vi "DCSource.vi"() -> ()   [LabVIEW 2014]
uses:
  <vilib>/Instr/_visa.llb/VISA Set IO Buffer Mask.ctl
  <vilib>/Utility/miscctls.llb/LVRowAndColumnTypeDef.ctl
  <vilib>/Instr/_visa.llb/VISA Configure Serial Port (Instr).vi
  <vilib>/Utility/file.llb/Write To Spreadsheet File (string).vi
  <vilib>/Utility/file.llb/Read From Spreadsheet File (string).vi
panel:
  in  "shutDown":bool
  in  "本机表格":string[][](table)=[["0.000"], ["0.000"], ["0.000"], ["0.000"], ["0.000"], ["0.000"], ["0.000"], ["0.000"]]
  in  "result_Tab":enum32{"输出控制", "电能校验", "误差计算", "潜动启动", "无"}(tab)
  in  "outPut_form":string[][](table)=[["0.000"], ["0.000"], ["0.000"], ["0.000"], ["0.000"], ["0.000"], ["0.000"], ["0.000"]]
  in  "电能显示表":string[][](table)=[["", "", "", "", "", ""], ["", "", "", "", "", ""], ["", "", "", "", "", ""], ["", "", "", "", "", ""], ["", "", "", "", "", ""], ["", "", "", "", "", ""], ["", "", "", "", "", ""], ["", "", "", "", "", ""], ["", "", "", "", "", ""], ["", "", "", "", "", ""], ["", "", "", "", "", ""], ["", "", "", "", "", ""], ["", "", "", "", "", ""], ["", "", "", "", "", ""], ["", "", "", "", "", ""]]
  in  "误差显示表":string[][](table)=[["", "", "", "", "", ""], ["", "", "", "", "", ""], ["", "", "", "", "", ""], ["", "", "", "", "", ""], ["", "", "", "", "", ""], ["", "", "", "", "", ""], ["", "", "", "", "", ""], ["", "", "", "", "", ""], ["", "", "", "", "", ""], ["", "", "", "", "", ""], ["", "", "", "", "", ""], ["", "", "", "", "", ""], ["", "", "", "", "", ""], ["", "", "", "", "", ""], ["", "", "", "", "", ""]]
  out "单点显示表":string[][](table)
  in  "All输出":cluster{"A停止":bool, "A启动":bool}
  in  "超时记录":bool[](array[boolean])=[FALSE, FALSE, FALSE]
  out "当前功率":dbl
  out "表3已等待时间":dbl
  out "表2已等待时间":dbl
  out "表1已等待时间":dbl
  in  "表1OK":bool
  in  "表2OK":bool
  in  "表3OK":bool
  in  "已用秒数":dbl
  out "计时状态":bool
  out "E检定行":i32
  out "下一点":bool
  out "UI行数":i32
  out "E行数":i32
  in  "UI当前行":i32
  out "检定状态":bool
  in  "E当前行":i32
  in  "软键盘":bool caption="Ia停止"
  out "提示信息":bool
  in  "控制选项卡":T1(tab)
  in  "vOptios_Tab":enum32{"电流1", "电流2", "电流3", "电流4"}(tab)
  in  "I操作":T2
  in  "I纹波":sgl caption="电流纹波(A)" min=0 max=20 format="%.3f"
  out "I状态":bool caption="状态"
  in  "I幅值":sgl=1.0 caption="电流(A)" min=0 max=200 format="%.3f"
  in  "I档位":u32(ring)=85 caption="电流档位" items=["自动"=85, "0.02A"=0, "0.2A"=1, "1A"=2, "5A"=3, "10A"=4, "20A"=5, "30A"=6, "60A"=7, "200A"=8]
  in  "UB_outPut_ctl":T3
  out "UB_status":bool caption="状态"
  in  "UB_Pos":u32(ring)=85 caption="电流档位" items=["自动"=85, "0.01V"=0, "0.1V"=1, "0.5"=2, "5V"=3]
  in  "UB_amplitude":sgl=48.0 caption="电流(A)" min=0 max=10 format="%.3f"
  in  "UB_ripple":sgl caption="电流纹波(A)" min=0 max=100 format="%.3f"
  in  "IB_outPut_ctl":T4
  in  "IB_pos":u32(ring)=85 caption="电流档位" items=["自动"=85, "0.01V"=0, "0.1V"=1, "0.5V"=2, "5V"=3]
  in  "IB_amplitude":sgl=1.0 caption="电流(A)" min=0 max=200 format="%.3f"
  out "IB_status":bool caption="状态"
  in  "IB_ripple":sgl caption="电流纹波(A)" min=0 max=20 format="%.3f"
  in  "UC_outPut_ctl":T5
  in  "UC_ripple":sgl caption="电流纹波(A)" min=0 max=20 format="%.3f"
  out "UC_status":bool caption="状态"
  in  "UC_amplitude":sgl=1.0 caption="电流(A)" min=0 max=200 format="%.3f"
  in  "UC_pos":u32(ring)=85 caption="电流档位" items=["自动"=85, "0.01"=0, "0.1V"=1, "0.5V"=2, "5V"=3]
  in  "U档位":u32(ring)=85 caption="电压档位" items=["自动"=85, "65V"=0, "250V"=1, "500V"=2, "750V"=3, "1000V"=4]
  in  "U频率":sgl caption="纹波频率(Hz)" min=0 max=1000 format="%.3f"
  in  "U纹波":sgl caption="电压纹波(V)" min=0 max=100 format="%.3f"
  out "U状态":bool caption="状态"
  in  "U幅值":sgl=48.0 caption="电压(V)" min=0 max=1000 format="%.3f"
  in  "U操作":T6
  in  "电能检定通道":u16(ring) items=["电流 1", "电流 2", "电流 3", "电流 4"]
  in  "表3超时时间":string
  in  "表2超时时间":string
  in  "表1超时时间":string
  in  "E检定表格":string[][](table)=[["", "", "", "", ""], ["", "", "", "", ""], ["", "", "", "", ""], ["", "", "", "", ""], ["", "", "", "", ""]]
  in  "E检定操作":T7
  in  "E检定参数":T8={"额定电压"=48.0, "U检定点"=100.0, "标定电流"=20.0, "I检定点"=100.0, "允许误差"=0.5, "I检定点 2"=10.0} {"标定电流" min=0 max=200; "额定电压" min=0 max=1000}
  in  "E增删改清":T9
  in  "表1":bool
  in  "表2":bool
  in  "表3":bool
  in  "增加等待时间(s)":dbl=4.0
  in  "UI检定表格":string[][](table) caption="默认电压误差表"
  in  "UI检定操作":T10
  in  "UI增删改清":T9
  in  "UI检定参数":T11={"检定项目"=0, "额定电压"=48.0, "电压检定点"=20.0, "标定电流"=100.0, "电流检定点"=100.0, "误差限值"=0.5, "电压纹波"=0.0, "电流纹波"=0.0, "纹波频率"=0.0} {"标定电流" min=0 max=200; "额定电压" min=0 max=1000; "检定项目" items=["电压误差", "电流误差", "纹波试验"]}
  in  "误差电流通道":u16(ring) items=["电流 1", "电流 2", "电流 3", "电流 4"]
  in  "潜启电流通道":u16(ring) items=["电流 1", "电流 2", "电流 3", "电流 4"]
  in  "潜动起动":T12={"已用时间"="", "开始试验"=FALSE, "测试时间"=20.0, "标定电流"=20.0, "额定电压"=48.0, "试验项目"=0, "U检定点"=130.0, "I检定点"=0.1, "脉冲数"=1} {"脉冲数" max=200; "试验项目" items=["潜动试验", "起动试验"]; "额定电压" min=0 max=1000; "标定电流" min=0 max=200; "测试时间" format="%#.3f"}
  out "试验结果":string[](array[string])
  in  "生成报表":bool
  in  "报表名称":string
  in  "报表选项":u16(ring) items=["按时间命名", "自定义命名"]
  in  "小信号变比(A/1mv)":cluster{"电流2":sgl, "电流3":sgl, "电流4":sgl}={"电流2"=200.0, "电流3"=200.0, "电流4"=200.0}
  in  "脉冲输入口":u8(ring) items=["端口1", "端口2", "端口3"]
  in  "本机表参数":cluster{"有功常数":i32, "无功常数":i32, "输出类型":i32}={"有功常数"=200, "无功常数"=200, "输出类型"=0} {"输出类型" items=["有功脉冲", "无功脉冲"]}
  in  "电能表参数":T13={"有功常数"=200, "无功常数"=200, "校验圈数"=5, "校验类型"=0, "S值计算次数"=12, "S值计算方法"=0} {"S值计算方法" items=["平均值法"]; "校验类型" items=["有功脉冲", "无功脉冲"]}
  in  "本机表设置":cluster{"本机读参数":bool, "本机写参数":bool}
  in  "电能表设置":cluster{"表读参数":bool, "表写参数":bool}
  in  "串口信息":T14={"串口号"="COM1", "波特率"=57600, "校验位"=0, "停止位"=10} {"停止位" items=["1位"=10, "1.5位"=15, "2位"=20]; "校验位" items=["无校验", "奇校验", "偶检验"]; "波特率" items=["9600"=9600, "38400"=38400, "57600"=57600]}
  in  "串口连接":bool
  out "串口灯":bool
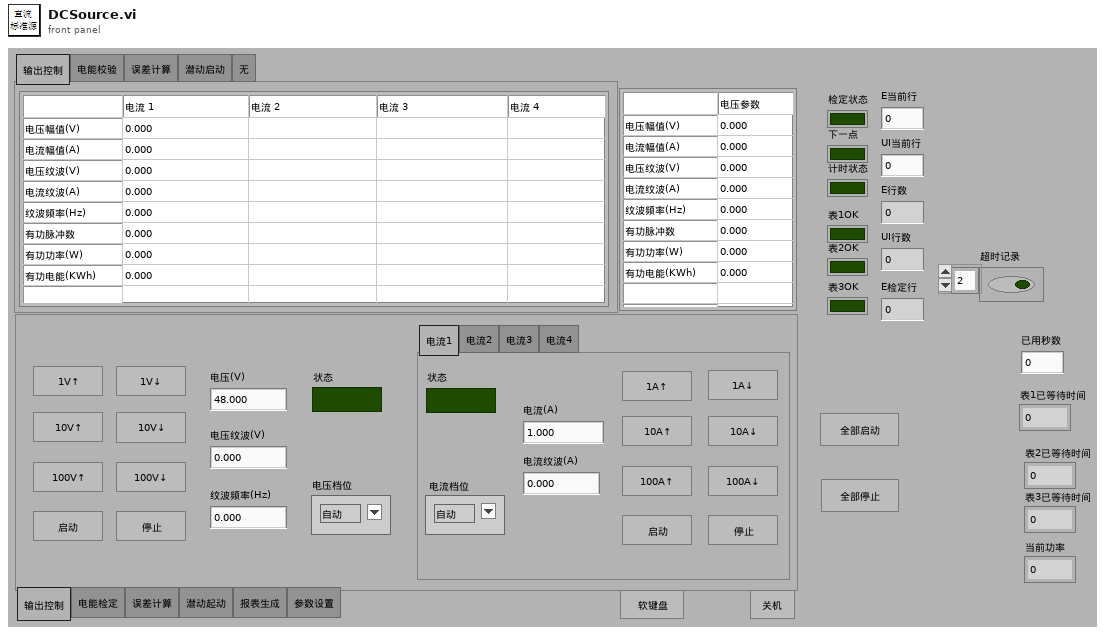
[diagram p1: front panel]
types:
  T1 = enum32{"输出控制", "电能检定", "误差计算", "潜动起动", "报表生成", "参数设置"}
  T2 = cluster{"ISub100":bool, "IAdd100":bool, "ISub10":bool, "IAdd10":bool, "ISub1":bool, "IAdd1":bool, "I启动":bool, "I停止":bool}
  T3 = cluster{"UB_outPut_start":bool, "UB_outPut_stop":bool}
  T4 = cluster{"IB_outPut_start":bool, "IB_outPut_stop":bool}
  T5 = cluster{"UC_outPut_stop":bool, "UC_outPut_start":bool}
  T6 = cluster{"UAdd10":bool, "USub10":bool, "UAdd100":bool, "USub100":bool, "U停止":bool, "USub1":bool, "UAdd1":bool, "U启动":bool}
  T7 = cluster{"开始检定":bool, "单点检定":bool, "保存方案":bool, "导入方案":bool}
  T8 = cluster{"额定电压":sgl, "U检定点":sgl, "标定电流":sgl, "I检定点":sgl, "允许误差":sgl, "I检定点 2":sgl}
  T9 = cluster{"插入":bool, "编辑":bool, "删除":bool, "清空":bool}
  T10 = cluster{"输出开关":bool, "保存方案":bool, "导入方案":bool, "计算误差":bool}
  T11 = cluster{"检定项目":u16, "额定电压":sgl, "电压检定点":sgl, "标定电流":sgl, "电流检定点":sgl, "误差限值":sgl, "电压纹波":sgl, "电流纹波":sgl, "纹波频率":sgl}
  T12 = cluster{"已用时间":string, "开始试验":bool, "测试时间":dbl, "标定电流":sgl, "额定电压":sgl, "试验项目":u16, "U检定点":sgl, "I检定点":sgl, "脉冲数":u32}
  T13 = cluster{"有功常数":i32, "无功常数":i32, "校验圈数":i32, "校验类型":i32, "S值计算次数":i32, "S值计算方法":i32}
  T14 = cluster{"串口号":refnum<visa-resource-name>, "波特率":u32, "校验位":u8, "停止位":u16}
  T15 = cluster{"串口号":refnum<visa-resource-name>, "波特率":u16, "校验位":u16, "停止位":u16}
  T16 = cluster{"有功功率":sgl, "有功电能":sgl, "有功脉冲":u64, "标准偏差值":sgl[], "电能误差":sgl[], "脉冲输入功率":sgl[], "脉冲电能累计":sgl[], "输入脉冲数":sgl[]}
  T17 = typedef "LVRowAndColumnTypeDef.ctl" = cluster{"Row":i32, "Column":i32}
  T18 = cluster{"有功常数":i32, "无功常数":i32, "校验圈数":i32, "校验类型":i32, "S值计算次数":i32, "S值计算方法":i32}[]
  T19 = enum8{"Enabled", "Disabled", "Disabled and Grayed Out"}
  T20 = typedef "VISA Set IO Buffer Mask.ctl" = u16
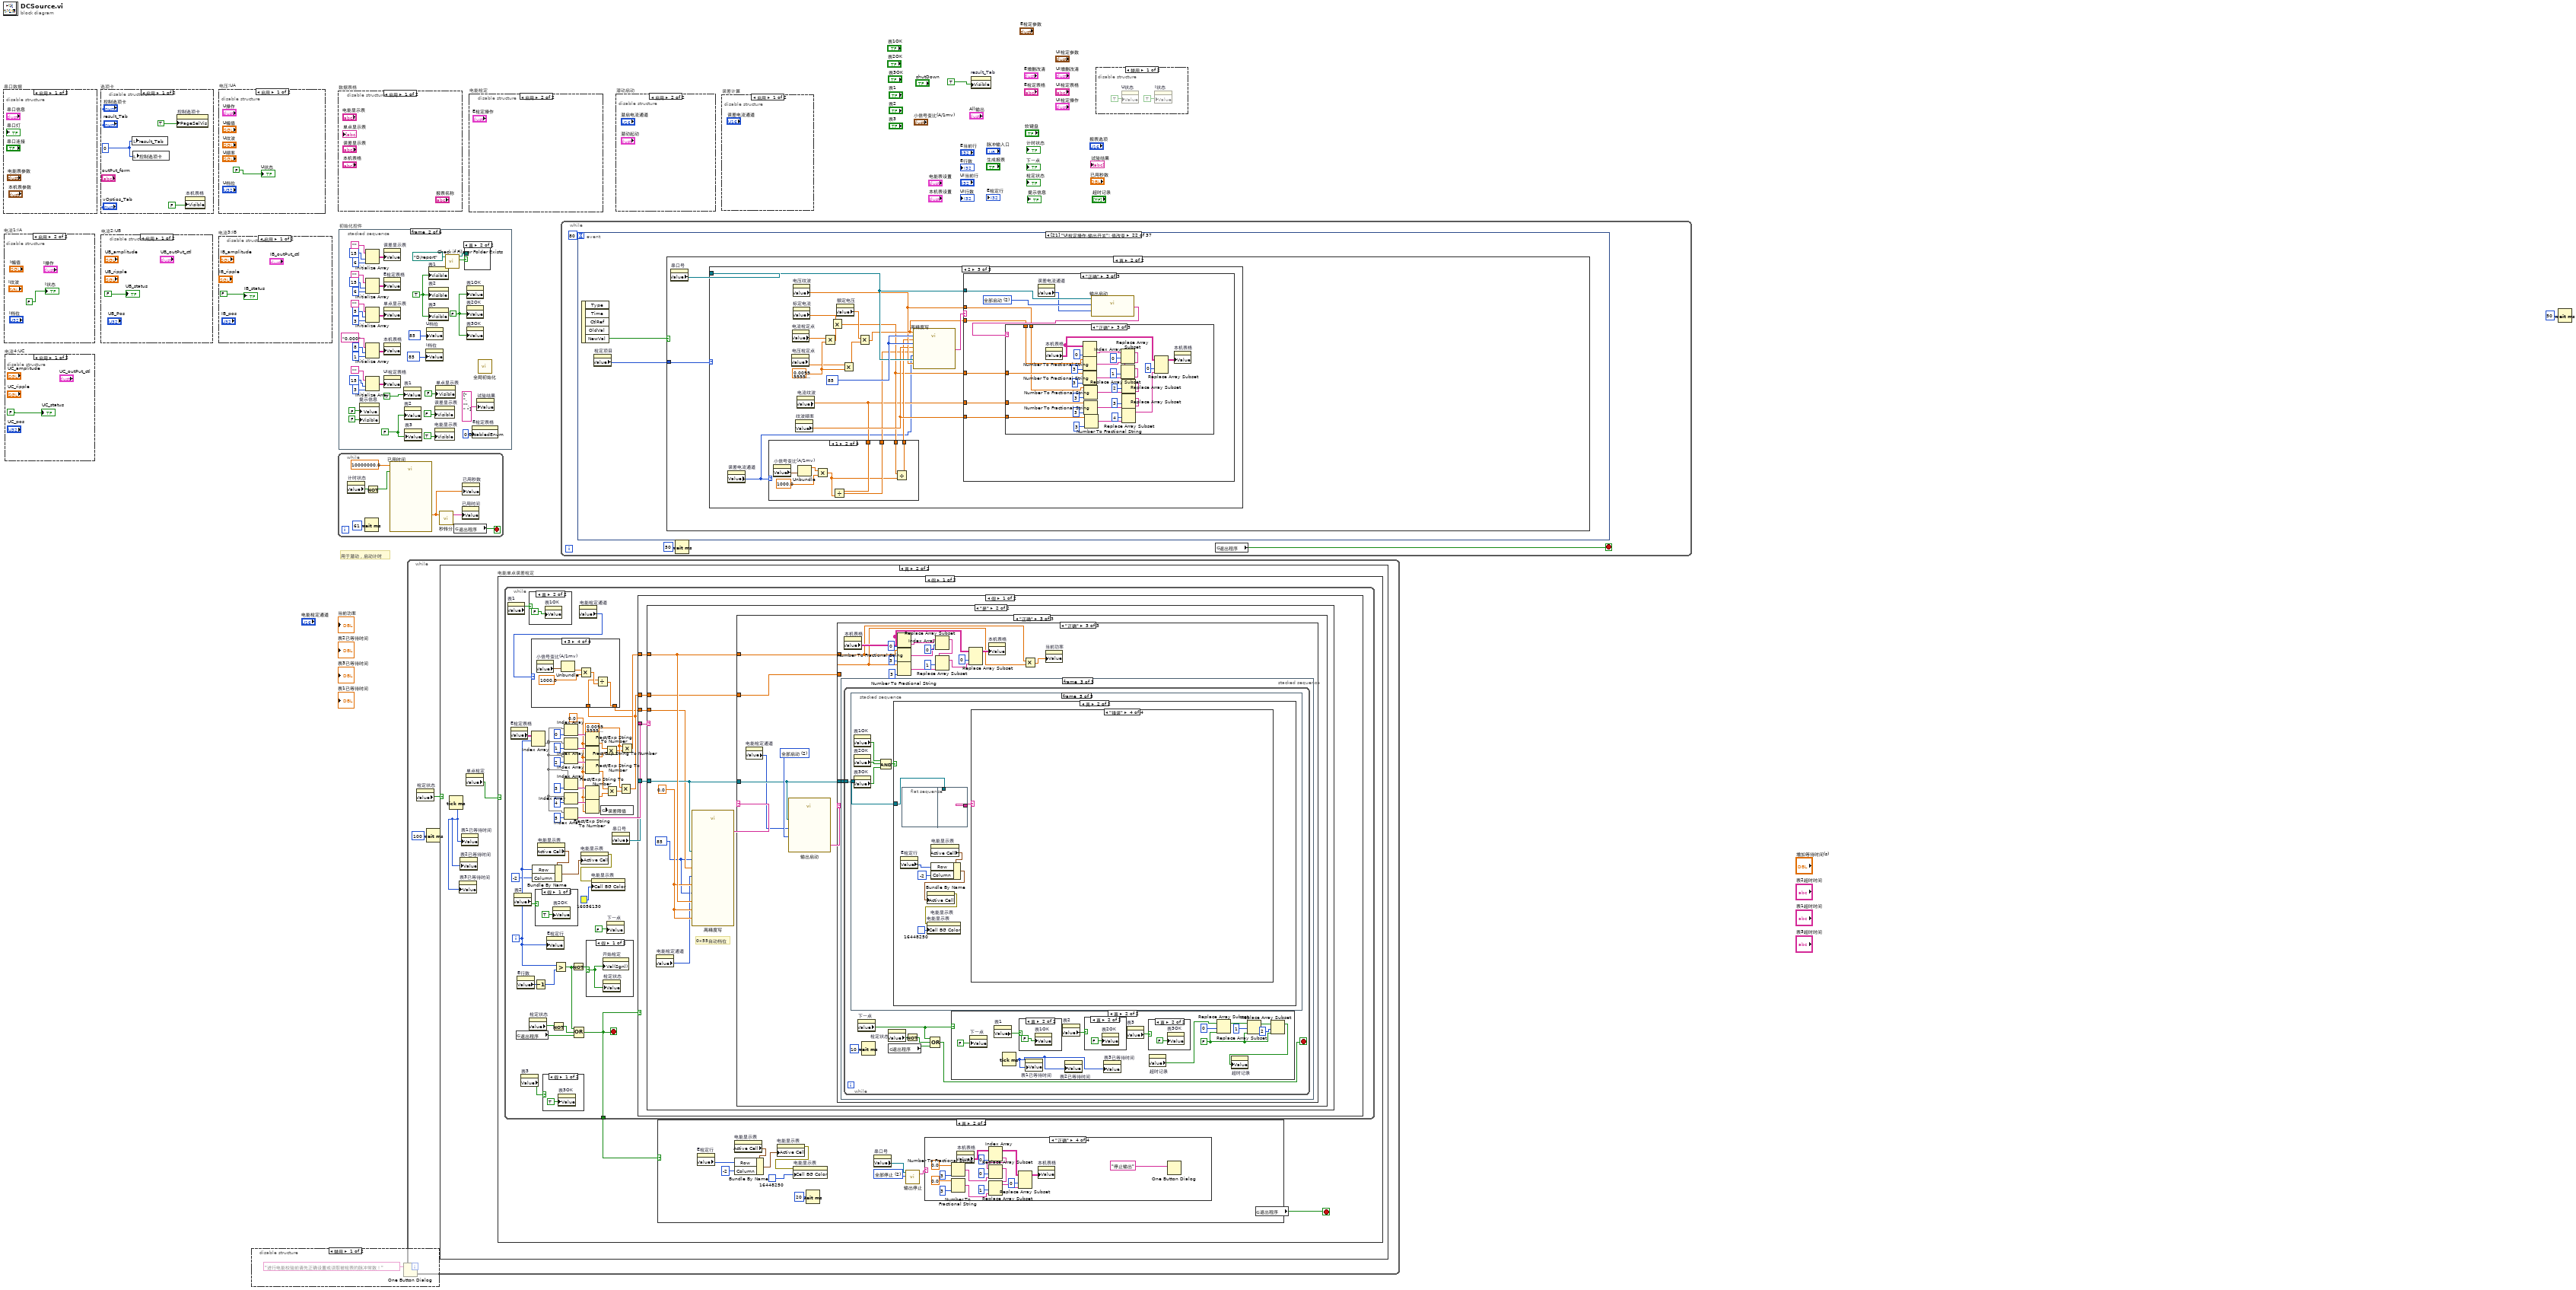
[diagram p0: block diagram]
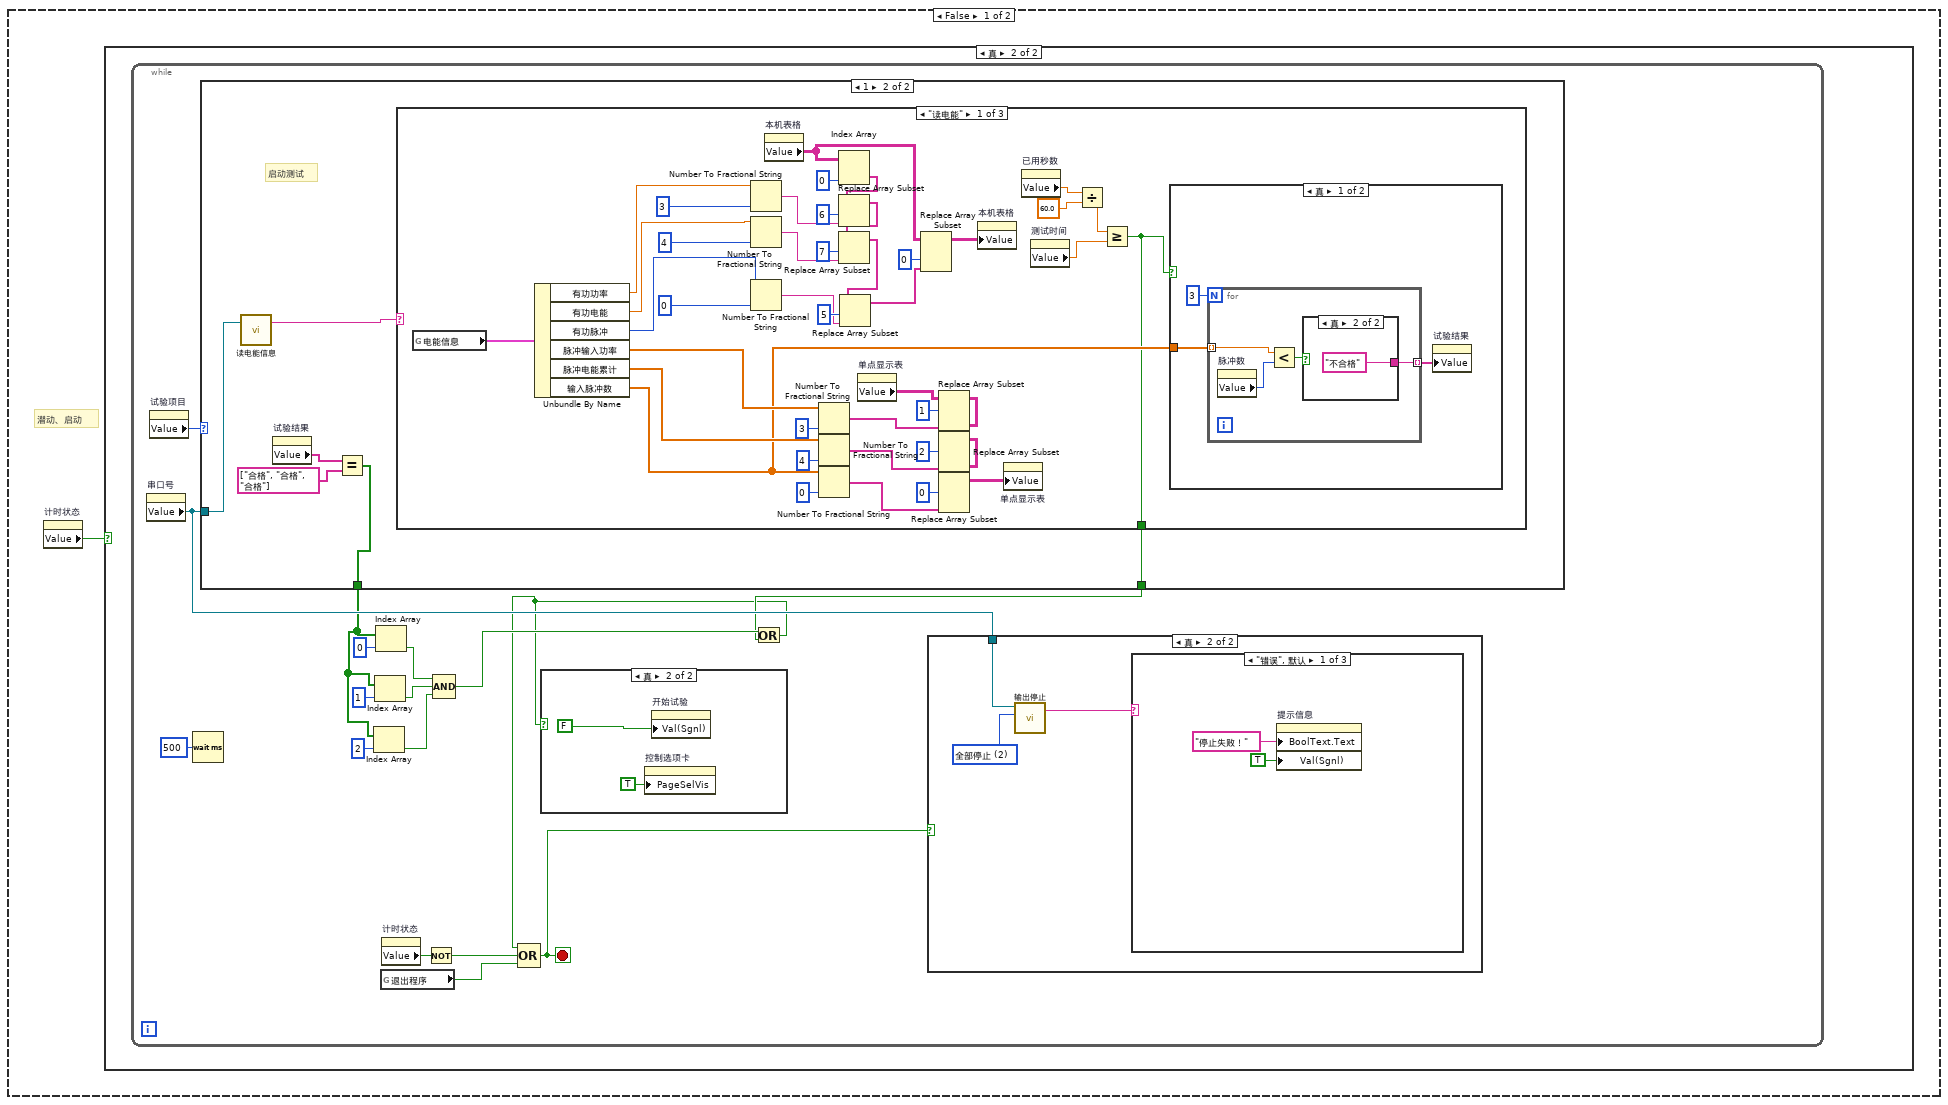
[diagram p15: hidden frame]
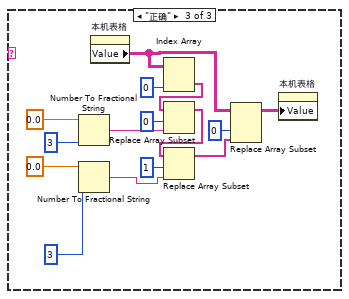
[diagram p20: hidden frame]
diagram:
  # "用于潜动，启动计时"
  n1 = disable-structure "串口数据" shown="启用" {
    frame Enabled {
    }
    frame Disabled {
    }
  }
  n2 = disable-structure "电流1:IA" shown="启用" {
    frame Disabled {
    }
    frame Enabled {
      "I状态" <- FALSE
    }
  }
  n3 = disable-structure "电流4:UC" shown="启用" {
    frame Enabled {
      "UC_status" <- FALSE
    }
    frame Disabled {
    }
  }
  n4 = disable-structure "选项卡" shown="启用" {
    frame Enabled {
      w6 = 0
      n5 = local write "result_Tab"(w6) -> ()
      n6 = local write "控制选项卡"(w6) -> ()
      n7 = property on="控制选项卡" class="TabCtl (严格)"("PageSelVis"=TRUE ("页选择器可见")) -> ()  [unwired: 2 in, 2 out]
      n8 = property on="本机表格" class="Tbl (严格)"("Visible"=FALSE) -> ()  [unwired: 2 in, 2 out]
    }
    frame Disabled {
    }
  }
  n9 = disable-structure "电流2:UB" shown="启用" {
    frame Enabled {
      "UB_status" <- FALSE
    }
    frame Disabled {
    }
  }
  n10 = disable-structure "电流3:IB" shown="启用" {
    frame Enabled {
      "IB_status" <- FALSE
    }
    frame Disabled {
    }
  }
  n11 = disable-structure "电压:UA" shown="启用" {
    frame Enabled {
      "U状态" <- FALSE
    }
    frame Disabled {
    }
  }
  n12 = disable-structure shown="禁用" {
    frame Disabled {
      n13 = One Button Dialog(message="进行电能校验前请先正确设置或读取被检表的脉冲常数！" ("消息")) -> ()  [unwired: 1 in, 1 out]
    }
    frame Enabled {
    }
  }
  n14 = disable-structure "数据表格" shown="启用" {
    frame Enabled {
    }
    frame Disabled {
    }
  }
  n15 = while {
    stop <- w12 stop-if-true
    n16 = property on="计时状态" class="Bool (严格)"() -> ("Value"=w16:bool)  [unwired: 2 in, 2 out]
    n17 = Wait (ms)(milliseconds to wait=u32 61 ("等待时间（毫秒）")) -> ()  [unwired: 1 out]
    n18 = Not(x=w16) -> (.not. x?=w15:bool)
    n19 = call "已用时间"("Time Target (s)"=10000000.0, "Reset"=w15) -> ("Elapsed Time (s)"=w13:dbl)  [unwired: 10 in, 7 out]
    n20 = call "秒转分.vi"("秒计数"=w13) -> ("分钟数"=w14:string)  [unwired: 2 in]
    n21 = global read "系统全局.vi" "退出程序"() -> (w12:bool)
    n22 = property on="已用时间" class="Str"("Value"=w14) -> ()  [unwired: 2 in, 2 out]
    n23 = property on="已用秒数" class="DigNum (严格)"("Value"=w13) -> ()  [unwired: 2 in, 2 out]
  }
  n24 = stacked-sequence "初始化控件" {
    frame #0 {
      n25 = property on="保存方案" class="Bool (严格)"("DisabledEnum"=0) -> ()  [unwired: 2 in, 2 out]
      n26 = property on="导入方案" class="Bool (严格)"("DisabledEnum"=0) -> ()  [unwired: 2 in, 2 out]
      n27 = property on="额定电压" class="DigNum (严格)"("DisabledEnum"=0) -> ()  [unwired: 2 in, 2 out]
      n28 = property on="标定电流" class="DigNum (严格)"("DisabledEnum"=3) -> ()  [unwired: 2 in, 2 out]
      n29 = property on="误差限值" class="DigNum (严格)"("DisabledEnum"=0) -> ()  [unwired: 2 in, 2 out]
      n30 = property on="电压纹波" class="DigNum (严格)"("DisabledEnum"=3) -> ()  [unwired: 2 in, 2 out]
      n31 = property on="电流纹波" class="DigNum (严格)"("DisabledEnum"=3) -> ()  [unwired: 2 in, 2 out]
      n32 = property on="纹波频率" class="DigNum (严格)"("DisabledEnum"=3) -> ()  [unwired: 2 in, 2 out]
      n33 = property on="报表名称" class="Str"("DisabledEnum"=3) -> ()  [unwired: 2 in, 2 out]
      n34 = property on="电压检定点" class="DigNum (严格)"("DisabledEnum"=0) -> ()  [unwired: 2 in, 2 out]
      n35 = property on="电流检定点" class="DigNum (严格)"("DisabledEnum"=3) -> ()  [unwired: 2 in, 2 out]
      n36 = property on="UI检定表格" class="Tbl (严格)"("DisabledEnum"=0) -> ()  [unwired: 2 in, 2 out]
      n37 = property on="UI增删改清" class="Clust (严格)"("DisabledEnum"=0) -> ()  [unwired: 2 in, 2 out]
      n38 = property on="输出开关" class="Bool (严格)"("DisabledEnum"=0) -> ()  [unwired: 2 in, 2 out]
      n39 = property on="串口信息" class="Clust (严格)"("DisabledEnum"=0) -> ()  [unwired: 2 in, 2 out]
      n40 = property on="标定电流" class="DigNum (严格)"("DisabledEnum"=3) -> ()  [unwired: 2 in, 2 out]
      n41 = property on="I检定点" class="DigNum (严格)"("DisabledEnum"=3) -> ()  [unwired: 2 in, 2 out]
      n42 = property on="U状态" class="Bool (严格)"("Value"=FALSE ("输出状态")) -> ()  [unwired: 2 in, 2 out]
      n43 = property on="I状态" class="Bool (严格)"("Value"=FALSE ("输出状态")) -> ()  [unwired: 2 in, 2 out]
      n44 = property on="下一点" class="Bool (严格)"("Value"=FALSE ("下一点")) -> ()  [unwired: 2 in, 2 out]
      n45 = property on="检定状态" class="Bool (严格)"("Value"=FALSE ("检定状态")) -> ()  [unwired: 2 in, 2 out]
      n46 = property on="单点检定" class="Bool (严格)"("Value"=FALSE ("检定状态")) -> ()  [unwired: 2 in, 2 out]
      n47 = property on="开始检定" class="Bool (严格)"("Value"=FALSE ("检定状态")) -> ()  [unwired: 2 in, 2 out]
      n48 = property on="串口灯" class="Bool (严格)"("Value"=FALSE ("串口灯")) -> ()  [unwired: 2 in, 2 out]
      n49 = property on="串口连接" class="Bool (严格)"("Value"=FALSE ("串口灯")) -> ()  [unwired: 2 in, 2 out]
      n50 = property on="脉冲数" class="DigNum (严格)"("Value"=u32 1 ("值")) -> ()  [unwired: 2 in, 2 out]
      n51 = property on="E当前行" class="DigNum (严格)"("Value"=0 ("当前行")) -> ()  [unwired: 2 in, 2 out]
      n52 = property on="UI当前行" class="DigNum (严格)"("Value"=0 ("当前行")) -> ()  [unwired: 2 in, 2 out]
      n53 = property on="U频率" class="DigNum (严格)"("Value"=sgl 0.0 ("U频率")) -> ()  [unwired: 2 in, 2 out]
      n54 = property on="检定项目" class="Ring (严格)"("Value"=u16 0 ("值")) -> ()  [unwired: 2 in, 2 out]
      n55 = property on="E检定行" class="DigNum (严格)"("Value"=0 ("E检定行")) -> ()  [unwired: 2 in, 2 out]
      n56 = property on="E行数" class="DigNum (严格)"("Value"=0 ("E行数")) -> ()  [unwired: 2 in, 2 out]
      n57 = property on="UI行数" class="DigNum (严格)"("Value"=0 ("UI行数")) -> ()  [unwired: 2 in, 2 out]
      n58 = property on="试验项目" class="Ring (严格)"("Value"=u16 0 ("值")) -> ()  [unwired: 2 in, 2 out]
      n59 = property on="报表选项" class="Ring (严格)"("Value"=u16 0) -> ()  [unwired: 2 in, 2 out]
    }
    frame #1 {
      w55 = FALSE
      w56 = TRUE ("表2OK")
      w58 = FALSE ("表2OK")
      n60 = property on="提示信息" class="Bool (严格)"("Value"=FALSE ("提示信息"), "Visible"=FALSE ("可见")) -> ()  [unwired: 2 in, 2 out]
      n61 = Initialize Array("", 15 ("维数大小"), 6 ("维数大小")) -> (w87:string[][])
      n62 = Initialize Array("", 15 ("维数大小"), 6 ("维数大小")) -> (w82:string[][])
      n63 = Initialize Array("", 5 ("维数大小"), 3 ("维数大小")) -> (w78:string[][])
      n64 = Initialize Array("0.000" ("元素"), 8 ("维数大小"), 1 ("维数大小")) -> (w77:string[][])
      n65 = Initialize Array("", 15 ("维数大小"), 3 ("维数大小")) -> (w73:string[][])
      n66 = property on="误差显示表" class="Tbl (严格)"("Value"=w87) -> ()  [unwired: 2 in, 2 out]
      n67 = property on="E检定表格" class="Tbl (严格)"("Value"=w82) -> ()  [unwired: 2 in, 2 out]
      n68 = property on="单点显示表" class="Tbl (严格)"("Value"=w78) -> ()  [unwired: 2 in, 2 out]
      n69 = property on="本机表格" class="Tbl (严格)"("Value"=w77) -> ()  [unwired: 2 in, 2 out]
      n70 = property on="UI检定表格" class="Tbl (严格)"("Value"=w73) -> ()  [unwired: 2 in, 2 out]
      n71 = property on="表1" class="Bool (严格)"("Value"=TRUE) -> ()  [unwired: 2 in, 2 out]
      n72 = property on="表2" class="Bool (严格)"("Value"=w55) -> ()  [unwired: 2 in, 2 out]
      n73 = property on="表3" class="Bool (严格)"("Value"=w55) -> ()  [unwired: 2 in, 2 out]
      n74 = property on="I档位" class="Ring (严格)"("Value"=u32 85 ("电流档位")) -> ()  [unwired: 2 in, 2 out]
      n75 = property on="U档位" class="Ring (严格)"("Value"=u32 85 ("电流档位")) -> ()  [unwired: 2 in, 2 out]
      n76 = property on="表1" class="Bool (严格)"("Visible"=w56) -> ()  [unwired: 2 in, 2 out]
      n77 = property on="表2" class="Bool (严格)"("Visible"=w56) -> ()  [unwired: 2 in, 2 out]
      n78 = property on="表3" class="Bool (严格)"("Visible"=w56) -> ()  [unwired: 2 in, 2 out]
      n79 = property on="误差显示表" class="Tbl (严格)"("Visible"=FALSE ("可见")) -> ()  [unwired: 2 in, 2 out]
      n80 = property on="电能显示表" class="Tbl (严格)"("Visible"=TRUE ("可见")) -> ()  [unwired: 2 in, 2 out]
      n81 = property on="单点显示表" class="Tbl (严格)"("Visible"=FALSE ("可见")) -> ()  [unwired: 2 in, 2 out]
      n82 = call <vilib>:"Check if File or Folder Exists.vi"("path"=path "D:/report" ("路径（使用对话框）")) -> ("file or folder exists?"=w68:bool, "dup path"=w67:path)  [unwired: 8 in, 1 out]
      n83 = case shown="真" w68 {
        tunnel: w67 -> [w90 _]
        frame False {
          n84 = Create Folder(path (use dialog)=w90) -> ()  [unwired: 2 in, 3 out]
        }
        frame True {
        }
      }
      n85 = property on="表1OK" class="Bool (严格)"("Value"=w58) -> ()  [unwired: 2 in, 2 out]
      n86 = property on="表2OK" class="Bool (严格)"("Value"=w58) -> ()  [unwired: 2 in, 2 out]
      n87 = property on="表3OK" class="Bool (严格)"("Value"=w58) -> ()  [unwired: 2 in, 2 out]
      n88 = property on="E检定表格" class="Tbl (严格)"("DisabledEnum"=0) -> ()  [unwired: 2 in, 2 out]
      n89 = property on="试验结果" class="Arr (严格)"("Value"=string[] [" ", "", " "] ("试验结果")) -> ()  [unwired: 2 in, 2 out]
      n90 = call "全局初始化.vi"() -> ()  [unwired: 12 in]
    }
    frame #2 {
      n91 = property on="U幅值" class="DigNum (严格)"() -> ("Maximum"=w98:dbl)  [unwired: 2 in, 2 out]
      n92 = property on="I幅值" class="DigNum (严格)"() -> ("Maximum"=w97:dbl)  [unwired: 2 in, 2 out]
      n93 = property on="U幅值" class="DigNum (严格)"("Maximum"=sgl 1000.0 ("数据输入界限:最大值"), "Minimum"=0.0 ("数据输入界限:最小值")) -> ()  [unwired: 2 in, 2 out]
      n94 = property on="I幅值" class="DigNum (严格)"("Maximum"=sgl 200.0 ("数据输入界限:最大值"), "Minimum"=0.0 ("数据输入界限:最小值")) -> ()  [unwired: 2 in, 2 out]
      n95 = Multiply(x=w98, y=0.1) -> (x*y=w100:dbl)
      n96 = Multiply(x=w97, y=0.1) -> (x*y=w95:dbl)
      n97 = property on="U纹波" class="DigNum (严格)"("Maximum"=w100) -> ()  [unwired: 2 in, 2 out]
      n98 = property on="I纹波" class="DigNum (严格)"("Maximum"=w95) -> ()  [unwired: 2 in, 2 out]
    }
    frame #3 {
      n99 = disable-structure shown="启用" {
        frame Enabled {
          n100 = Current VI's Path() -> (path=w105:path)
          n101 = Strip Path(path=w105) -> (stripped path=w104:path)  [unwired: 1 out]
          n102 = Strip Path(path=w104) -> (stripped path=w108:path)  [unwired: 1 out]
          n103 = Build Path(base path=w108, name or relative path="table\\默认电压误差表" ("名称或相对路径")) -> (appended path=w107:path)
          n104 = Build Path(base path=w108, name or relative path="table\\默认电能检定表" ("名称或相对路径")) -> (appended path=w106:path)
          n105 = call-poly <vilib>:"Read From Spreadsheet File.vi"("file path (dialog if empty)"=w107) -> ("all rows"=w112:string[][])  [unwired: 6 in, 4 out]
          n106 = call-poly <vilib>:"Read From Spreadsheet File.vi"("file path (dialog if empty)"=w106) -> ("all rows"=w111:string[][])  [unwired: 6 in, 4 out]
          n107 = property on="UI检定表格" class="Tbl (严格)"("Value"=w112) -> ()  [unwired: 2 in, 2 out]
          n108 = property on="E检定表格" class="Tbl (严格)"("Value"=w111) -> ()  [unwired: 2 in, 2 out]
        }
        frame Disabled {
        }
      }
      n109 = property on="本机表参数" class="Clust (严格)"("Value"=cluster{"有功常数":i32, "无功常数":i32, "输出类型":i32} {"有功常数"=200, "无功常数"=200, "输出类型"=0} ("本机表参数")) -> ()  [unwired: 2 in, 2 out]
      n110 = property on="电能表参数" class="Clust (严格)"("Value"=T13 {"有功常数"=200, "无功常数"=200, "校验圈数"=5, "校验类型"=0, "S值计算次数"=12, "S值计算方法"=0} ("电能表参数")) -> ()  [unwired: 2 in, 2 out]
      n111 = local write "串口信息"(T15 {"串口号"="COM1", "波特率"=57600, "校验位"=0, "停止位"=10} ("串口信息")) -> ()
    }
    frame #4 {
      n112 = property on="串口连接" class="Bool (严格)"("Val(Sgnl)"=TRUE ("值(信号)")) -> ()  [unwired: 2 in, 2 out]
      n113 = property on="误差显示表" class="Tbl (严格)"("Column Headers[]"=string[] ["表1电能(KWh)", "误差(%)", "表2电能(KWh)", "误差(%)", "表3电能(KWh)", "误差(%)"] ("列首字符串[]")) -> ()  [unwired: 2 in, 2 out]
      n114 = property on="本机表格" class="Tbl (严格)"("Row Headers[]"=string[] ["电压幅值(V)", "电流幅值(A)", "电压纹波(V)", "电流纹波(A)", "纹波频率(Hz)", "有功脉冲数", "有功功率(W)", "有功电能(KWh)"] ("列首字符串[]")) -> ()  [unwired: 2 in, 2 out]
      n115 = property on="误差显示表" class="Tbl (严格)"("Row Headers[]"=string[] [] ("行首字符串[]")) -> ()  [unwired: 2 in, 2 out]
      n116 = property on="UI检定表格" class="Tbl (严格)"("Column Headers[]"=string[] ["电压幅值(V)", "检定点(%)", "误差限值(%)"] ("列首字符串[]")) -> ()  [unwired: 2 in, 2 out]
      n117 = property on="E检定表格" class="Tbl (严格)"("Column Headers[]"=string[] ["额定电压(V)", "检定点(%)", "标定电流(A)", "检定点(%)", "允许误差(%)", "是否检定"] ("行首字符串[]")) -> ()  [unwired: 2 in, 2 out]
      n118 = property on="本机表格" class="Tbl (严格)"("Column Headers[]"=string[] ["电压参数"] ("列首字符串[]")) -> ()  [unwired: 2 in, 2 out]
    }
    frame #5 {
      w120 = 1
      n119 = Initialize Array("0.000" ("元素"), 8 ("维数大小"), 4 ("维数大小")) -> (w123:string[][])
      n120 = property on="outPut_form" class="Tbl (严格)"("Column Headers[]"=string[] ["电流 1", "电流 2", "电流 3", "电流 4"]) -> ()  [unwired: 2 in, 2 out]
      n121 = property on="outPut_form" class="Tbl (严格)"("Value"=w123) -> ()  [unwired: 2 in, 2 out]
      n122 = property on="outPut_form" class="Tbl (严格)"("Row Headers[]"=string[] ["电压幅值(V)", "电流幅值(A)", "电压纹波(V)", "电流纹波(A)", "纹波频率(Hz)", "有功脉冲数", "有功功率(W)", "有功电能(KWh)"] ("列首字符串[]")) -> ()  [unwired: 2 in, 2 out]
      n123 = local write "小信号变比(A/1mv)"(cluster{"有功常数":i32, "无功常数":i32, "输出类型":i32} {"有功常数"=0, "无功常数"=0, "输出类型"=0} ("本机表参数")) -> ()
      n124 = property on="outPut_form" class="Tbl (严格)"("AutoRowHt"=TRUE) -> ()  [unwired: 2 in, 2 out]
      n125 = property on="UB_amplitude" class="DigNum (严格)"("Value"=w120) -> ()  [unwired: 2 in, 2 out]
      n126 = property on="UC_amplitude" class="DigNum (严格)"("Value"=w120) -> ()  [unwired: 2 in, 2 out]
      n127 = property on="IB_amplitude" class="DigNum (严格)"("Value"=w120) -> ()  [unwired: 2 in, 2 out]
    }
  }
  n128 = while {
    stop <- w129 stop-if-true
    n129 = property on="检定状态" class="Bool (严格)"() -> ("Value"=w131:bool)  [unwired: 2 in, 2 out]
    n130 = Wait (ms)(milliseconds to wait=u32 100 ("等待时间（毫秒）")) -> ()  [unwired: 1 out]
    n131 = case shown="真" w131 {
      frame False {
        # "潜动、启动"
        n132 = property on="计时状态" class="Bool (严格)"() -> ("Value"=w132:bool)  [unwired: 2 in, 2 out]
        n133 = case shown="真" w132 {
          frame False {
          }
          frame True {
            n134 = while {
              stop <- w144 stop-if-true
              n135 = property on="串口号" class="VISAName"() -> ("Value"=w143:refnum<visa-resource-name>)  [unwired: 2 in, 2 out]
              n136 = property on="试验项目" class="Ring (严格)"() -> ("Value"=w147:u16)  [unwired: 2 in, 2 out]
              n137 = Wait (ms)(milliseconds to wait=u32 500 ("等待时间（毫秒）")) -> ()  [unwired: 1 out]
              n138 = case shown="1" w147 {
                tunnel: [w177 w249] -> w134
                tunnel: w143 -> [w175 w248]
                tunnel: [w172 w244] -> w139
                frame 0, Default {
                  # "潜动测试"
                  n139 = call "读电能信息.vi"("串口号"=w175) -> ("应答"=w176:string)  [unwired: 2 in]
                  n140 = property on="试验结果" class="Arr (严格)"() -> ("Value"=w173:string[])  [unwired: 2 in, 2 out]
                  n141 = Equal?(x=w173, y=string[] ["不合格", "不合格", "不合格"]) -> (x = y?=w172:bool[])
                  n142 = case shown="\"错误\", 默认" w176 {
                    tunnel: [w178 FALSE FALSE] -> w177
                    frame "读电能" {
                      n143 = global read "程序全局.vi" "电能信息"() -> (w219:T16)
                      n144 = Unbundle By Name(w219) -> ("有功功率"=w207:sgl, "有功电能"=w190:sgl, "有功脉冲"=w208:u64, "脉冲输入功率"=w204:sgl[], "脉冲电能累计"=w189:sgl[], "输入脉冲数"=w183:sgl[])
                      n145 = Number To Fractional String(number=w207, precision (6)=i16 3 ("精度(6)")) -> (F-format string=w214:string)  [unwired: 2 in]
                      n146 = Number To Fractional String(number=w190, precision (6)=i16 4 ("精度(6)")) -> (F-format string=w215:string)  [unwired: 2 in]
                      n147 = Number To Fractional String(number=w208, precision (6)=i16 0 ("精度(6)")) -> (F-format string=w205:string)  [unwired: 2 in]
                      n148 = property on="本机表格" class="Tbl (严格)"() -> ("Value"=w217:string[][])  [unwired: 2 in, 2 out]
                      n149 = Number To Fractional String(number=w204, precision (6)=i16 3 ("精度(6)")) -> (F-format string=w197:string[])  [unwired: 2 in]
                      n150 = Number To Fractional String(number=w189, precision (6)=i16 4 ("精度(6)")) -> (F-format string=w196:string[])  [unwired: 2 in]
                      n151 = Number To Fractional String(number=w183, precision (6)=i16 0 ("精度(6)")) -> (F-format string=w195:string[])  [unwired: 2 in]
                      n152 = property on="单点显示表" class="Tbl (严格)"() -> ("Value"=w179:string[][])  [unwired: 2 in, 2 out]
                      n153 = Index Array(array=w217, index (col)=0 ("禁用的索引 (列)")) -> (element=w211:string[])  [unwired: 1 in]
                      n154 = Replace Array Subset(array=w211, new element=w214, index=6 ("索引")) -> (w192:string[])
                      n155 = Replace Array Subset(array=w192, new element=w215, index=7 ("索引")) -> (w193:string[])
                      n156 = Replace Array Subset(array=w193, new element=w205, index=5 ("索引")) -> (w194:string[])
                      n157 = Replace Array Subset(array=w217, new element=w194, index (col)=0 ("禁用的索引 (列)")) -> (w218:string[][])  [unwired: 1 in]
                      n158 = Replace Array Subset(array=w179, new element=w197, index (row)=1 ("索引 (行)")) -> (w200:string[][])  [unwired: 1 in]
                      n159 = Replace Array Subset(array=w200, new element=w196, index (row)=2 ("索引 (行)")) -> (w199:string[][])  [unwired: 1 in]
                      n160 = Replace Array Subset(array=w199, new element=w195, index (row)=0 ("索引 (行)")) -> (w198:string[][])  [unwired: 1 in]
                      n161 = property on="本机表格" class="Tbl (严格)"("Value"=w218) -> ()  [unwired: 2 in, 2 out]
                      n162 = property on="单点显示表" class="Tbl (严格)"("Value"=w198) -> ()  [unwired: 2 in, 2 out]
                      n163 = property on="已用秒数" class="DigNum (严格)"() -> ("Value"=w181:dbl)  [unwired: 2 in, 2 out]
                      n164 = property on="测试时间" class="DigNum (严格)"() -> ("Value"=w184:dbl)  [unwired: 2 in, 2 out]
                      n165 = Divide(x=w181, y=60.0) -> (x/y=w180:dbl)
                      n166 = Greater Or Equal?(x=w180, y=w184) -> (x >= y?=w178:bool)
                      n167 = case shown="假" w178 {
                        tunnel: w183 -> [w220 w229]
                        frame True {
                          n168 = for {
                            N: 3 -> [_]
                            tunnel: w220 -> [w226] mode=indexing
                            tunnel: [w224] -> w221 mode=indexing
                            n169 = property on="脉冲数" class="DigNum (严格)"() -> ("Value"=w223:u32)  [unwired: 2 in, 2 out]
                            n170 = Greater Or Equal?(x=w226, y=w223) -> (x >= y?=w225:bool)
                            n171 = case shown="真" w225 {
                              tunnel: ["合格" "不合格"] -> w224
                              frame False {
                              }
                              frame True {
                              }
                            }
                          }
                          n172 = property on="试验结果" class="Arr (严格)"("Value"=w221) -> ()  [unwired: 2 in, 2 out]
                        }
                        frame False {
                          n173 = for {
                            N: 3 -> [_]
                            tunnel: w229 -> [w235] mode=indexing
                            tunnel: [w233] -> w230 mode=indexing
                            n174 = property on="脉冲数" class="DigNum (严格)"() -> ("Value"=w232:u32)  [unwired: 2 in, 2 out]
                            n175 = Greater Or Equal?(x=w235, y=w232) -> (x >= y?=w234:bool)
                            n176 = case shown="真" w234 {
                              tunnel: ["正在检定" "不合格"] -> w233
                              frame False {
                              }
                              frame True {
                              }
                            }
                          }
                          n177 = property on="试验结果" class="Arr (严格)"("Value"=w230) -> ()  [unwired: 2 in, 2 out]
                        }
                      }
                    }
                    frame "超时" {
                      n178 = property on="提示信息" class="Bool (严格)"("BoolText.Text"="读电能超时！", "Val(Sgnl)"=TRUE ("提示信息")) -> ()  [unwired: 2 in, 2 out]
                    }
                    frame "错误", Default {
                      n179 = property on="提示信息" class="Bool (严格)"("BoolText.Text"="读电能错误！", "Val(Sgnl)"=TRUE ("提示信息")) -> ()  [unwired: 2 in, 2 out]
                    }
                  }
                }
                frame 1 {
                  # "启动测试"
                  n180 = call "读电能信息.vi"("串口号"=w248) -> ("应答"=w247:string)  [unwired: 2 in]
                  n181 = property on="试验结果" class="Arr (严格)"() -> ("Value"=w245:string[])  [unwired: 2 in, 2 out]
                  n182 = Equal?(x=w245, y=string[] ["合格", "合格", "合格"]) -> (x = y?=w244:bool[])
                  n183 = case shown="\"读电能\"" w247 {
                    tunnel: [w250 FALSE FALSE] -> w249
                    frame "读电能" {
                      n184 = global read "程序全局.vi" "电能信息"() -> (w291:T16)
                      n185 = Unbundle By Name(w291) -> ("有功功率"=w279:sgl, "有功电能"=w262:sgl, "有功脉冲"=w280:u64, "脉冲输入功率"=w276:sgl[], "脉冲电能累计"=w261:sgl[], "输入脉冲数"=w255:sgl[])
                      n186 = Number To Fractional String(number=w279, precision (6)=i16 3 ("精度(6)")) -> (F-format string=w286:string)  [unwired: 2 in]
                      n187 = Number To Fractional String(number=w262, precision (6)=i16 4 ("精度(6)")) -> (F-format string=w287:string)  [unwired: 2 in]
                      n188 = Number To Fractional String(number=w280, precision (6)=i16 0 ("精度(6)")) -> (F-format string=w277:string)  [unwired: 2 in]
                      n189 = property on="本机表格" class="Tbl (严格)"() -> ("Value"=w289:string[][])  [unwired: 2 in, 2 out]
                      n190 = Number To Fractional String(number=w276, precision (6)=i16 3 ("精度(6)")) -> (F-format string=w269:string[])  [unwired: 2 in]
                      n191 = Number To Fractional String(number=w261, precision (6)=i16 4 ("精度(6)")) -> (F-format string=w268:string[])  [unwired: 2 in]
                      n192 = Number To Fractional String(number=w255, precision (6)=i16 0 ("精度(6)")) -> (F-format string=w267:string[])  [unwired: 2 in]
                      n193 = Index Array(array=w289, index (col)=0 ("禁用的索引 (列)")) -> (element=w283:string[])  [unwired: 1 in]
                      n194 = Replace Array Subset(array=w283, new element=w286, index=6 ("索引")) -> (w264:string[])
                      n195 = Replace Array Subset(array=w264, new element=w287, index=7 ("索引")) -> (w265:string[])
                      n196 = Replace Array Subset(array=w265, new element=w277, index=5 ("索引")) -> (w266:string[])
                      n197 = property on="单点显示表" class="Tbl (严格)"() -> ("Value"=w251:string[][])  [unwired: 2 in, 2 out]
                      n198 = Replace Array Subset(array=w289, new element=w266, index (col)=0 ("禁用的索引 (列)")) -> (w290:string[][])  [unwired: 1 in]
                      n199 = Replace Array Subset(array=w251, new element=w269, index (row)=1 ("索引 (行)")) -> (w272:string[][])  [unwired: 1 in]
                      n200 = Replace Array Subset(array=w272, new element=w268, index (row)=2 ("索引 (行)")) -> (w271:string[][])  [unwired: 1 in]
                      n201 = Replace Array Subset(array=w271, new element=w267, index (row)=0 ("索引 (行)")) -> (w270:string[][])  [unwired: 1 in]
                      n202 = property on="本机表格" class="Tbl (严格)"("Value"=w290) -> ()  [unwired: 2 in, 2 out]
                      n203 = property on="单点显示表" class="Tbl (严格)"("Value"=w270) -> ()  [unwired: 2 in, 2 out]
                      n204 = property on="已用秒数" class="DigNum (严格)"() -> ("Value"=w253:dbl)  [unwired: 2 in, 2 out]
                      n205 = property on="测试时间" class="DigNum (严格)"() -> ("Value"=w256:dbl)  [unwired: 2 in, 2 out]
                      n206 = Divide(x=w253, y=60.0) -> (x/y=w252:dbl)
                      n207 = Greater Or Equal?(x=w252, y=w256) -> (x >= y?=w250:bool)
                      n208 = case shown="真" w250 {
                        tunnel: w255 -> [w292 w301]
                        frame True {
                          n209 = for {
                            N: 3 -> [_]
                            tunnel: w292 -> [w298] mode=indexing
                            tunnel: [w296] -> w293 mode=indexing
                            n210 = property on="脉冲数" class="DigNum (严格)"() -> ("Value"=w295:u32)  [unwired: 2 in, 2 out]
                            n211 = Less?(x=w298, y=w295) -> (x < y?=w297:bool)
                            n212 = case shown="真" w297 {
                              tunnel: ["合格" "不合格"] -> w296
                              frame False {
                              }
                              frame True {
                              }
                            }
                          }
                          n213 = property on="试验结果" class="Arr (严格)"("Value"=w293) -> ()  [unwired: 2 in, 2 out]
                        }
                        frame False {
                          n214 = for {
                            N: 3 -> [_]
                            tunnel: w301 -> [w307] mode=indexing
                            tunnel: [w305] -> w302 mode=indexing
                            n215 = property on="脉冲数" class="DigNum (严格)"() -> ("Value"=w304:u32)  [unwired: 2 in, 2 out]
                            n216 = Greater Or Equal?(x=w307, y=w304) -> (x >= y?=w306:bool)
                            n217 = case shown="真" w306 {
                              tunnel: ["正在检定" "合格"] -> w305
                              frame False {
                              }
                              frame True {
                              }
                            }
                          }
                          n218 = property on="试验结果" class="Arr (严格)"("Value"=w302) -> ()  [unwired: 2 in, 2 out]
                        }
                      }
                    }
                    frame "超时" {
                      n219 = property on="提示信息" class="Bool (严格)"("BoolText.Text"="读电能超时！", "Val(Sgnl)"=TRUE ("提示信息")) -> ()  [unwired: 2 in, 2 out]
                    }
                    frame "错误", Default {
                      n220 = property on="提示信息" class="Bool (严格)"("BoolText.Text"="读电能错误！", "Val(Sgnl)"=TRUE ("提示信息")) -> ()  [unwired: 2 in, 2 out]
                    }
                  }
                }
              }
              n221 = Index Array(array=w139, index=2 ("索引")) -> (element=w136:bool)
              n222 = Index Array(array=w139, index=1 ("索引")) -> (element=w137:bool)
              n223 = Index Array(array=w139, index=0 ("索引")) -> (element=w138:bool)
              n224 = global read "系统全局.vi" "退出程序"() -> (w149:bool)
              n225 = property on="计时状态" class="Bool (严格)"() -> ("Value"=w146:bool)  [unwired: 2 in, 2 out]
              n226 = Not(x=w146) -> (.not. x?=w148:bool)
              n227 = Compound Arithmetic op=AND(w138, w137, w136) -> (w135:bool)
              n228 = Or(x=w135, y=w134) -> (x .or. y?=w133:bool)
              n229 = Compound Arithmetic op=OR(w133, w148, w149) -> (w144:bool)
              n230 = case shown="真" w133 {
                frame False {
                }
                frame True {
                  n231 = property on="控制选项卡" class="TabCtl (严格)"("PageSelVis"=TRUE ("页选择器可见")) -> ()  [unwired: 2 in, 2 out]
                  n232 = property on="开始试验" class="Bool (严格)"("Val(Sgnl)"=FALSE ("值(信号)")) -> ()  [unwired: 2 in, 2 out]
                }
              }
              n233 = case shown="真" w144 {
                tunnel: w143 -> [_ w153]
                frame False {
                }
                frame True {
                  w154 = u16 2 items=["电压停止", "电流停止", "全部停止"] ("启动项")
                  n234 = call "输出停止.vi"("启动项"=w154, "串口号"=w153) -> ("应答"=w152:string)  [unwired: 3 in]
                  n235 = case shown="\"错误\", 默认" w152 {
                    frame "错误", Default {
                      n236 = property on="提示信息" class="Bool (严格)"("BoolText.Text"="停止失败！", "Val(Sgnl)"=TRUE ("提示信息")) -> ()  [unwired: 2 in, 2 out]
                    }
                    frame "超时" {
                    }
                    frame "正确" {
                      n237 = Number To Fractional String(number=0.0 ("数字"), precision (6)=i16 3 ("精度(6)")) -> (F-format string=w166:string)  [unwired: 2 in]
                      n238 = Number To Fractional String(number=0.0 ("数字"), precision (6)=i16 3 ("精度(6)")) -> (F-format string=w168:string)  [unwired: 2 in]
                      n239 = property on="本机表格" class="Tbl (严格)"() -> ("Value"=w159:string[][])  [unwired: 2 in, 2 out]
                      n240 = Index Array(array=w159, index (col)=0 ("禁用的索引 (列)")) -> (element=w161:string[])  [unwired: 1 in]
                      n241 = Replace Array Subset(array=w161, new element=w166, index=0 ("索引")) -> (w164:string[])
                      n242 = Replace Array Subset(array=w164, new element=w168, index=1 ("索引")) -> (w171:string[])
                      n243 = Replace Array Subset(array=w159, new element=w171, index (col)=0 ("禁用的索引 (列)")) -> (w170:string[][])  [unwired: 1 in]
                      n244 = property on="本机表格" class="Tbl (严格)"("Value"=w170) -> ()  [unwired: 2 in, 2 out]
                    }
                  }
                }
              }
            }
          }
        }
      }
      frame True {
        n245 = Tick Count (ms)() -> (millisecond timer value=w316:u32)
        n246 = property on="表3已等待时间" class="DigNum (严格)"("Value"=w316) -> ()  [unwired: 2 in, 2 out]
        n247 = property on="表2已等待时间" class="DigNum (严格)"("Value"=w316) -> ()  [unwired: 2 in, 2 out]
        n248 = property on="表1已等待时间" class="DigNum (严格)"("Value"=w316) -> ()  [unwired: 2 in, 2 out]
        n249 = property on="单点检定" class="Bool (严格)"() -> ("Value"=w317:bool)  [unwired: 2 in, 2 out]
        n250 = case "电能单点误差检定" shown="假" w317 {
          frame False {
            n251 = while {
              tunnel: [w363] -> w318
              i -> [w358]
              stop <- w363 stop-if-true
              w371 = sgl 0.01
              w378 = sgl 0.0 ("默认(0 DBL)")
              n252 = property on="表1" class="Bool (严格)"() -> ("Value"=w351:bool)  [unwired: 2 in, 2 out]
              n253 = property on="E检定表格" class="Tbl (严格)"() -> ("Value"=w389:string[][])  [unwired: 2 in, 2 out]
              n254 = property on="表2" class="Bool (严格)"() -> ("Value"=w352:bool)  [unwired: 2 in, 2 out]
              n255 = global read "系统全局.vi" "退出程序"() -> (w392:bool)
              n256 = property on="E行数" class="DigNum (严格)"() -> ("Value"=w368:i32)  [unwired: 2 in, 2 out]
              n257 = property on="表3" class="Bool (严格)"() -> ("Value"=w353:bool)  [unwired: 2 in, 2 out]
              n258 = case shown="真" w351 {
                frame False {
                  n259 = property on="表1OK" class="Bool (严格)"("Value"=TRUE ("表2OK")) -> ()  [unwired: 2 in, 2 out]
                }
                frame True {
                  n260 = property on="表1OK" class="Bool (严格)"("Value"=FALSE ("表2OK")) -> ()  [unwired: 2 in, 2 out]
                }
              }
              n261 = property on="检定状态" class="Bool (严格)"() -> ("Value"=w390:bool)  [unwired: 2 in, 2 out]
              n262 = Index Array(array=w389, index (row)=w358) -> (element=w365:string[])  [unwired: 1 in]
              n263 = Decrement(x=w368) -> (x-1=w367:i32)
              n264 = case shown="假" w352 {
                frame False {
                  n265 = property on="表2OK" class="Bool (严格)"("Value"=TRUE ("表2OK")) -> ()  [unwired: 2 in, 2 out]
                }
                frame True {
                  n266 = property on="表2OK" class="Bool (严格)"("Value"=FALSE ("表2OK")) -> ()  [unwired: 2 in, 2 out]
                }
              }
              n267 = property on="电能显示表" class="Tbl (严格)"() -> ("Active Cell"=w355:T17)  [unwired: 2 in, 2 out]
              n268 = Bundle By Name(cluster=w355, "Row"=w358, "Column"=-2) -> (w350:T17)
              n269 = case shown="假" w353 {
                frame False {
                  n270 = property on="表3OK" class="Bool (严格)"("Value"=TRUE ("表3OK")) -> ()  [unwired: 2 in, 2 out]
                }
                frame True {
                  n271 = property on="表3OK" class="Bool (严格)"("Value"=FALSE ("表3OK")) -> ()  [unwired: 2 in, 2 out]
                }
              }
              n272 = property on="E检定行" class="DigNum (严格)"("Value"=w358) -> ()  [unwired: 2 in, 2 out]
              n273 = Not(x=w390) -> (.not. x?=w391:bool)
              n274 = Greater?(x=w358, y=w367) -> (0:w361:bool)
              n275 = Index Array(array=w365, index=0 ("索引")) -> (element=w383:string)
              n276 = Index Array(array=w365, index=1 ("索引")) -> (element=w382:string)
              n277 = Index Array(array=w365, index=2 ("索引")) -> (element=w381:string)
              n278 = Index Array(array=w365, index=3 ("索引")) -> (element=w380:string)
              n279 = Index Array(array=w365, index=4 ("索引")) -> (element=w379:string)
              n280 = Index Array(array=w365, index=5 ("索引")) -> (element=w364:string)
              n281 = Not(x=w361) -> (.not. x?=w359:bool)
              n282 = Compound Arithmetic op=OR(w361, w391, w392) -> (w363:bool)
              n283 = property on="电能检定通道" class="Ring (严格)"() -> ("Value"=w349:u16)  [unwired: 2 in, 2 out]
              n284 = property on="电能显示表" class="Tbl (严格)"("Active Cell"=w350) -> (error out=w357:errorcluster)  [unwired: 2 in, 1 out]
              n285 = Fract/Exp String To Number(string=w383, default (0 dbl)=w378) -> (number=w373:sgl)  [unwired: 2 in, 1 out]
              n286 = Fract/Exp String To Number(string=w382, default (0 dbl)=w378) -> (number=w374:sgl)  [unwired: 2 in, 1 out]
              n287 = Fract/Exp String To Number(string=w381, default (0 dbl)=w378) -> (number=w376:sgl)  [unwired: 2 in, 1 out]
              n288 = Fract/Exp String To Number(string=w380, default (0 dbl)=w378) -> (number=w375:sgl)  [unwired: 2 in, 1 out]
              n289 = Fract/Exp String To Number(string=w379, default (0 dbl)=w378) -> (number=w377:sgl)  [unwired: 2 in, 1 out]
              n290 = case shown="假" w359 {
                selector: w359 -> [w418 _]
                frame False {
                  n291 = property on="开始检定" class="Bool (严格)"("Val(Sgnl)"=w418) -> ()  [unwired: 2 in, 2 out]
                  n292 = property on="检定状态" class="Bool (严格)"("Value"=w418) -> ()  [unwired: 2 in, 2 out]
                }
                frame True {
                }
              }
              n293 = property on="电能显示表" class="Tbl (严格)"(error in=w357, "Cell BG Color"=u32 16056130) -> ()  [unwired: 1 in, 2 out]
              n294 = global write "程序全局.vi" "误差限值"(w377) -> ()
              n295 = Multiply(x=w373, y=w374) -> (x*y=w370:sgl)
              n296 = Multiply(x=w376, y=w375) -> (x*y=w369:sgl)
              n297 = property on="下一点" class="Bool (严格)"("Value"=FALSE ("值(信号)")) -> ()  [unwired: 2 in, 2 out]
              n298 = property on="串口号" class="VISAName"() -> ("Value"=w362:refnum<visa-resource-name>)  [unwired: 2 in, 2 out]
              n299 = Multiply(x=w371, y=w369) -> (x*y=w348:sgl)
              n300 = case shown="3" w349 {
                tunnel: w348 -> [w393 w395 w401 w407]
                tunnel: [w393 w394 w400 w406] -> w347
                frame 0, Default {
                }
                frame 1 {
                  n301 = property on="小信号变比(A/1mv)" class="Clust (严格)"() -> ("Value"=w399:cluster{"电流2":sgl, "电流3":sgl, "电流4":sgl})  [unwired: 2 in, 2 out]
                  n302 = Unbundle(w399) -> ("电流2"=w397:sgl)  [unwired: 2 out]
                  n303 = Multiply(x=w397, y=1000.0) -> (x*y=w396:dbl)
                  n304 = Divide(x=w395, y=w396) -> (x/y=w394:dbl)
                }
                frame 2 {
                  n305 = property on="小信号变比(A/1mv)" class="Clust (严格)"() -> ("Value"=w405:cluster{"电流2":sgl, "电流3":sgl, "电流4":sgl})  [unwired: 2 in, 2 out]
                  n306 = Unbundle(w405) -> ("电流3"=w403:sgl)  [unwired: 2 out]
                  n307 = Multiply(x=w403, y=1000.0) -> (x*y=w402:dbl)
                  n308 = Divide(x=w401, y=w402) -> (x/y=w400:dbl)
                }
                frame 3 {
                  n309 = property on="小信号变比(A/1mv)" class="Clust (严格)"() -> ("Value"=w411:cluster{"电流2":sgl, "电流3":sgl, "电流4":sgl})  [unwired: 2 in, 2 out]
                  n310 = Unbundle(w411) -> ("电流4"=w409:sgl)  [unwired: 2 out]
                  n311 = Multiply(x=w409, y=1000.0) -> (x*y=w408:dbl)
                  n312 = Divide(x=w407, y=w408) -> (x/y=w406:dbl)
                }
              }
              n313 = Multiply(x=w371, y=w370) -> (x*y=w372:sgl)
              n314 = case shown="假" w363 {
                tunnel: w372 -> [w423 _]
                tunnel: w348 -> [w422 _]
                tunnel: w364 -> [w421 _]
                tunnel: w362 -> [w420 _]
                tunnel: w347 -> [w419 _]
                frame False {
                  n315 = case shown="\"是\"" w421 {
                    tunnel: w423 -> [_ w438]
                    tunnel: w422 -> [_ w433]
                    tunnel: w420 -> [_ w435]
                    tunnel: w419 -> [_ w432]
                    frame "否", Default {
                      n316 = property on="E行数" class="DigNum (严格)"() -> ("Value"=w426:i32)  [unwired: 2 in, 2 out]
                      n317 = property on="E检定行" class="DigNum (严格)"() -> ("Value"=w428:i32)  [unwired: 2 in, 2 out]
                      n318 = Decrement(x=w426) -> (x-1=w425:i32)
                      n319 = property on="下一点" class="Bool (严格)"("Value"=FALSE ("下一点")) -> ()  [unwired: 2 in, 2 out]
                      n320 = Greater Or Equal?(x=w428, y=w425) -> (x >= y?=w427:bool)
                      n321 = case shown="真" w427 {
                        frame False {
                        }
                        frame True {
                          n322 = property on="开始检定" class="Bool (严格)"("Val(Sgnl)"=FALSE ("值")) -> ()  [unwired: 2 in, 2 out]
                          n323 = property on="检定状态" class="Bool (严格)"("Value"=FALSE ("检定状态")) -> ()  [unwired: 2 in, 2 out]
                        }
                      }
                    }
                    frame "是" {
                      w431 = u32 85 ("电流档位")
                      w437 = sgl 0.0 ("电压纹波")
                      # "0x55自动档位"
                      n324 = property on="电能检定通道" class="Ring (严格)"() -> ("Value"=w434:u16)  [unwired: 2 in, 2 out]
                      n325 = call "高精度写.vi"("电压幅值"=w438, "电压纹波"=w437, "串口号"=w435, "电压档位"=w431, "电流幅值"=w432, "电流档位值"=w431, "纹波频率"=w437, "电流纹波"=w437, "电流通道"=w434) -> ("应答"=w436:string)  [unwired: 6 in]
                      n326 = case shown="\"正确\"" w436 {
                        tunnel: w435 -> [_ _ w444]
                        tunnel: w438 -> [_ _ w448]
                        tunnel: w433 -> [_ _ w447]
                        frame "错误", Default {
                          n327 = property on="提示信息" class="Bool (严格)"("BoolText.Text"="高精度写错误！", "Val(Sgnl)"=TRUE ("提示信息")) -> ()  [unwired: 2 in, 2 out]
                        }
                        frame "超时" {
                          n328 = property on="提示信息" class="Bool (严格)"("BoolText.Text"="高精度写超时！", "Val(Sgnl)"=TRUE ("提示信息")) -> ()  [unwired: 2 in, 2 out]
                        }
                        frame "正确" {
                          w446 = u16 2 items=["电压启动", "电流启动", "全部启动"] ("启动项")
                          n329 = property on="电能检定通道" class="Ring (严格)"() -> ("Value"=w443:u16)  [unwired: 2 in, 2 out]
                          n330 = call "输出启动.vi"("电流通道"=w443, "启动项"=w446, "串口号"=w444) -> ("应答"=w445:string)  [unwired: 2 in]
                          n331 = case shown="\"正确\"" w445 {
                            tunnel: w448 -> [_ _ w455]
                            tunnel: w447 -> [_ _ w454]
                            tunnel: w444 -> [_ _ w457]
                            frame "错误", Default {
                              n332 = property on="提示信息" class="Bool (严格)"("BoolText.Text"="输出失败！", "Val(Sgnl)"=TRUE ("提示信息")) -> ()  [unwired: 2 in, 2 out]
                            }
                            frame "超时" {
                              n333 = property on="提示信息" class="Bool (严格)"("BoolText.Text"="输出超时！", "Val(Sgnl)"=TRUE ("提示信息")) -> ()  [unwired: 2 in, 2 out]
                            }
                            frame "正确" {
                              n334 = stacked-sequence {
                                tunnel: w457 -> [_ _ w472]
                                frame #0 {
                                n335 = Wait (ms)(milliseconds to wait=u32 3000 ("等待时间（毫秒）")) -> ()  [unwired: 1 out]
                                }
                                frame #1 {
                                n336 = Tick Count (ms)() -> (millisecond timer value=w471:u32)
                                n337 = property on="表3已等待时间" class="DigNum (严格)"("Value"=w471) -> ()  [unwired: 2 in, 2 out]
                                n338 = property on="表2已等待时间" class="DigNum (严格)"("Value"=w471) -> ()  [unwired: 2 in, 2 out]
                                n339 = property on="表1已等待时间" class="DigNum (严格)"("Value"=w471) -> ()  [unwired: 2 in, 2 out]
                                }
                                frame #2 {
                                n340 = while {
                                tunnel: w472 -> [w473]
                                stop <- w475 stop-if-true
                                n341 = stacked-sequence {
                                tunnel: w473 -> [w481 w524 w567 w610 w634]
                                frame #0 {
                                n342 = property on="表1" class="Bool (严格)"() -> ("Value"=w482:bool)  [unwired: 2 in, 2 out]
                                n343 = property on="表1OK" class="Bool (严格)"() -> ("Value"=w480:bool)  [unwired: 2 in, 2 out]
                                n344 = case shown="真" w482 {
                                tunnel: w481 -> [_ w484]
                                tunnel: w480 -> [_ w483]
                                frame False {
                                }
                                frame True {
                                n345 = case shown="假" w483 {
                                tunnel: w484 -> [w512 _]
                                frame False {
                                w492 = 0 ("索引")
                                # "等待时间超出了超时设定"
                                # "1圈的时间"
                                # "脉冲频率"
                                n346 = call "有效状态.vi"("脉冲选择"=u8 0, "串口号"=w512) -> ("应答"=w511:string)  [unwired: 3 in]
                                n347 = Wait (ms)(milliseconds to wait=u32 100 ("等待时间（毫秒）")) -> ()  [unwired: 1 out]
                                n348 = Tick Count (ms)() -> (millisecond timer value=w509:u32)
                                n349 = global read "程序全局.vi" "电能表参数数组"() -> (w505:T18)
                                n350 = property on="表1已等待时间" class="DigNum (严格)"() -> ("Value"=w508:dbl)  [unwired: 2 in, 2 out]
                                n351 = case shown="\"读有效\"" w511 {
                                frame "假", Default {
                                }
                                frame "读有效" {
                                n352 = global read "程序全局.vi" "有效状态"() -> (w520:u8)
                                n353 = Greater?(x=w520, y=u8 0) -> (0:w518:bool)
                                n354 = case shown="真" w518 {
                                frame False {
                                }
                                frame True {
                                n355 = global write "程序全局.vi" "有效状态"(u8 0 ("有效状态")) -> ()
                                n356 = property on="表1OK" class="Bool (严格)"("Value"=TRUE ("表1OK")) -> ()  [unwired: 2 in, 2 out]
                                }
                                }
                                }
                                }
                                n357 = Subtract(x=w509, y=w508) -> (x-y=w507:dbl)
                                n358 = Index Array(array=w505, index=w492) -> (element=w504:T13)
                                n359 = Divide(x=w507, y=1000.0) -> (x/y=w494:dbl)
                                n360 = Unbundle By Name(w504) -> ("有功常数"=w503:i32)  [unwired: 1 out]
                                n361 = property on="增加等待时间(s)" class="DigNum (严格)"() -> ("Value"=w486:dbl)  [unwired: 2 in, 2 out]
                                n362 = Divide(x=w503, y=3600.0) -> (x/y=w501:dbl)
                                n363 = Divide(x=w501, y=1000.0) -> (x/y=w499:dbl)
                                n364 = property on="当前功率" class="DigNum (严格)"() -> ("Value"=w498:dbl)  [unwired: 2 in, 2 out]
                                n365 = property on="超时圈数" class="DigNum (严格)"() -> ("Value"=w495:sgl)  [unwired: 2 in, 2 out]
                                n366 = Multiply(x=w498, y=w499) -> (x*y=w497:dbl)
                                n367 = Reciprocal(x=w497) -> (1/x=w496:dbl)
                                n368 = Multiply(x=w496, y=w495) -> (x*y=w487:dbl)
                                n369 = Add(x=w487, y=w486) -> (x+y=w485:dbl)
                                n370 = Greater?(x=w494, y=w485) -> (0:w493:bool)
                                n371 = case shown="真" w493 {
                                tunnel: w492 -> [_ w516]
                                frame False {
                                }
                                frame True {
                                w515 = TRUE ("表1OK")
                                n372 = property on="超时记录" class="Arr (严格)"() -> ("Value"=w517:bool[])  [unwired: 2 in, 2 out]
                                n373 = property on="表1OK" class="Bool (严格)"("Value"=w515) -> ()  [unwired: 2 in, 2 out]
                                n374 = Replace Array Subset(array=w517, new element=w515, index=w516) -> (w514:bool[])
                                n375 = property on="超时记录" class="Arr (严格)"("Value"=w514) -> ()  [unwired: 2 in, 2 out]
                                }
                                }
                                n376 = Number To Fractional String(number=w485, precision (6)=i16 3 ("精度(6)")) -> (F-format string=w490:string)  [unwired: 2 in]
                                n377 = Concatenate Strings(w490, "秒" ("字符串")) -> (w489:string)
                                n378 = property on="表1超时时间" class="Str"("Value"=w489) -> ()  [unwired: 2 in, 2 out]
                                }
                                frame True {
                                }
                                }
                                }
                                }
                                }
                                frame #1 {
                                n379 = property on="表2OK" class="Bool (严格)"() -> ("Value"=w523:bool)  [unwired: 2 in, 2 out]
                                n380 = property on="表2" class="Bool (严格)"() -> ("Value"=w525:bool)  [unwired: 2 in, 2 out]
                                n381 = case shown="真" w525 {
                                tunnel: w524 -> [_ w527]
                                tunnel: w523 -> [_ w526]
                                frame False {
                                }
                                frame True {
                                n382 = case shown="假" w526 {
                                tunnel: w527 -> [w555 _]
                                frame False {
                                w535 = 1 ("索引")
                                # "等待时间超出了超时设定"
                                # "1圈的时间"
                                # "脉冲频率"
                                n383 = property on="表2已等待时间" class="DigNum (严格)"() -> ("Value"=w536:dbl)  [unwired: 2 in, 2 out]
                                n384 = call "有效状态.vi"("脉冲选择"=u8 1, "串口号"=w555) -> ("应答"=w554:string)  [unwired: 3 in]
                                n385 = Tick Count (ms)() -> (millisecond timer value=w552:u32)
                                n386 = global read "程序全局.vi" "电能表参数数组"() -> (w549:T18)
                                n387 = Wait (ms)(milliseconds to wait=u32 100 ("等待时间（毫秒）")) -> ()  [unwired: 1 out]
                                n388 = case shown="\"读有效\"" w554 {
                                frame "假", Default {
                                }
                                frame "读有效" {
                                n389 = global read "程序全局.vi" "有效状态"() -> (w563:u8)
                                n390 = Greater?(x=w563, y=u8 0) -> (0:w561:bool)
                                n391 = case shown="真" w561 {
                                frame False {
                                }
                                frame True {
                                n392 = global write "程序全局.vi" "有效状态"(u8 0 ("有效状态")) -> ()
                                n393 = property on="表2OK" class="Bool (严格)"("Value"=TRUE ("表1OK")) -> ()  [unwired: 2 in, 2 out]
                                }
                                }
                                }
                                }
                                n394 = Subtract(x=w552, y=w536) -> (x-y=w551:dbl)
                                n395 = Index Array(array=w549, index=w535) -> (element=w548:T13)
                                n396 = Divide(x=w551, y=1000.0) -> (x/y=w538:dbl)
                                n397 = Unbundle By Name(w548) -> ("有功常数"=w547:i32)
                                n398 = Divide(x=w547, y=3600.0) -> (x/y=w545:dbl)
                                n399 = Divide(x=w545, y=1000.0) -> (x/y=w543:dbl)
                                n400 = property on="当前功率" class="DigNum (严格)"() -> ("Value"=w542:dbl)  [unwired: 2 in, 2 out]
                                n401 = property on="增加等待时间(s)" class="DigNum (严格)"() -> ("Value"=w529:dbl)  [unwired: 2 in, 2 out]
                                n402 = property on="超时圈数" class="DigNum (严格)"() -> ("Value"=w539:sgl)  [unwired: 2 in, 2 out]
                                n403 = Multiply(x=w542, y=w543) -> (x*y=w541:dbl)
                                n404 = Reciprocal(x=w541) -> (1/x=w540:dbl)
                                n405 = Multiply(x=w540, y=w539) -> (x*y=w530:dbl)
                                n406 = Add(x=w530, y=w529) -> (x+y=w528:dbl)
                                n407 = Greater?(x=w538, y=w528) -> (0:w537:bool)
                                n408 = case shown="真" w537 {
                                tunnel: w535 -> [_ w558]
                                frame False {
                                }
                                frame True {
                                w557 = TRUE ("表1OK")
                                n409 = property on="超时记录" class="Arr (严格)"() -> ("Value"=w560:bool[])  [unwired: 2 in, 2 out]
                                n410 = property on="表2OK" class="Bool (严格)"("Value"=w557) -> ()  [unwired: 2 in, 2 out]
                                n411 = Replace Array Subset(array=w560, new element=w557, index=w558) -> (w559:bool[])
                                n412 = property on="超时记录" class="Arr (严格)"("Value"=w559) -> ()  [unwired: 2 in, 2 out]
                                }
                                }
                                n413 = Number To Fractional String(number=w528, precision (6)=i16 3 ("精度(6)")) -> (F-format string=w533:string)  [unwired: 2 in]
                                n414 = Concatenate Strings(w533, "秒" ("字符串")) -> (w531:string)
                                n415 = property on="表2超时时间" class="Str"("Value"=w531) -> ()  [unwired: 2 in, 2 out]
                                }
                                frame True {
                                }
                                }
                                }
                                }
                                }
                                frame #2 {
                                n416 = property on="表3OK" class="Bool (严格)"() -> ("Value"=w566:bool)  [unwired: 2 in, 2 out]
                                n417 = property on="表3" class="Bool (严格)"() -> ("Value"=w568:bool)  [unwired: 2 in, 2 out]
                                n418 = case shown="真" w568 {
                                tunnel: w567 -> [_ w570]
                                tunnel: w566 -> [_ w569]
                                frame False {
                                }
                                frame True {
                                n419 = case shown="假" w569 {
                                tunnel: w570 -> [w598 _]
                                frame False {
                                w578 = 2 ("索引")
                                # "等待时间超出了超时设定"
                                # "1圈的时间"
                                # "脉冲频率"
                                n420 = property on="表3已等待时间" class="DigNum (严格)"() -> ("Value"=w579:dbl)  [unwired: 2 in, 2 out]
                                n421 = Tick Count (ms)() -> (millisecond timer value=w595:u32)
                                n422 = global read "程序全局.vi" "电能表参数数组"() -> (w592:T18)
                                n423 = call "有效状态.vi"("脉冲选择"=u8 2, "串口号"=w598) -> ("应答"=w597:string)  [unwired: 3 in]
                                n424 = Wait (ms)(milliseconds to wait=u32 100 ("等待时间（毫秒）")) -> ()  [unwired: 1 out]
                                n425 = case shown="\"读有效\"" w597 {
                                frame "假", Default {
                                }
                                frame "读有效" {
                                n426 = global read "程序全局.vi" "有效状态"() -> (w606:u8)
                                n427 = Greater?(x=w606, y=u8 0) -> (0:w604:bool)
                                n428 = case shown="真" w604 {
                                frame False {
                                }
                                frame True {
                                n429 = global write "程序全局.vi" "有效状态"(u8 0 ("有效状态")) -> ()
                                n430 = property on="表3OK" class="Bool (严格)"("Value"=TRUE ("表1OK")) -> ()  [unwired: 2 in, 2 out]
                                }
                                }
                                }
                                }
                                n431 = Subtract(x=w595, y=w579) -> (x-y=w594:dbl)
                                n432 = Index Array(array=w592, index=w578) -> (element=w591:T13)
                                n433 = Divide(x=w594, y=1000.0) -> (x/y=w581:dbl)
                                n434 = Unbundle By Name(w591) -> ("有功常数"=w590:i32)  [unwired: 1 out]
                                n435 = Divide(x=w590, y=3600.0) -> (x/y=w588:dbl)
                                n436 = Divide(x=w588, y=1000.0) -> (x/y=w586:dbl)
                                n437 = property on="当前功率" class="DigNum (严格)"() -> ("Value"=w585:dbl)  [unwired: 2 in, 2 out]
                                n438 = property on="增加等待时间(s)" class="DigNum (严格)"() -> ("Value"=w571:dbl)  [unwired: 2 in, 2 out]
                                n439 = property on="超时圈数" class="DigNum (严格)"() -> ("Value"=w582:sgl)  [unwired: 2 in, 2 out]
                                n440 = Multiply(x=w585, y=w586) -> (x*y=w584:dbl)
                                n441 = Reciprocal(x=w584) -> (1/x=w583:dbl)
                                n442 = Multiply(x=w583, y=w582) -> (x*y=w573:dbl)
                                n443 = Add(x=w573, y=w571) -> (x+y=w572:dbl)
                                n444 = Greater?(x=w581, y=w572) -> (0:w580:bool)
                                n445 = case shown="真" w580 {
                                tunnel: w578 -> [_ w601]
                                frame False {
                                }
                                frame True {
                                w600 = TRUE ("表1OK")
                                n446 = property on="超时记录" class="Arr (严格)"() -> ("Value"=w603:bool[])  [unwired: 2 in, 2 out]
                                n447 = Replace Array Subset(array=w603, new element=w600, index=w601) -> (w602:bool[])
                                n448 = property on="表3OK" class="Bool (严格)"("Value"=w600) -> ()  [unwired: 2 in, 2 out]
                                n449 = property on="超时记录" class="Arr (严格)"("Value"=w602) -> ()  [unwired: 2 in, 2 out]
                                }
                                }
                                n450 = Number To Fractional String(number=w572, precision (6)=i16 3 ("精度(6)")) -> (F-format string=w576:string)  [unwired: 2 in]
                                n451 = Concatenate Strings(w576, "秒" ("字符串")) -> (w574:string)
                                n452 = property on="表3超时时间" class="Str"("Value"=w574) -> ()  [unwired: 2 in, 2 out]
                                }
                                frame True {
                                }
                                }
                                }
                                }
                                }
                                frame #3 {
                                n453 = call "读电能信息.vi"("串口号"=w610) -> ("应答"=w609:string)  [unwired: 2 in]
                                n454 = case shown="\"错误\"" w609 {
                                frame "读电能" {
                                n455 = global read "程序全局.vi" "电能信息"() -> (w631:T16)
                                n456 = Unbundle By Name(w631) -> ("有功功率"=w619:sgl, "有功电能"=w613:sgl, "有功脉冲"=w620:u64)  [unwired: 2 out]
                                n457 = property on="本机表格" class="Tbl (严格)"() -> ("Value"=w629:string[][])  [unwired: 2 in, 2 out]
                                n458 = Index Array(array=w629, index (col)=0 ("禁用的索引 (列)")) -> (element=w623:string[])  [unwired: 1 in]
                                n459 = Number To Fractional String(number=w619, precision (6)=i16 3 ("精度(6)")) -> (F-format string=w626:string)  [unwired: 2 in]
                                n460 = Number To Fractional String(number=w613, precision (6)=i16 4 ("精度(6)")) -> (F-format string=w627:string)  [unwired: 2 in]
                                n461 = Number To Fractional String(number=w620, precision (6)=i16 0 ("精度(6)")) -> (F-format string=w617:string)  [unwired: 2 in]
                                n462 = Replace Array Subset(array=w623, new element=w626, index=6 ("索引")) -> (w614:string[])
                                n463 = Replace Array Subset(array=w614, new element=w627, index=7 ("索引")) -> (w615:string[])
                                n464 = Replace Array Subset(array=w615, new element=w617, index=5 ("索引")) -> (w616:string[])
                                n465 = Replace Array Subset(array=w629, new element=w616, index (col)=0 ("禁用的索引 (列)")) -> (w630:string[][])  [unwired: 1 in]
                                n466 = property on="本机表格" class="Tbl (严格)"("Value"=w630) -> ()  [unwired: 2 in, 2 out]
                                }
                                frame "超时" {
                                }
                                frame Default {
                                }
                                frame "错误" {
                                n467 = property on="提示信息" class="Bool (严格)"("BoolText.Text"="读电能错误！", "Val(Sgnl)"=TRUE ("提示信息")) -> ()  [unwired: 2 in, 2 out]
                                }
                                }
                                }
                                frame #4 {
                                n468 = property on="表1OK" class="Bool (严格)"() -> ("Value"=w638:bool)  [unwired: 2 in, 2 out]
                                n469 = property on="表2OK" class="Bool (严格)"() -> ("Value"=w637:bool)  [unwired: 2 in, 2 out]
                                n470 = property on="表3OK" class="Bool (严格)"() -> ("Value"=w636:bool)  [unwired: 2 in, 2 out]
                                n471 = Compound Arithmetic op=AND(w638, w637, w636) -> (w635:bool)
                                n472 = case shown="真" w635 {
                                tunnel: w634 -> [_ w645]
                                frame False {
                                }
                                frame True {
                                n473 = property on="E检定行" class="DigNum (严格)"() -> ("Value"=w639:i32)  [unwired: 2 in, 2 out]
                                n474 = flat-sequence {
                                tunnel: [w649] -> w646
                                tunnel: w645 -> [w648]
                                frame #0 {
                                n475 = Wait (ms)(milliseconds to wait=u32 500 ("等待时间（毫秒）")) -> ()  [unwired: 1 out]
                                }
                                frame #1 {
                                n476 = call "读电能信息.vi"("串口号"=w648) -> ("应答"=w649:string)  [unwired: 2 in]
                                }
                                }
                                n477 = property on="电能显示表" class="Tbl (严格)"() -> ("Active Cell"=w643:T17)  [unwired: 2 in, 2 out]
                                n478 = Bundle By Name(cluster=w643, "Row"=w639, "Column"=-2) -> (w640:T17)
                                n479 = property on="电能显示表" class="Tbl (严格)"("Active Cell"=w640) -> (error out=w644:errorcluster)  [unwired: 2 in, 1 out]
                                n480 = property on="电能显示表" class="Tbl (严格)"(error in=w644, "Cell BG Color"=u32 16448250) -> ()  [unwired: 1 in, 2 out]
                                n481 = case shown="\"错误\"" w646 {
                                frame "读电能" {
                                n482 = global read "程序全局.vi" "电能信息"() -> (w702:T16)
                                n483 = Unbundle By Name(w702) -> ("有功功率"=w690:sgl, "有功电能"=w683:sgl, "有功脉冲"=w691:u64, "电能误差"=w651:sgl[], "脉冲电能累计"=w682:sgl[])
                                n484 = property on="E检定表格" class="Tbl (严格)"() -> ("Value"=w660:string[][])  [unwired: 2 in, 2 out]
                                n485 = property on="E检定行" class="DigNum (严格)"() -> ("Value"=w652:i32)  [unwired: 2 in, 2 out]
                                n486 = property on="本机表格" class="Tbl (严格)"() -> ("Value"=w700:string[][])  [unwired: 2 in, 2 out]
                                n487 = Index Array(array=w660, index (col)=4 ("禁用的索引 (列)")) -> (element=w658:string[])  [unwired: 1 in]
                                n488 = Index Array(array=w658, index=w652) -> (element=w657:string)
                                n489 = Absolute Value(x=w651) -> (abs(x)=w655:sgl[])
                                n490 = Number To Fractional String(number=w651, precision (6)=i16 3 ("精度(6)")) -> (F-format string=w681:string[])  [unwired: 2 in]
                                n491 = Number To Fractional String(number=w682, precision (6)=i16 4 ("精度(6)")) -> (F-format string=w680:string[])  [unwired: 2 in]
                                n492 = Index Array(array=w700, index (col)=0 ("禁用的索引 (列)")) -> (element=w694:string[])  [unwired: 1 in]
                                n493 = Number To Fractional String(number=w690, precision (6)=i16 3 ("精度(6)")) -> (F-format string=w697:string)  [unwired: 2 in]
                                n494 = Number To Fractional String(number=w683, precision (6)=i16 4 ("精度(6)")) -> (F-format string=w698:string)  [unwired: 2 in]
                                n495 = Number To Fractional String(number=w691, precision (6)=i16 0 ("精度(6)")) -> (F-format string=w688:string)  [unwired: 2 in]
                                n496 = Fract/Exp String To Number(string=w657, default (0 dbl)=sgl 0.0 ("默认(0 DBL)")) -> (number=w654:sgl)  [unwired: 2 in, 1 out]
                                n497 = property on="电能显示表" class="Tbl (严格)"() -> ("Value"=w668:string[][])  [unwired: 2 in, 2 out]
                                n498 = Index Array(array=w680, index=0 ("索引")) -> (element=w674:string)
                                n499 = Index Array(array=w680, index=1 ("索引")) -> (element=w673:string)
                                n500 = Index Array(array=w680, index=2 ("索引")) -> (element=w672:string)
                                n501 = Replace Array Subset(array=w694, new element=w697, index=6 ("索引")) -> (w685:string[])
                                n502 = Replace Array Subset(array=w685, new element=w698, index=7 ("索引")) -> (w686:string[])
                                n503 = Replace Array Subset(array=w686, new element=w688, index=5 ("索引")) -> (w687:string[])
                                n504 = Greater?(x=w655, y=w654) -> (0:w653:bool[])
                                n505 = for {
                                N: 3 -> [_]
                                tunnel: w653 -> [w707] mode=indexing
                                tunnel: w652 -> [w712]
                                i -> [w704]
                                n506 = property on="超时记录" class="Arr (严格)"() -> ("Value"=w705:bool[])  [unwired: 2 in, 2 out]
                                n507 = property on="电能显示表" class="Tbl (严格)"() -> ("Active Cell"=w711:T17)  [unwired: 2 in, 2 out]
                                n508 = Multiply(x=2, y=w704) -> (x*y=w709:i32)
                                n509 = Increment(x=w709) -> (x+1=w708:i32)
                                n510 = Index Array(array=w705, index=w704) -> (element=w703:bool)
                                n511 = Or(x=w707, y=w703) -> (x .or. y?=w706:bool)
                                n512 = case shown="假" w706 {
                                tunnel: w708 -> [w717 w723]
                                tunnel: w712 -> [w718 w724]
                                tunnel: w711 -> [w716 w722]
                                frame True {
                                n513 = Bundle By Name(cluster=w716, "Row"=w718, "Column"=w717) -> (w715:T17)
                                n514 = property on="电能显示表" class="Tbl (严格)"("Active Cell"=w715) -> (error out=w714:errorcluster)  [unwired: 2 in, 1 out]
                                n515 = property on="电能显示表" class="Tbl (严格)"(error in=w714, "Cell BG Color"=u32 16056130) -> ()  [unwired: 1 in, 2 out]
                                }
                                frame False {
                                n516 = Bundle By Name(cluster=w722, "Row"=w724, "Column"=w723) -> (w721:T17)
                                n517 = property on="电能显示表" class="Tbl (严格)"("Active Cell"=w721) -> (error out=w720:errorcluster)  [unwired: 2 in, 1 out]
                                n518 = property on="电能显示表" class="Tbl (严格)"(error in=w720, "Cell BG Color"=u32 16448250) -> ()  [unwired: 1 in, 2 out]
                                }
                                }
                                }
                                n519 = property on="E检定行" class="DigNum (严格)"() -> ("Value"=w665:i32)  [unwired: 2 in, 2 out]
                                n520 = Insert Into Array(array=w681, index=0 ("索引"), new element=w674) -> (w676:string[])
                                n521 = Insert Into Array(array=w676, index=2 ("索引"), new element=w673) -> (w675:string[])
                                n522 = Insert Into Array(array=w675, index=4 ("索引"), new element=w672) -> (w667:string[])
                                n523 = Replace Array Subset(array=w700, new element=w687, index (col)=0 ("禁用的索引 (列)")) -> (w701:string[][])  [unwired: 1 in]
                                n524 = Replace Array Subset(array=w668, new element=w667, index (row)=w665) -> (w666:string[][])  [unwired: 1 in]
                                n525 = property on="本机表格" class="Tbl (严格)"("Value"=w701) -> ()  [unwired: 2 in, 2 out]
                                n526 = property on="电能显示表" class="Tbl (严格)"("Value"=w666) -> ()  [unwired: 2 in, 2 out]
                                n527 = property on="下一点" class="Bool (严格)"("Value"=TRUE ("值(信号)")) -> ()  [unwired: 2 in, 2 out]
                                }
                                frame "超时" {
                                }
                                frame Default {
                                }
                                frame "错误" {
                                n528 = property on="提示信息" class="Bool (严格)"("BoolText.Text"="读电能错误！", "Val(Sgnl)"=TRUE ("提示信息")) -> ()  [unwired: 2 in, 2 out]
                                }
                                }
                                }
                                }
                                }
                                }
                                n529 = property on="下一点" class="Bool (严格)"() -> ("Value"=w474:bool)  [unwired: 2 in, 2 out]
                                n530 = Wait (ms)(milliseconds to wait=u32 10 ("等待时间（毫秒）")) -> ()  [unwired: 1 out]
                                n531 = property on="检定状态" class="Bool (严格)"() -> ("Value"=w476:bool)  [unwired: 2 in, 2 out]
                                n532 = global read "系统全局.vi" "退出程序"() -> (w477:bool)
                                n533 = Not(x=w476) -> (.not. x?=w478:bool)
                                n534 = Compound Arithmetic op=OR(w474, w478, w477) -> (w475:bool)
                                n535 = case shown="真" w474 {
                                frame False {
                                }
                                frame True {
                                w728 = FALSE ("表1OK")
                                n536 = property on="下一点" class="Bool (严格)"("Value"=FALSE ("值(信号)")) -> ()  [unwired: 2 in, 2 out]
                                n537 = property on="表1" class="Bool (严格)"() -> ("Value"=w736:bool)  [unwired: 2 in, 2 out]
                                n538 = Tick Count (ms)() -> (millisecond timer value=w735:u32)
                                n539 = case shown="真" w736 {
                                frame False {
                                n540 = property on="表1OK" class="Bool (严格)"("Value"=TRUE ("表2OK")) -> ()  [unwired: 2 in, 2 out]
                                }
                                frame True {
                                n541 = property on="表1OK" class="Bool (严格)"("Value"=FALSE ("表2OK")) -> ()  [unwired: 2 in, 2 out]
                                }
                                }
                                n542 = property on="表1已等待时间" class="DigNum (严格)"("Value"=w735) -> ()  [unwired: 2 in, 2 out]
                                n543 = property on="表2" class="Bool (严格)"() -> ("Value"=w737:bool)  [unwired: 2 in, 2 out]
                                n544 = property on="表2已等待时间" class="DigNum (严格)"("Value"=w735) -> ()  [unwired: 2 in, 2 out]
                                n545 = case shown="真" w737 {
                                frame False {
                                n546 = property on="表2OK" class="Bool (严格)"("Value"=TRUE ("表2OK")) -> ()  [unwired: 2 in, 2 out]
                                }
                                frame True {
                                n547 = property on="表2OK" class="Bool (严格)"("Value"=FALSE ("表2OK")) -> ()  [unwired: 2 in, 2 out]
                                }
                                }
                                n548 = property on="表3已等待时间" class="DigNum (严格)"("Value"=w735) -> ()  [unwired: 2 in, 2 out]
                                n549 = property on="表3" class="Bool (严格)"() -> ("Value"=w738:bool)  [unwired: 2 in, 2 out]
                                n550 = case shown="真" w738 {
                                frame False {
                                n551 = property on="表3OK" class="Bool (严格)"("Value"=TRUE ("表3OK")) -> ()  [unwired: 2 in, 2 out]
                                }
                                frame True {
                                n552 = property on="表3OK" class="Bool (严格)"("Value"=FALSE ("表3OK")) -> ()  [unwired: 2 in, 2 out]
                                }
                                }
                                n553 = property on="超时记录" class="Arr (严格)"() -> ("Value"=w734:bool[])  [unwired: 2 in, 2 out]
                                n554 = Replace Array Subset(array=w734, new element=w728, index=0 ("索引")) -> (w731:bool[])
                                n555 = Replace Array Subset(array=w731, new element=w728, index=1 ("索引")) -> (w730:bool[])
                                n556 = Replace Array Subset(array=w730, new element=w728, index=2 ("索引")) -> (w727:bool[])
                                n557 = property on="超时记录" class="Arr (严格)"("Value"=w727) -> ()  [unwired: 2 in, 2 out]
                                }
                                }
                                }
                                }
                              }
                              n558 = property on="本机表格" class="Tbl (严格)"() -> ("Value"=w469:string[][])  [unwired: 2 in, 2 out]
                              n559 = Index Array(array=w469, index (col)=0 ("禁用的索引 (列)")) -> (element=w467:string[])  [unwired: 1 in]
                              n560 = Number To Fractional String(number=w455, precision (6)=i16 3 ("精度(6)")) -> (F-format string=w462:string)  [unwired: 2 in]
                              n561 = Number To Fractional String(number=w454, precision (6)=i16 3 ("精度(6)")) -> (F-format string=w461:string)  [unwired: 2 in]
                              n562 = Replace Array Subset(array=w467, new element=w462, index=0 ("索引")) -> (w464:string[])
                              n563 = Replace Array Subset(array=w464, new element=w461, index=1 ("索引")) -> (w458:string[])
                              n564 = Replace Array Subset(array=w469, new element=w458, index (col)=0 ("禁用的索引 (列)")) -> (w459:string[][])  [unwired: 1 in]
                              n565 = property on="本机表格" class="Tbl (严格)"("Value"=w459) -> ()  [unwired: 2 in, 2 out]
                              n566 = Multiply(x=w455, y=w454) -> (x*y=w453:sgl)
                              n567 = property on="当前功率" class="DigNum (严格)"("Value"=w453) -> ()  [unwired: 2 in, 2 out]
                            }
                          }
                        }
                      }
                    }
                  }
                }
                frame True {
                }
              }
            }
            n568 = case shown="真" w318 {
              frame False {
              }
              frame True {
                w328 = u16 2 items=["电压停止", "电流停止", "全部停止"] ("启动项")
                n569 = property on="E检定行" class="DigNum (严格)"() -> ("Value"=w325:i32)  [unwired: 2 in, 2 out]
                n570 = property on="电能显示表" class="Tbl (严格)"() -> ("Active Cell"=w324:T17)  [unwired: 2 in, 2 out]
                n571 = Bundle By Name(cluster=w324, "Row"=w325, "Column"=-2) -> (w321:T17)
                n572 = property on="电能显示表" class="Tbl (严格)"("Active Cell"=w321) -> (error out=w320:errorcluster)  [unwired: 2 in, 1 out]
                n573 = property on="电能显示表" class="Tbl (严格)"(error in=w320, "Cell BG Color"=u32 16448250) -> ()  [unwired: 1 in, 2 out]
                n574 = Wait (ms)(milliseconds to wait=u32 20 ("等待时间（毫秒）")) -> ()  [unwired: 1 out]
                n575 = property on="串口号" class="VISAName"() -> ("Value"=w327:refnum<visa-resource-name>)  [unwired: 2 in, 2 out]
                n576 = call "输出停止.vi"("启动项"=w328, "串口号"=w327) -> ("应答"=w326:string)  [unwired: 3 in]
                n577 = case shown="\"正确\"" w326 {
                  frame Default {
                  }
                  frame "错误" {
                    n578 = One Button Dialog(message="停止失败") -> ()  [unwired: 1 in, 1 out]
                  }
                  frame "超时" {
                    n579 = One Button Dialog(message="停止超时") -> ()  [unwired: 1 in, 1 out]
                  }
                  frame "正确" {
                    n580 = Number To Fractional String(number=0.0 ("数字"), precision (6)=i16 3 ("精度(6)")) -> (F-format string=w341:string)  [unwired: 2 in]
                    n581 = Number To Fractional String(number=0.0 ("数字"), precision (6)=i16 3 ("精度(6)")) -> (F-format string=w343:string)  [unwired: 2 in]
                    n582 = property on="本机表格" class="Tbl (严格)"() -> ("Value"=w334:string[][])  [unwired: 2 in, 2 out]
                    n583 = Index Array(array=w334, index (col)=0 ("禁用的索引 (列)")) -> (element=w336:string[])  [unwired: 1 in]
                    n584 = Replace Array Subset(array=w336, new element=w341, index=0 ("索引")) -> (w339:string[])
                    n585 = Replace Array Subset(array=w339, new element=w343, index=1 ("索引")) -> (w346:string[])
                    n586 = Replace Array Subset(array=w334, new element=w346, index (col)=0 ("禁用的索引 (列)")) -> (w345:string[][])  [unwired: 1 in]
                    n587 = property on="本机表格" class="Tbl (严格)"("Value"=w345) -> ()  [unwired: 2 in, 2 out]
                    n588 = One Button Dialog(message="停止输出") -> ()  [unwired: 1 in, 1 out]
                  }
                }
              }
            }
          }
          frame True {
            w779 = sgl 0.01 ("y")
            w746 = u32 85 ("电流档位")
            w754 = sgl 0.0 ("电压纹波")
            n589 = property on="电能检定通道" class="Ring (严格)"() -> ("Value"=w749:u16)  [unwired: 2 in, 2 out]
            n590 = property on="E检定表格" class="Tbl (严格)"() -> ("Value"=w755:string[][])  [unwired: 2 in, 2 out]
            n591 = property on="E当前行" class="DigNum (严格)"() -> ("Value"=w756:i32)  [unwired: 2 in, 2 out]
            n592 = Index Array(array=w755, index (row)=w756) -> (element=w772:string[])  [unwired: 1 in]
            n593 = property on="串口号" class="VISAName"() -> ("Value"=w753:refnum<visa-resource-name>)  [unwired: 2 in, 2 out]
            n594 = property on="电能检定通道" class="Ring (严格)"() -> ("Value"=w751:u16)  [unwired: 2 in, 2 out]
            n595 = Index Array(array=w772, index=0 ("索引")) -> (element=w757:string)
            n596 = Index Array(array=w772, index=1 ("索引")) -> (element=w762:string)
            n597 = Index Array(array=w772, index=2 ("索引")) -> (element=w763:string)
            n598 = Index Array(array=w772, index=3 ("索引")) -> (element=w768:string)
            n599 = Index Array(array=w772, index=4 ("索引")) -> (element=w769:string)
            n600 = Fract/Exp String To Number(string=w769, default (0 dbl)=sgl 0.0) -> (number=w780:sgl)  [unwired: 2 in, 1 out]
            n601 = global write "程序全局.vi" "误差限值"(w780) -> ()
            n602 = Fract/Exp String To Number(string=w757, default (0 dbl)=sgl 0.0) -> (number=w773:sgl)  [unwired: 2 in, 1 out]
            n603 = Fract/Exp String To Number(string=w762, default (0 dbl)=sgl 0.0) -> (number=w778:sgl)  [unwired: 2 in, 1 out]
            n604 = Fract/Exp String To Number(string=w763, default (0 dbl)=sgl 0.0) -> (number=w774:sgl)  [unwired: 2 in, 1 out]
            n605 = Fract/Exp String To Number(string=w768, default (0 dbl)=sgl 0.0) -> (number=w776:sgl)  [unwired: 2 in, 1 out]
            n606 = Multiply(x=w779, y=w773) -> (x*y=w777:sgl)
            n607 = Multiply(x=w779, y=w774) -> (x*y=w775:sgl)
            n608 = Multiply(x=w775, y=w776) -> (x*y=w747:sgl)
            n609 = case shown="3" w749 {
              tunnel: w747 -> [w781 w782 w789 w796]
              tunnel: [w781 w783 w790 w795] -> w748
              frame 0, Default {
              }
              frame 1 {
                n610 = property on="小信号变比(A/1mv)" class="Clust (严格)"() -> ("Value"=w787:cluster{"电流2":sgl, "电流3":sgl, "电流4":sgl})  [unwired: 2 in, 2 out]
                n611 = Unbundle(w787) -> ("电流2"=w785:sgl)  [unwired: 2 out]
                n612 = Multiply(x=w785, y=1000.0) -> (x*y=w784:dbl)
                n613 = Divide(x=w782, y=w784) -> (x/y=w783:dbl)
              }
              frame 2 {
                n614 = property on="小信号变比(A/1mv)" class="Clust (严格)"() -> ("Value"=w793:cluster{"电流2":sgl, "电流3":sgl, "电流4":sgl})  [unwired: 2 in, 2 out]
                n615 = Unbundle(w793) -> ("电流3"=w791:sgl)  [unwired: 2 out]
                n616 = Multiply(x=w791, y=1000.0) -> (x*y=w788:dbl)
                n617 = Divide(x=w789, y=w788) -> (x/y=w790:dbl)
              }
              frame 3 {
                n618 = property on="小信号变比(A/1mv)" class="Clust (严格)"() -> ("Value"=w799:cluster{"电流2":sgl, "电流3":sgl, "电流4":sgl})  [unwired: 2 in, 2 out]
                n619 = Unbundle(w799) -> ("电流4"=w794:sgl)  [unwired: 2 out]
                n620 = Multiply(x=w794, y=1000.0) -> (x*y=w797:dbl)
                n621 = Divide(x=w796, y=w797) -> (x/y=w795:dbl)
              }
            }
            n622 = Multiply(x=w777, y=w778) -> (x*y=w750:sgl)
            n623 = call "高精度写.vi"("电压幅值"=w750, "电压纹波"=w754, "串口号"=w753, "电压档位"=w746, "电流幅值"=w748, "电流档位值"=w746, "纹波频率"=w754, "电流纹波"=w754, "电流通道"=w751) -> ("应答"=w752:string)  [unwired: 6 in]
            n624 = case shown="\"正确\"" w752 {
              tunnel: w753 -> [_ _ w805]
              tunnel: w750 -> [_ _ w809]
              tunnel: w747 -> [_ _ w808]
              frame "错误", Default {
                n625 = property on="提示信息" class="Bool (严格)"("BoolText.Text"="高精度写错误！", "Val(Sgnl)"=TRUE ("提示信息")) -> ()  [unwired: 2 in, 2 out]
              }
              frame "超时" {
                n626 = property on="提示信息" class="Bool (严格)"("BoolText.Text"="高精度写超时！", "Val(Sgnl)"=TRUE ("提示信息")) -> ()  [unwired: 2 in, 2 out]
              }
              frame "正确" {
                w807 = u16 2 items=["电压启动", "电流启动", "全部启动"] ("启动项")
                n627 = property on="电能检定通道" class="Ring (严格)"() -> ("Value"=w804:u16)  [unwired: 2 in, 2 out]
                n628 = call "输出启动.vi"("电流通道"=w804, "启动项"=w807, "串口号"=w805) -> ("应答"=w806:string)  [unwired: 2 in]
                n629 = case "电能单点检定" shown="\"正确\"" w806 {
                  tunnel: w809 -> [_ _ w818]
                  tunnel: w808 -> [_ _ w816]
                  tunnel: w805 -> [_ _ w814]
                  frame "错误", Default {
                    n630 = property on="提示信息" class="Bool (严格)"("BoolText.Text"="输出失败！", "Val(Sgnl)"=TRUE ("提示信息")) -> ()  [unwired: 2 in, 2 out]
                  }
                  frame "超时" {
                    n631 = property on="提示信息" class="Bool (严格)"("BoolText.Text"="输出超时！", "Val(Sgnl)"=TRUE ("提示信息")) -> ()  [unwired: 2 in, 2 out]
                  }
                  frame "正确" {
                    n632 = while {
                      tunnel: w814 -> [w855]
                      tunnel: [w856] -> w815
                      stop <- w856 stop-if-true
                      n633 = call "读电能信息.vi"("串口号"=w855) -> ("应答"=w854:string)  [unwired: 2 in]
                      n634 = Wait (ms)(milliseconds to wait=u32 500 ("等待时间（毫秒）")) -> ()  [unwired: 1 out]
                      n635 = case shown="\"读电能\"" w854 {
                        frame "读电能" {
                          w868 = i16 3 ("精度(6)")
                          n636 = global read "程序全局.vi" "电能信息"() -> (w905:T16)
                          n637 = Unbundle By Name(w905) -> ("有功功率"=w893:sgl, "有功电能"=w867:sgl, "有功脉冲"=w894:u64, "标准偏差值"=w869:sgl[], "电能误差"=w890:sgl[], "脉冲输入功率"=w889:sgl[], "脉冲电能累计"=w866:sgl[], "输入脉冲数"=w888:sgl[])
                          n638 = property on="单点显示表" class="Tbl (严格)"() -> ("Value"=w865:string[][])  [unwired: 2 in, 2 out]
                          n639 = Number To Fractional String(number=w869, precision (6)=w868) -> (F-format string=w882:string[])  [unwired: 2 in]
                          n640 = Number To Fractional String(number=w890, precision (6)=w868) -> (F-format string=w881:string[])  [unwired: 2 in]
                          n641 = Number To Fractional String(number=w889, precision (6)=w868) -> (F-format string=w875:string[])  [unwired: 2 in]
                          n642 = Number To Fractional String(number=w866, precision (6)=i16 4 ("精度(6)")) -> (F-format string=w874:string[])  [unwired: 2 in]
                          n643 = Number To Fractional String(number=w888, precision (6)=i16 0 ("精度(6)")) -> (F-format string=w873:string[])  [unwired: 2 in]
                          n644 = Number To Fractional String(number=w893, precision (6)=i16 3 ("精度(6)")) -> (F-format string=w900:string)  [unwired: 2 in]
                          n645 = Number To Fractional String(number=w867, precision (6)=i16 4 ("精度(6)")) -> (F-format string=w901:string)  [unwired: 2 in]
                          n646 = Number To Fractional String(number=w894, precision (6)=i16 0 ("精度(6)")) -> (F-format string=w891:string)  [unwired: 2 in]
                          n647 = property on="本机表格" class="Tbl (严格)"() -> ("Value"=w903:string[][])  [unwired: 2 in, 2 out]
                          n648 = Replace Array Subset(array=w865, new element=w882, index (row)=3 ("索引 (行)")) -> (w880:string[][])  [unwired: 1 in]
                          n649 = Replace Array Subset(array=w880, new element=w881, index (row)=4 ("索引 (行)")) -> (w879:string[][])  [unwired: 1 in]
                          n650 = Replace Array Subset(array=w879, new element=w875, index (row)=1 ("索引 (行)")) -> (w878:string[][])  [unwired: 1 in]
                          n651 = Replace Array Subset(array=w878, new element=w874, index (row)=2 ("索引 (行)")) -> (w877:string[][])  [unwired: 1 in]
                          n652 = Replace Array Subset(array=w877, new element=w873, index (row)=0 ("索引 (行)")) -> (w876:string[][])  [unwired: 1 in]
                          n653 = Index Array(array=w903, index (col)=0 ("禁用的索引 (列)")) -> (element=w897:string[])  [unwired: 1 in]
                          n654 = Replace Array Subset(array=w897, new element=w900, index=6 ("索引")) -> (w870:string[])
                          n655 = Replace Array Subset(array=w870, new element=w901, index=7 ("索引")) -> (w871:string[])
                          n656 = Replace Array Subset(array=w871, new element=w891, index=5 ("索引")) -> (w872:string[])
                          n657 = property on="单点显示表" class="Tbl (严格)"("Value"=w876) -> ()  [unwired: 2 in, 2 out]
                          n658 = Replace Array Subset(array=w903, new element=w872, index (col)=0 ("禁用的索引 (列)")) -> (w904:string[][])  [unwired: 1 in]
                          n659 = property on="本机表格" class="Tbl (严格)"("Value"=w904) -> ()  [unwired: 2 in, 2 out]
                        }
                        frame "超时" {
                        }
                        frame "错误", Default {
                        }
                      }
                      n660 = global read "系统全局.vi" "退出程序"() -> (w858:bool)
                      n661 = property on="检定状态" class="Bool (严格)"() -> ("Value"=w857:bool)  [unwired: 2 in, 2 out]
                      n662 = Not(x=w857) -> (.not. x?=w859:bool)
                      n663 = Compound Arithmetic op=OR(w859, w858) -> (w856:bool)
                    }
                    n664 = case shown="真" w815 {
                      tunnel: w814 -> [_ w831]
                      frame False {
                      }
                      frame True {
                        w832 = u16 2 items=["电压停止", "电流停止", "全部停止"] ("启动项")
                        n665 = call "输出停止.vi"("启动项"=w832, "串口号"=w831) -> ("应答"=w833:string)  [unwired: 3 in]
                        n666 = case shown="\"正确\"" w833 {
                          tunnel: w831 -> [_ _ _ w838]
                          frame Default {
                          }
                          frame "错误" {
                            n667 = property on="提示信息" class="Bool (严格)"("BoolText.Text"="停止失败！", "Val(Sgnl)"=TRUE ("提示信息")) -> ()  [unwired: 2 in, 2 out]
                          }
                          frame "超时" {
                            n668 = property on="提示信息" class="Bool (严格)"("BoolText.Text"="停止超时！", "Val(Sgnl)"=TRUE ("提示信息")) -> ()  [unwired: 2 in, 2 out]
                          }
                          frame "正确" {
                            n669 = call "电能清零.vi"("串口号"=w838) -> ()  [unwired: 2 in, 1 out]
                            n670 = Number To Fractional String(number=0.0 ("数字"), precision (6)=i16 3 ("精度(6)")) -> (F-format string=w848:string)  [unwired: 2 in]
                            n671 = Number To Fractional String(number=0.0 ("数字"), precision (6)=i16 3 ("精度(6)")) -> (F-format string=w850:string)  [unwired: 2 in]
                            n672 = property on="本机表格" class="Tbl (严格)"() -> ("Value"=w841:string[][])  [unwired: 2 in, 2 out]
                            n673 = Index Array(array=w841, index (col)=0 ("禁用的索引 (列)")) -> (element=w843:string[])  [unwired: 1 in]
                            n674 = Replace Array Subset(array=w843, new element=w848, index=0 ("索引")) -> (w846:string[])
                            n675 = Replace Array Subset(array=w846, new element=w850, index=1 ("索引")) -> (w853:string[])
                            n676 = Replace Array Subset(array=w841, new element=w853, index (col)=0 ("禁用的索引 (列)")) -> (w852:string[][])  [unwired: 1 in]
                            n677 = property on="本机表格" class="Tbl (严格)"("Value"=w852) -> ()  [unwired: 2 in, 2 out]
                          }
                        }
                      }
                    }
                    n678 = Number To Fractional String(number=w818, precision (6)=i16 3 ("精度(6)")) -> (F-format string=w823:string)  [unwired: 2 in]
                    n679 = Number To Fractional String(number=w816, precision (6)=i16 3 ("精度(6)")) -> (F-format string=w821:string)  [unwired: 2 in]
                    n680 = property on="本机表格" class="Tbl (严格)"() -> ("Value"=w830:string[][])  [unwired: 2 in, 2 out]
                    n681 = Index Array(array=w830, index (col)=0 ("禁用的索引 (列)")) -> (element=w828:string[])  [unwired: 1 in]
                    n682 = Replace Array Subset(array=w828, new element=w823, index=0 ("索引")) -> (w825:string[])
                    n683 = Replace Array Subset(array=w825, new element=w821, index=1 ("索引")) -> (w817:string[])
                    n684 = Replace Array Subset(array=w830, new element=w817, index (col)=0 ("禁用的索引 (列)")) -> (w819:string[][])  [unwired: 1 in]
                    n685 = property on="本机表格" class="Tbl (严格)"("Value"=w819) -> ()  [unwired: 2 in, 2 out]
                  }
                }
              }
            }
          }
        }
      }
    }
    n686 = global read "系统全局.vi" "退出程序"() -> (w129:bool)
  }
  n687 = disable-structure "电能检定" shown="启用" {
    frame Disabled {
    }
    frame Enabled {
    }
  }
  n688 = while {
    stop <- w907 stop-if-true
    n689 = event shown="[21] \"UI检定操作.输出开关\": 值改变" {
      selector: _ -> [_ _ _ _ _ _ _ _ _ _ _ _ _ _ _ _ _ _ _ _ _ _ _ _ _ _ _ _ _ _ _ _ _ _ _ _ _]
      dyn-events: _ -> [_ _ _ _ _ _ _ _ _ _ _ _ _ _ _ _ _ _ _ _ _ _ _ _ _ _ _ _ _ _ _ _ _ _ _ _ _]
      timeout: 80 -> [_ _ _ _ _ _ _ _ _ _ _ _ _ _ _ _ _ _ _ _ _ _ _ _ _ _ _ _ _ _ _ _ _ _ _ _ _]
      event Timeout {
        n690 = event-data() -> ()  [unwired: 1 in, 2 out]
        n691 = property on="串口灯" class="Bool (严格)"() -> ("Value"=w909:bool)  [unwired: 2 in, 2 out]
        n692 = global read "程序全局.vi" "额定电压"() -> (w910:sgl)
        n693 = case shown="真" w909 {
          frame False {
          }
          frame True {
            n694 = property on="计时状态" class="Bool (严格)"() -> ("Value"=w914:bool)  [unwired: 2 in, 2 out]
            n695 = property on="检定状态" class="Bool (严格)"() -> ("Value"=w913:bool)  [unwired: 2 in, 2 out]
            n696 = Compound Arithmetic op=OR(w914, w913) -> (w912:bool)
            n697 = case shown="假" w912 {
              frame False {
                n698 = property on="串口号" class="VISAName"() -> ("Value"=w915:refnum<visa-resource-name>)  [unwired: 2 in, 2 out]
                n699 = property class="Instr"(reference=w915) -> (reference out=w916:refnum<visa-resource-name>, "Serial Settings:Number of Bytes at Serial Port"=w917:u32)  [unwired: 1 in, 1 out]
                n700 = case shown="1, 默认" w917 {
                  tunnel: w916 -> [_ w918]
                  frame 0 {
                  }
                  frame 1, Default {
                    n701 = flat-sequence {
                      tunnel: w918 -> [w920]
                      frame #0 {
                        n702 = call "unpack.vi"("超时时间"=u32 1000, "串口号输入"=w920) -> ()  [unwired: 4 in, 2 out]
                      }
                      frame #1 {
                        n703 = global read "系统全局.vi" "告警状态"() -> (w923:bool)
                        n704 = property on="开始试验" class="Bool (严格)"("Val(Sgnl)"=FALSE ("值(信号)")) -> ()  [unwired: 2 in, 2 out]
                        n705 = case shown="真" w923 {
                          frame False {
                          }
                          frame True {
                            n706 = global read "系统全局.vi" "告警信息"() -> (w924:string)
                            n707 = One Button Dialog(message=w924) -> ()  [unwired: 1 in, 1 out]
                          }
                        }
                        n708 = property on="A停止" class="Bool (严格)"("Val(Sgnl)"=w923) -> ()  [unwired: 2 in, 2 out]
                        n709 = property on="开始检定" class="Bool (严格)"("Val(Sgnl)"=FALSE ("值(信号)")) -> ()  [unwired: 2 in, 2 out]
                      }
                      frame #2 {
                        n710 = global write "系统全局.vi" "告警状态"(FALSE ("告警状态")) -> ()
                      }
                    }
                  }
                }
              }
              frame True {
                n711 = flat-sequence {
                  frame #0 {
                    n712 = global read "系统全局.vi" "告警状态"() -> (w926:bool)
                    n713 = case shown="真" w926 {
                      frame False {
                      }
                      frame True {
                        n714 = global read "系统全局.vi" "告警信息"() -> (w927:string)
                        n715 = One Button Dialog(message=w927) -> ()  [unwired: 1 in, 1 out]
                      }
                    }
                  }
                  frame #1 {
                    n716 = global write "系统全局.vi" "告警状态"(FALSE ("告警状态")) -> ()
                  }
                }
              }
            }
          }
        }
        n717 = property on="额定电压" class="DigNum (严格)"("Value"=w910) -> ()  [unwired: 2 in, 2 out]
        n718 = property on="额定电压" class="DigNum (严格)"("Value"=w910) -> ()  [unwired: 2 in, 2 out]
        n719 = property on="额定电压" class="DigNum (严格)"("Value"=w910) -> ()  [unwired: 2 in, 2 out]
        n720 = global read "程序全局.vi" "标定电流"() -> (w911:sgl)
        n721 = property on="标定电流" class="DigNum (严格)"("Value"=w911) -> ()  [unwired: 2 in, 2 out]
        n722 = property on="标定电流" class="DigNum (严格)"("Value"=w911) -> ()  [unwired: 2 in, 2 out]
        n723 = property on="标定电流" class="DigNum (严格)"("Value"=w911) -> ()  [unwired: 2 in, 2 out]
      }
      event "提示信息": Value Change {
        n724 = event-data() -> ()  [unwired: 1 in, 5 out]
        n725 = flat-sequence {
          frame #0 {
            n726 = property on="提示信息" class="Bool (严格)"("Value"=FALSE ("提示信息"), "Visible"=TRUE ("可见")) -> ()  [unwired: 2 in, 2 out]
          }
          frame #1 {
            n727 = Wait (ms)(milliseconds to wait=u32 500 ("等待时间（毫秒）")) -> ()  [unwired: 1 out]
          }
          frame #2 {
            n728 = property on="提示信息" class="Bool (严格)"("BoolText.Text"="", "Visible"=FALSE ("可见")) -> ()  [unwired: 2 in, 2 out]
          }
        }
      }
      event "软键盘": Value Change {
        n729 = event-data() -> ("NewVal"=w934:bool)  [unwired: 1 in, 4 out]
        n730 = case shown="真" w934 {
          frame False {
          }
          frame True {
            n731 = call <vilib>:"System Exec.vi"("wait until completion? (T)"=FALSE, "command line"="cmd /c start .\\data\\key.exe") -> ()  [unwired: 6 in, 4 out]
          }
        }
      }
      event "串口连接": Value Change {
        w937 = FALSE ("表2OK")
        n732 = event-data() -> ("NewVal"=w943:bool)  [unwired: 1 in]
        n733 = local read "串口信息"() -> (w942:T14)
        n734 = property on="表1OK" class="Bool (严格)"("Value"=w937) -> ()  [unwired: 2 in, 2 out]
        n735 = property on="表2OK" class="Bool (严格)"("Value"=w937) -> ()  [unwired: 2 in, 2 out]
        n736 = property on="表3OK" class="Bool (严格)"("Value"=w937) -> ()  [unwired: 2 in, 2 out]
        n737 = Unbundle By Name(w942) -> ("串口号"=w941:refnum<visa-resource-name>, "波特率"=w940:u32, "校验位"=w939:u8, "停止位"=w938:u16)
        n738 = case shown="真" w943 {
          tunnel: w941 -> [w944 w959]
          tunnel: w940 -> [_ w966]
          tunnel: w939 -> [_ w965]
          tunnel: w938 -> [_ w964]
          frame False {
            n739 = VISA Close(VISA resource name=w944) -> (error out=w945:errorcluster)  [unwired: 1 in]
            n740 = case shown="错误" w945 {
              frame No Error {
                w946 = FALSE ("发送状态")
                n741 = property on="串口号" class="VISAName"() -> ("Text.Text"=w949:string)  [unwired: 2 in, 2 out]
                n742 = property on="串口信息" class="Clust (严格)"("DisabledEnum"=0) -> ()  [unwired: 2 in, 2 out]
                n743 = Concatenate Strings(w949, "断开连接成功！") -> (w951:string)
                n744 = property on="提示信息" class="Bool (严格)"("BoolText.Text"=w951, "Val(Sgnl)"=TRUE ("提示信息")) -> ()  [unwired: 2 in, 2 out]
                n745 = global write "系统全局.vi" "串口状态"(w946) -> ()
                n746 = local write "串口灯"(w946) -> ()
              }
              frame Error {
                n747 = property on="串口号" class="VISAName"() -> ("Text.Text"=w953:string)  [unwired: 2 in, 2 out]
                n748 = Concatenate Strings(w953, "断开连接失败！") -> (w955:string)
                n749 = property on="提示信息" class="Bool (严格)"("BoolText.Text"=w955, "Val(Sgnl)"=TRUE ("提示信息")) -> ()  [unwired: 2 in, 2 out]
              }
            }
          }
          frame True {
            w958 = T20 48 items=["I/O接收缓冲区"=16, "I/O传输缓冲区"=32, "I/O接收和传输缓冲区"=48] ("Mask")
            n750 = call-poly "VISA Configure Serial Port"("VISA resource name"=w959, "Enable Termination\nChar (T)"=FALSE ("Enable Termination\nChar (T)"), "baud rate (9600)"=w966, "parity (0:none)"=w965, "stop bits (10: 1 bit)"=w964) -> ("VISA resource name out"=w957:refnum<visa-resource-name>, "error out"=w956:errorcluster)  [unwired: 9 in]
            n751 = VISA Set I/O Buffer Size(VISA resource name=w957, mask (16)=w958, size (4096)=u32 4096 ("大小(4096)"), error in (no error)=w956) -> (VISA resource name out=w960:refnum<visa-resource-name>, error out=w961:errorcluster)
            n752 = case shown="错误" w961 {
              selector: w961 -> [_ w998]
              tunnel: w960 -> [w967 w997]
              frame No Error {
                n753 = call "测试连接.vi"("串口号"=w967) -> ("应答"=w968:string)  [unwired: 2 in]
                n754 = case shown="\"正确\"" w968 {
                  tunnel: w967 -> [w969 w975 w981 _]
                  frame "假", Default {
                    n755 = VISA Close(VISA resource name=w969) -> ()  [unwired: 1 in, 1 out]
                    n756 = property on="串口号" class="VISAName"() -> ("Text.Text"=w972:string)  [unwired: 2 in, 2 out]
                    n757 = Concatenate Strings(w972, "ERROR1") -> (w974:string)
                    n758 = property on="提示信息" class="Bool (严格)"("BoolText.Text"=w974, "Val(Sgnl)"=TRUE ("提示信息")) -> ()  [unwired: 2 in, 2 out]
                    n759 = property on="串口连接" class="Bool (严格)"("Value"=FALSE ("串口连接")) -> ()  [unwired: 2 in, 2 out]
                  }
                  frame "错误" {
                    n760 = VISA Close(VISA resource name=w975) -> ()  [unwired: 1 in, 1 out]
                    n761 = property on="串口连接" class="Bool (严格)"("Value"=FALSE ("串口连接")) -> ()  [unwired: 2 in, 2 out]
                    n762 = property on="串口号" class="VISAName"() -> ("Text.Text"=w978:string)  [unwired: 2 in, 2 out]
                    n763 = Concatenate Strings(w978, "连接错误！") -> (w980:string)
                    n764 = property on="提示信息" class="Bool (严格)"("BoolText.Text"=w980, "Val(Sgnl)"=TRUE ("提示信息")) -> ()  [unwired: 2 in, 2 out]
                  }
                  frame "超时" {
                    n765 = VISA Close(VISA resource name=w981) -> ()  [unwired: 1 in, 1 out]
                    n766 = property on="串口连接" class="Bool (严格)"("Value"=FALSE ("串口连接")) -> ()  [unwired: 2 in, 2 out]
                    n767 = property on="串口号" class="VISAName"() -> ("Text.Text"=w984:string)  [unwired: 2 in, 2 out]
                    n768 = Concatenate Strings(w984, "连接超时！") -> (w986:string)
                    n769 = property on="提示信息" class="Bool (严格)"("BoolText.Text"=w986, "Val(Sgnl)"=TRUE ("提示信息")) -> ()  [unwired: 2 in, 2 out]
                  }
                  frame "正确" {
                    w992 = TRUE ("发送状态")
                    n770 = property on="串口号" class="VISAName"() -> ("Text.Text"=w989:string)  [unwired: 2 in, 2 out]
                    n771 = local write "串口灯"(w992) -> ()
                    n772 = global write "系统全局.vi" "串口状态"(w992) -> ()
                    n773 = Concatenate Strings(w989, "连接正确！") -> (w991:string)
                    n774 = property on="串口信息" class="Clust (严格)"("DisabledEnum"=3) -> ()  [unwired: 2 in, 2 out]
                    n775 = property on="提示信息" class="Bool (严格)"("BoolText.Text"=w991, "Val(Sgnl)"=TRUE ("提示信息")) -> ()  [unwired: 2 in, 2 out]
                  }
                }
              }
              frame Error {
                n776 = VISA Close(VISA resource name=w997, error in (no error)=w998) -> (error out=w999:errorcluster)
                n777 = call <vilib>:"Clear Errors.vi"("error in (no error)"=w999) -> ()  [unwired: 5 in, 2 out]
                n778 = property on="串口号" class="VISAName"() -> ("Text.Text"=w994:string)  [unwired: 2 in, 2 out]
                n779 = Concatenate Strings(w994, "无效或被占用！") -> (w996:string)
                n780 = property on="提示信息" class="Bool (严格)"("BoolText.Text"=w996, "Val(Sgnl)"=TRUE ("提示信息")) -> ()  [unwired: 2 in, 2 out]
              }
            }
          }
        }
      }
      event "U操作.UAdd1", "U操作.UAdd10", "U操作.UAdd100", "I操作.IAdd1", "I操作.IAdd10", "I操作.IAdd100": Value Change {
        n781 = event-data() -> ("CtlRef"=w1001:refnum<vi>, "NewVal"=w1000:bool)  [unwired: 1 in, 3 out]
        n782 = case shown="真" w1000 {
          tunnel: w1001 -> [_ w1013]
          frame False {
          }
          frame True {
            n783 = property class="Bool (严格)"(reference=w1013) -> ("Label.Text"=w1011:string, "BoolText.Text"=w1009:string)  [unwired: 1 in, 2 out]
            n784 = Search and Replace String(input string=w1009, search string="V↑ ", replace string=" ") -> (result string=w1003:string)  [unwired: 5 in, 3 out]
            n785 = Search and Replace String(input string=w1003, search string="A↑", replace string=" ") -> (result string=w1002:string)  [unwired: 5 in, 3 out]
            n786 = Fract/Exp String To Number(string=w1002) -> (number=w1006:dbl)  [unwired: 3 in, 1 out]
            n787 = String Subset(string=w1011, length (rest)=3 ("长度（剩余）")) -> (substring=w1010:string)  [unwired: 1 in]
            n788 = case shown="\"UA1\"" w1010 {
              tunnel: w1006 -> [_ w1018 w1019 w1027]
              frame "假", Default {
              }
              frame "UAd" {
                n789 = property on="U幅值" class="DigNum (严格)"() -> ("Maximum"=w1015:dbl)  [unwired: 2 in, 2 out]
                n790 = property on="U幅值" class="DigNum (严格)"() -> ("Value"=w1017:sgl)  [unwired: 2 in, 2 out]
                n791 = Add(x=w1017, y=w1018) -> (x+y=w1016:dbl)
                n792 = Max & Min(x=w1016, y=w1015) -> (min(x,y)=w1014:dbl)  [unwired: 1 out]
                n793 = property on="U幅值" class="DigNum (严格)"("Value"=w1014) -> ()  [unwired: 2 in, 2 out]
              }
              frame "IAd" {
                n794 = property on="I幅值" class="DigNum (严格)"() -> ("Maximum"=w1021:dbl)  [unwired: 2 in, 2 out]
                n795 = property on="I幅值" class="DigNum (严格)"() -> ("Value"=w1023:sgl)  [unwired: 2 in, 2 out]
                n796 = Add(x=w1023, y=w1019) -> (x+y=w1022:dbl)
                n797 = Max & Min(x=w1022, y=w1021) -> (min(x,y)=w1020:dbl)  [unwired: 1 out]
                n798 = property on="I幅值" class="DigNum (严格)"("Value"=w1020) -> ()  [unwired: 2 in, 2 out]
              }
              frame "UA1" {
                n799 = property on="UB_amplitude" class="DigNum (严格)"() -> ("Maximum"=w1024:dbl)  [unwired: 2 in, 2 out]
                n800 = property on="UB_amplitude" class="DigNum (严格)"() -> ("Value"=w1026:sgl)  [unwired: 2 in, 2 out]
                n801 = Add(x=w1026, y=w1027) -> (x+y=w1028:dbl)
                n802 = Max & Min(x=w1028, y=w1024) -> (min(x,y)=w1025:dbl)  [unwired: 1 out]
                n803 = property on="UB_amplitude" class="DigNum (严格)"("Value"=w1025) -> ()  [unwired: 2 in, 2 out]
              }
            }
          }
        }
      }
      event "U操作.USub1", "U操作.USub10", "U操作.USub100", "I操作.ISub1", "I操作.ISub10", "I操作.ISub100": Value Change {
        n804 = event-data() -> ("CtlRef"=w1030:refnum<vi>, "NewVal"=w1029:bool)  [unwired: 1 in, 3 out]
        n805 = case shown="真" w1029 {
          tunnel: w1030 -> [_ w1037]
          frame False {
          }
          frame True {
            n806 = property class="Bool (严格)"(reference=w1037) -> ("Label.Text"=w1036:string, "BoolText.Text"=w1034:string)  [unwired: 1 in, 2 out]
            n807 = Search and Replace String(input string=w1034, search string="A↓", replace string=" ") -> (result string=w1033:string)  [unwired: 5 in, 3 out]
            n808 = Search and Replace String(input string=w1033, search string="V↓", replace string=" ") -> (result string=w1039:string)  [unwired: 5 in, 3 out]
            n809 = Fract/Exp String To Number(string=w1039) -> (number=w1035:dbl)  [unwired: 3 in, 1 out]
            n810 = String Subset(string=w1036, length (rest)=3 ("长度（剩余）")) -> (substring=w1038:string)  [unwired: 1 in]
            n811 = case shown="\"UA1\"" w1038 {
              tunnel: w1035 -> [_ w1045 w1048 w1055]
              frame "假", Default {
              }
              frame "USu" {
                n812 = property on="U幅值" class="DigNum (严格)"() -> ("Value"=w1046:sgl)  [unwired: 2 in, 2 out]
                n813 = Subtract(x=w1046, y=w1045) -> (x-y=w1047:dbl)
                n814 = Max & Min(x=w1047, y=sgl 0.0) -> (max(x,y)=w1043:dbl)  [unwired: 1 out]
                n815 = property on="U幅值" class="DigNum (严格)"("Value"=w1043) -> ()  [unwired: 2 in, 2 out]
              }
              frame "ISu" {
                n816 = property on="I幅值" class="DigNum (严格)"() -> ("Value"=w1051:sgl)  [unwired: 2 in, 2 out]
                n817 = Subtract(x=w1051, y=w1048) -> (x-y=w1052:dbl)
                n818 = Max & Min(x=w1052, y=sgl 0.0) -> (max(x,y)=w1049:dbl)  [unwired: 1 out]
                n819 = property on="I幅值" class="DigNum (严格)"("Value"=w1049) -> ()  [unwired: 2 in, 2 out]
              }
              frame "UA1" {
                n820 = property on="UB_amplitude" class="DigNum (严格)"() -> ("Value"=w1057:sgl)  [unwired: 2 in, 2 out]
                n821 = Subtract(x=w1057, y=w1055) -> (x-y=w1056:dbl)
                n822 = Max & Min(x=w1056, y=sgl 0.0) -> (max(x,y)=w1053:dbl)  [unwired: 1 out]
                n823 = property on="UB_amplitude" class="DigNum (严格)"("Value"=w1053) -> ()  [unwired: 2 in, 2 out]
              }
            }
          }
        }
      }
      event "U操作.U启动", "I操作.I启动", "All输出.A启动", "UB_outPut_ctl.UB_outPut_start", "UC_outPut_ctl.UC_outPut_start", "IB_outPut_ctl.IB_outPut_start": Value Change {
        n824 = event-data() -> ("CtlRef"=w1059:refnum<vi>, "NewVal"=w1058:bool)  [unwired: 1 in, 3 out]
        n825 = case shown="真" w1058 {
          tunnel: w1059 -> [_ w1063]
          frame False {
          }
          frame True {
            n826 = property on="vOptios_Tab" class="TabCtl (严格)"() -> ("Value"=w1060:enum32{"电流1", "电流2", "电流3", "电流4"})  [unwired: 2 in, 2 out]
            n827 = property class="Bool (严格)"(reference=w1063) -> (reference out=w1066:refnum<vi>, "Label.Text"=w1061:string)  [unwired: 1 in, 1 out]
            n828 = property on="串口号" class="VISAName"() -> ("Value"=w1062:refnum<visa-resource-name>)  [unwired: 2 in, 2 out]
            n829 = case shown="\"假\", 默认" w1061 {
              tunnel: [w1070 w1155] -> w1065
              tunnel: [w1069 w1154] -> w1064
              tunnel: w1062 -> [w1068 w1155]
              tunnel: w1060 -> [w1067 _]
              frame "假", Default {
                n830 = case shown="\"电流4\"" w1067 {
                  tunnel: [w1073 w1098 w1122 w1145] -> w1069
                  tunnel: w1068 -> [w1072 w1099 w1121 w1144]
                  tunnel: [w1072 w1099 w1121 w1144] -> w1070
                  frame "电流1", Default {
                    n831 = local read "I档位"() -> (w1078:u32)
                    n832 = local read "I幅值"() -> (w1077:sgl)
                    n833 = local read "I纹波"() -> (w1079:sgl)
                    n834 = local read "U档位"() -> (w1075:u32)
                    n835 = local read "U幅值"() -> (w1074:sgl)
                    n836 = local read "U纹波"() -> (w1076:sgl)
                    n837 = local read "U频率"() -> (w1080:sgl)
                    n838 = call "高精度写.vi"("电压幅值"=w1074, "电压纹波"=w1076, "串口号"=w1072, "电压档位"=w1075, "电流幅值"=w1077, "电流档位值"=w1078, "纹波频率"=w1080, "电流纹波"=w1079, "电流通道"=0) -> ("应答"=w1073:string)  [unwired: 6 in]
                  }
                  frame "电流2" {
                    n839 = local read "UB_amplitude"() -> (w1087:sgl)
                    n840 = property on="小信号变比(A/1mv)" class="Clust (严格)"() -> ("Value"=w1094:cluster{"电流2":sgl, "电流3":sgl, "电流4":sgl})  [unwired: 2 in, 2 out]
                    n841 = local read "UB_ripple"() -> (w1083:sgl)
                    n842 = local read "U纹波"() -> (w1091:sgl)
                    n843 = local read "U档位"() -> (w1082:u32)
                    n844 = local read "U幅值"() -> (w1081:sgl)
                    n845 = local read "U频率"() -> (w1097:sgl)
                    n846 = Unbundle(w1094) -> ("电流2"=w1095:sgl)  [unwired: 2 out]
                    n847 = Multiply(x=w1095, y=1000.0) -> (x*y=w1084:dbl)
                    n848 = Divide(x=w1087, y=w1084) -> (x/y=w1086:dbl)
                    n849 = Divide(x=w1083, y=w1084) -> (x/y=w1085:dbl)
                    n850 = Less?(x=5, y=w1086) -> (x < y?=w1088:bool)
                    n851 = case shown="真" w1088 {
                      tunnel: [w1100 w1102] -> w1090
                      tunnel: w1086 -> [w1100 _]
                      tunnel: w1084 -> [_ w1101]
                      frame False {
                      }
                      frame True {
                        w1102 = 5
                        n852 = Multiply(x=w1102, y=w1101) -> (x*y=w1103:dbl)
                        n853 = local write "UB_amplitude"(w1103) -> ()
                      }
                    }
                    n854 = local read "UB_Pos"() -> (w1093:u32)
                    n855 = call "高精度写.vi"("电压幅值"=w1081, "电压纹波"=w1091, "串口号"=w1099, "电压档位"=w1082, "电流幅值"=w1090, "电流档位值"=w1093, "纹波频率"=w1097, "电流纹波"=w1085, "电流通道"=1) -> ("应答"=w1098:string)  [unwired: 6 in]
                  }
                  frame "电流3" {
                    n856 = local read "IB_amplitude"() -> (w1109:sgl)
                    n857 = local read "IB_ripple"() -> (w1107:sgl)
                    n858 = property on="小信号变比(A/1mv)" class="Clust (严格)"() -> ("Value"=w1118:cluster{"电流2":sgl, "电流3":sgl, "电流4":sgl})  [unwired: 2 in, 2 out]
                    n859 = local read "U档位"() -> (w1105:u32)
                    n860 = local read "U幅值"() -> (w1104:sgl)
                    n861 = Unbundle(w1118) -> ("电流3"=w1117:sgl)  [unwired: 2 out]
                    n862 = Multiply(x=w1117, y=1000.0) -> (x*y=w1106:dbl)
                    n863 = local read "U纹波"() -> (w1114:sgl)
                    n864 = Divide(x=w1107, y=w1106) -> (x/y=w1108:dbl)
                    n865 = Divide(x=w1109, y=w1106) -> (x/y=w1110:dbl)
                    n866 = local read "U频率"() -> (w1120:sgl)
                    n867 = Less?(x=5, y=w1110) -> (x < y?=w1113:bool)
                    n868 = case shown="真" w1113 {
                      tunnel: [w1123 w1126] -> w1112
                      tunnel: w1110 -> [w1123 _]
                      tunnel: w1106 -> [_ w1125]
                      frame False {
                      }
                      frame True {
                        w1126 = 5
                        n869 = Multiply(x=w1126, y=w1125) -> (x*y=w1124:dbl)
                        n870 = local write "IB_amplitude"(w1124) -> ()
                      }
                    }
                    n871 = local read "IB_pos"() -> (w1116:u32)
                    n872 = call "高精度写.vi"("电压幅值"=w1104, "电压纹波"=w1114, "串口号"=w1121, "电压档位"=w1105, "电流幅值"=w1112, "电流档位值"=w1116, "纹波频率"=w1120, "电流纹波"=w1108, "电流通道"=2) -> ("应答"=w1122:string)  [unwired: 6 in]
                  }
                  frame "电流4" {
                    # "小信号幅值\n最大输出5v"
                    # "UC"
                    n873 = local read "UC_amplitude"() -> (w1131:sgl)
                    n874 = local read "UC_ripple"() -> (w1133:sgl)
                    n875 = local read "U档位"() -> (w1128:u32)
                    n876 = property on="小信号变比(A/1mv)" class="Clust (严格)"() -> ("Value"=w1134:cluster{"电流2":sgl, "电流3":sgl, "电流4":sgl})  [unwired: 2 in, 2 out]
                    n877 = local read "U幅值"() -> (w1127:sgl)
                    n878 = local read "U纹波"() -> (w1140:sgl)
                    n879 = local read "U频率"() -> (w1143:sgl)
                    n880 = Unbundle(w1134) -> ("电流4"=w1139:sgl)  [unwired: 2 out]
                    n881 = Multiply(x=w1139, y=1000.0) -> (x*y=w1130:dbl)
                    n882 = Divide(x=w1133, y=w1130) -> (x/y=w1129:dbl)
                    n883 = Divide(x=w1131, y=w1130) -> (x/y=w1132:dbl)
                    n884 = Less?(x=5, y=w1132) -> (x < y?=w1136:bool)
                    n885 = case shown="真" w1136 {
                      tunnel: [w1146 w1148] -> w1135
                      tunnel: w1132 -> [w1146 _]
                      tunnel: w1130 -> [_ w1149]
                      frame False {
                      }
                      frame True {
                        w1148 = 5
                        n886 = Multiply(x=w1148, y=w1149) -> (x*y=w1147:dbl)
                        n887 = local write "UC_amplitude"(w1147) -> ()
                      }
                    }
                    n888 = local read "UC_pos"() -> (w1141:u32)
                    n889 = call "高精度写.vi"("电压幅值"=w1127, "电压纹波"=w1140, "串口号"=w1144, "电压档位"=w1128, "电流幅值"=w1135, "电流档位值"=w1141, "纹波频率"=w1143, "电流纹波"=w1129, "电流通道"=3) -> ("应答"=w1145:string)  [unwired: 6 in]
                  }
                }
              }
              frame "U启动" {
                n890 = local read "U档位"() -> (w1153:u32)
                n891 = local read "U幅值"() -> (w1152:sgl)
                n892 = local read "U纹波"() -> (w1151:sgl)
                n893 = local read "U频率"() -> (w1150:sgl)
                n894 = call "高精度写.vi"("电压幅值"=w1152, "电压纹波"=w1151, "串口号"=w1155, "电压档位"=w1153, "纹波频率"=w1150) -> ("应答"=w1154:string)  [unwired: 10 in]
              }
            }
            n895 = case shown="\"正确\"" w1064 {
              tunnel: w1061 -> [_ _ w1162]
              tunnel: w1065 -> [_ _ w1161]
              tunnel: w1066 -> [_ _ w1160]
              frame "错误", Default {
                n896 = property on="提示信息" class="Bool (严格)"("BoolText.Text"="高精度写错误！", "Val(Sgnl)"=TRUE ("提示信息")) -> ()  [unwired: 2 in, 2 out]
              }
              frame "超时" {
                n897 = property on="提示信息" class="Bool (严格)"("BoolText.Text"="高精度写超时！", "Val(Sgnl)"=TRUE ("提示信息")) -> ()  [unwired: 2 in, 2 out]
              }
              frame "正确" {
                n898 = case shown="\"UC_outPut_start\"" w1162 {
                  tunnel: w1161 -> [_ w1166 w1193 w1221 w1261 w1289 w1316]
                  tunnel: w1160 -> [_ _ _ w1219 _ _ _]
                  frame "假", Default {
                    n899 = property on="提示信息" class="Bool (严格)"("BoolText.Text"="启动项错误！", "Val(Sgnl)"=TRUE ("提示信息")) -> ()  [unwired: 2 in, 2 out]
                  }
                  frame "U启动" {
                    w1167 = u16 0 items=["电压启动", "电流启动", "全部启动", "UA1start", "IA1start"] ("启动项")
                    n900 = call "输出启动.vi"("启动项"=w1167, "串口号"=w1166) -> ("应答"=w1165:string)  [unwired: 3 in]
                    n901 = case shown="\"正确\"" w1165 {
                      frame "错误", Default {
                        n902 = property on="提示信息" class="Bool (严格)"("BoolText.Text"="输出失败！", "Val(Sgnl)"=TRUE ("提示信息")) -> ()  [unwired: 2 in, 2 out]
                      }
                      frame "超时" {
                        n903 = property on="提示信息" class="Bool (严格)"("BoolText.Text"="输出超时！", "Val(Sgnl)"=TRUE ("提示信息")) -> ()  [unwired: 2 in, 2 out]
                      }
                      frame "正确" {
                        n904 = for {
                          N: 4 -> [_]
                          i -> [w1173]
                          w1177 = i16 3 ("精度(6)")
                          # "直接取某一列数组"
                          n905 = local read "U幅值"() -> (w1185:sgl)
                          n906 = local read "U纹波"() -> (w1183:sgl)
                          n907 = local read "U频率"() -> (w1182:sgl)
                          n908 = property on="outPut_form" class="Tbl (严格)"() -> ("Value"=w1174:string[][])  [unwired: 2 in, 2 out]
                          n909 = Number To Fractional String(number=w1185, precision (6)=w1177) -> (F-format string=w1184:string)  [unwired: 2 in]
                          n910 = Number To Fractional String(number=w1183, precision (6)=w1177) -> (F-format string=w1181:string)  [unwired: 2 in]
                          n911 = Number To Fractional String(number=w1182, precision (6)=w1177) -> (F-format string=w1180:string)  [unwired: 2 in]
                          n912 = Index Array(array=w1174, index (col)=w1173) -> (element=w1191:string[])  [unwired: 1 in]
                          n913 = Replace Array Subset(array=w1191, new element=w1184, index=0 ("索引")) -> (w1188:string[])
                          n914 = Replace Array Subset(array=w1188, new element=w1181, index=2 ("索引")) -> (w1186:string[])
                          n915 = Replace Array Subset(array=w1186, new element=w1180, index=4 ("索引")) -> (w1179:string[])
                          n916 = Replace Array Subset(array=w1174, new element=w1179, index (col)=w1173) -> (w1175:string[][])  [unwired: 1 in]
                          n917 = property on="控制选项卡" class="TabCtl (严格)"("PageSelVis"=FALSE ("页选择器可见")) -> ()  [unwired: 2 in, 2 out]
                          n918 = property on="outPut_form" class="Tbl (严格)"("Value"=w1175) -> ()  [unwired: 2 in, 2 out]
                          n919 = property on="U状态" class="Bool (严格)"("Value"=TRUE ("输出状态")) -> ()  [unwired: 2 in, 2 out]
                        }
                      }
                    }
                  }
                  frame "I启动" {
                    w1194 = u16 1 items=["电压启动", "电流启动", "全部启动"] ("启动项")
                    n920 = call "输出启动.vi"("启动项"=w1194, "串口号"=w1193) -> ("应答"=w1192:string)  [unwired: 3 in]
                    n921 = case shown="\"正确\"" w1192 {
                      frame "错误", Default {
                        n922 = property on="提示信息" class="Bool (严格)"("BoolText.Text"="输出失败！", "Val(Sgnl)"=TRUE ("提示信息")) -> ()  [unwired: 2 in, 2 out]
                      }
                      frame "超时" {
                        n923 = property on="提示信息" class="Bool (严格)"("BoolText.Text"="输出超时！", "Val(Sgnl)"=TRUE ("提示信息")) -> ()  [unwired: 2 in, 2 out]
                      }
                      frame "正确" {
                        w1205 = i16 3 ("精度(6)")
                        n924 = local read "I纹波"() -> (w1200:sgl)
                        n925 = local read "U频率"() -> (w1199:sgl)
                        n926 = local read "I幅值"() -> (w1213:sgl)
                        n927 = property on="outPut_form" class="Tbl (严格)"() -> ("Value"=w1207:string[][])  [unwired: 2 in, 2 out]
                        n928 = Number To Fractional String(number=w1213, precision (6)=w1205) -> (F-format string=w1212:string)  [unwired: 2 in]
                        n929 = Number To Fractional String(number=w1200, precision (6)=w1205) -> (F-format string=w1211:string)  [unwired: 2 in]
                        n930 = Number To Fractional String(number=w1199, precision (6)=w1205) -> (F-format string=w1204:string)  [unwired: 2 in]
                        n931 = Index Array(array=w1207, index (col)=0 ("禁用的索引 (列)")) -> (element=w1217:string[])  [unwired: 1 in]
                        n932 = Replace Array Subset(array=w1217, new element=w1212, index=1 ("索引")) -> (w1214:string[])
                        n933 = Replace Array Subset(array=w1214, new element=w1211, index=3 ("索引")) -> (w1202:string[])
                        n934 = Replace Array Subset(array=w1202, new element=w1204, index=4 ("索引")) -> (w1201:string[])
                        n935 = Replace Array Subset(array=w1207, new element=w1201, index (col)=0 ("禁用的索引 (列)")) -> (w1206:string[][])  [unwired: 1 in]
                        n936 = property on="控制选项卡" class="TabCtl (严格)"("PageSelVis"=FALSE ("页选择器可见")) -> ()  [unwired: 2 in, 2 out]
                        n937 = property on="outPut_form" class="Tbl (严格)"("Value"=w1206) -> ()  [unwired: 2 in, 2 out]
                        n938 = property on="I状态" class="Bool (严格)"("Value"=TRUE ("输出状态")) -> ()  [unwired: 2 in, 2 out]
                      }
                    }
                  }
                  frame "A启动" {
                    w1222 = u16 2 items=["电压启动", "电流启动", "全部启动"] ("启动项")
                    n939 = call "输出启动.vi"("启动项"=w1222, "串口号"=w1221) -> ("应答"=w1220:string)  [unwired: 3 in]
                    n940 = case shown="\"正确\"" w1220 {
                      tunnel: w1219 -> [w1225 w1228 _]
                      frame "错误", Default {
                        n941 = property class="Bool (严格)"(reference=w1225, "Value"=FALSE ("值")) -> ()  [unwired: 1 in, 2 out]
                        n942 = property on="提示信息" class="Bool (严格)"("BoolText.Text"="输出失败！", "Val(Sgnl)"=TRUE ("提示信息")) -> ()  [unwired: 2 in, 2 out]
                        n943 = property on="控制选项卡" class="TabCtl (严格)"("PageSelVis"=FALSE ("页选择器可见")) -> ()  [unwired: 2 in, 2 out]
                      }
                      frame "超时" {
                        n944 = property class="Bool (严格)"(reference=w1228, "Value"=FALSE ("值")) -> ()  [unwired: 1 in, 2 out]
                        n945 = property on="提示信息" class="Bool (严格)"("BoolText.Text"="输出超时！", "Val(Sgnl)"=TRUE ("提示信息")) -> ()  [unwired: 2 in, 2 out]
                      }
                      frame "正确" {
                        w1235 = i16 3 ("精度(6)")
                        n946 = local read "U幅值"() -> (w1253:sgl)
                        n947 = local read "U纹波"() -> (w1250:sgl)
                        n948 = local read "U频率"() -> (w1245:sgl)
                        n949 = local read "I幅值"() -> (w1251:sgl)
                        n950 = local read "I纹波"() -> (w1243:sgl)
                        n951 = property on="outPut_form" class="Tbl (严格)"() -> ("Value"=w1232:string[][])  [unwired: 2 in, 2 out]
                        n952 = property on="U状态" class="Bool (严格)"("Value"=TRUE ("输出状态")) -> ()  [unwired: 2 in, 2 out]
                        n953 = Number To Fractional String(number=w1253, precision (6)=w1235) -> (F-format string=w1252:string)  [unwired: 2 in]
                        n954 = Number To Fractional String(number=w1251, precision (6)=w1235) -> (F-format string=w1249:string)  [unwired: 2 in]
                        n955 = Number To Fractional String(number=w1250, precision (6)=w1235) -> (F-format string=w1248:string)  [unwired: 2 in]
                        n956 = Number To Fractional String(number=w1243, precision (6)=w1235) -> (F-format string=w1244:string)  [unwired: 2 in]
                        n957 = Number To Fractional String(number=w1245, precision (6)=w1235) -> (F-format string=w1246:string)  [unwired: 2 in]
                        n958 = property on="I状态" class="Bool (严格)"("Value"=TRUE ("输出状态")) -> ()  [unwired: 2 in, 2 out]
                        n959 = Index Array(array=w1232, index (col)=0 ("禁用的索引 (列)")) -> (element=w1259:string[])  [unwired: 1 in]
                        n960 = Replace Array Subset(array=w1259, new element=w1252, index=0 ("索引")) -> (w1256:string[])
                        n961 = Replace Array Subset(array=w1256, new element=w1249, index=1 ("索引")) -> (w1254:string[])
                        n962 = Replace Array Subset(array=w1254, new element=w1248, index=2 ("索引")) -> (w1239:string[])
                        n963 = Replace Array Subset(array=w1239, new element=w1244, index=3 ("索引")) -> (w1242:string[])
                        n964 = Replace Array Subset(array=w1242, new element=w1246, index=4 ("索引")) -> (w1238:string[])
                        n965 = property on="控制选项卡" class="TabCtl (严格)"("PageSelVis"=FALSE ("页选择器可见")) -> ()  [unwired: 2 in, 2 out]
                        n966 = Replace Array Subset(array=w1232, new element=w1238, index (col)=0 ("禁用的索引 (列)")) -> (w1233:string[][])  [unwired: 1 in]
                        n967 = property on="outPut_form" class="Tbl (严格)"("Value"=w1233) -> ()  [unwired: 2 in, 2 out]
                      }
                    }
                  }
                  frame "UB_outPut_start" {
                    w1263 = u16 3 items=["电压启动", "电流启动", "全部启动", "UB_outPut_start", "IB_outPut_start", "UC_outPut_start"] ("启动项")
                    n968 = call "输出启动.vi"("启动项"=w1263, "串口号"=w1261) -> ("应答"=w1262:string)  [unwired: 3 in]
                    n969 = case shown="\"正确\"" w1262 {
                      frame "错误", Default {
                        n970 = property on="提示信息" class="Bool (严格)"("BoolText.Text"="输出失败！", "Val(Sgnl)"=TRUE ("提示信息")) -> ()  [unwired: 2 in, 2 out]
                      }
                      frame "超时" {
                        n971 = property on="提示信息" class="Bool (严格)"("BoolText.Text"="输出超时！", "Val(Sgnl)"=TRUE ("提示信息")) -> ()  [unwired: 2 in, 2 out]
                      }
                      frame "正确" {
                        w1270 = i16 3 ("精度(6)")
                        n972 = local read "UB_ripple"() -> (w1269:sgl)
                        n973 = local read "UB_amplitude"() -> (w1275:sgl)
                        n974 = local read "U频率"() -> (w1268:sgl)
                        n975 = property on="outPut_form" class="Tbl (严格)"() -> ("Value"=w1276:string[][])  [unwired: 2 in, 2 out]
                        n976 = Number To Fractional String(number=w1275, precision (6)=w1270) -> (F-format string=w1282:string)  [unwired: 2 in]
                        n977 = Number To Fractional String(number=w1268, precision (6)=w1270) -> (F-format string=w1274:string)  [unwired: 2 in]
                        n978 = Number To Fractional String(number=w1269, precision (6)=w1270) -> (F-format string=w1281:string)  [unwired: 2 in]
                        n979 = Index Array(array=w1276, index (col)=1 ("禁用的索引 (列)")) -> (element=w1286:string[])  [unwired: 1 in]
                        n980 = Replace Array Subset(array=w1286, new element=w1282, index=1 ("索引")) -> (w1283:string[])
                        n981 = Replace Array Subset(array=w1283, new element=w1281, index=3 ("索引")) -> (w1272:string[])
                        n982 = Replace Array Subset(array=w1272, new element=w1274, index=4 ("索引")) -> (w1271:string[])
                        n983 = Replace Array Subset(array=w1276, new element=w1271, index (col)=1 ("禁用的索引 (列)")) -> (w1277:string[][])  [unwired: 1 in]
                        n984 = property on="控制选项卡" class="TabCtl (严格)"("PageSelVis"=FALSE ("页选择器可见")) -> ()  [unwired: 2 in, 2 out]
                        n985 = property on="UB_status" class="Bool (严格)"("Value"=TRUE ("输出状态")) -> ()  [unwired: 2 in, 2 out]
                        n986 = property on="outPut_form" class="Tbl (严格)"("Value"=w1277) -> ()  [unwired: 2 in, 2 out]
                      }
                    }
                  }
                  frame "IB_outPut_start" {
                    w1288 = u16 4 items=["电压启动", "电流启动", "全部启动", "UB_outPut_start", "IB_outPut_start", "UC_outPut_start"] ("启动项")
                    n987 = call "输出启动.vi"("启动项"=w1288, "串口号"=w1289) -> ("应答"=w1290:string)  [unwired: 3 in]
                    n988 = case shown="\"正确\"" w1290 {
                      frame "错误", Default {
                        n989 = property on="提示信息" class="Bool (严格)"("BoolText.Text"="输出失败！", "Val(Sgnl)"=TRUE ("提示信息")) -> ()  [unwired: 2 in, 2 out]
                      }
                      frame "超时" {
                        n990 = property on="提示信息" class="Bool (严格)"("BoolText.Text"="输出超时！", "Val(Sgnl)"=TRUE ("提示信息")) -> ()  [unwired: 2 in, 2 out]
                      }
                      frame "正确" {
                        w1299 = i16 3 ("精度(6)")
                        n991 = local read "U频率"() -> (w1295:sgl)
                        n992 = local read "IB_amplitude"() -> (w1305:sgl)
                        n993 = local read "IB_ripple"() -> (w1296:sgl)
                        n994 = Number To Fractional String(number=w1295, precision (6)=w1299) -> (F-format string=w1301:string)  [unwired: 2 in]
                        n995 = property on="outPut_form" class="Tbl (严格)"() -> ("Value"=w1302:string[][])  [unwired: 2 in, 2 out]
                        n996 = Number To Fractional String(number=w1305, precision (6)=w1299) -> (F-format string=w1309:string)  [unwired: 2 in]
                        n997 = Number To Fractional String(number=w1296, precision (6)=w1299) -> (F-format string=w1308:string)  [unwired: 2 in]
                        n998 = Index Array(array=w1302, index (col)=2 ("禁用的索引 (列)")) -> (element=w1313:string[])  [unwired: 1 in]
                        n999 = Replace Array Subset(array=w1313, new element=w1309, index=1 ("索引")) -> (w1310:string[])
                        n1000 = Replace Array Subset(array=w1310, new element=w1308, index=3 ("索引")) -> (w1298:string[])
                        n1001 = Replace Array Subset(array=w1298, new element=w1301, index=4 ("索引")) -> (w1297:string[])
                        n1002 = Replace Array Subset(array=w1302, new element=w1297, index (col)=2 ("禁用的索引 (列)")) -> (w1303:string[][])  [unwired: 1 in]
                        n1003 = property on="控制选项卡" class="TabCtl (严格)"("PageSelVis"=FALSE ("页选择器可见")) -> ()  [unwired: 2 in, 2 out]
                        n1004 = property on="IB_status" class="Bool (严格)"("Value"=TRUE ("输出状态")) -> ()  [unwired: 2 in, 2 out]
                        n1005 = property on="outPut_form" class="Tbl (严格)"("Value"=w1303) -> ()  [unwired: 2 in, 2 out]
                      }
                    }
                  }
                  frame "UC_outPut_start" {
                    w1315 = u16 5 items=["电压启动", "电流启动", "全部启动", "UB_outPut_start", "IB_outPut_start", "UC_outPut_start"] ("启动项")
                    n1006 = call "输出启动.vi"("启动项"=w1315, "串口号"=w1316) -> ("应答"=w1317:string)  [unwired: 3 in]
                    n1007 = case shown="\"正确\"" w1317 {
                      frame "错误", Default {
                        n1008 = property on="提示信息" class="Bool (严格)"("BoolText.Text"="输出失败！", "Val(Sgnl)"=TRUE ("提示信息")) -> ()  [unwired: 2 in, 2 out]
                      }
                      frame "超时" {
                        n1009 = property on="提示信息" class="Bool (严格)"("BoolText.Text"="输出超时！", "Val(Sgnl)"=TRUE ("提示信息")) -> ()  [unwired: 2 in, 2 out]
                      }
                      frame "正确" {
                        w1326 = i16 3 ("精度(6)")
                        n1010 = local read "UC_amplitude"() -> (w1332:sgl)
                        n1011 = local read "UC_ripple"() -> (w1323:sgl)
                        n1012 = local read "U频率"() -> (w1322:sgl)
                        n1013 = property on="控制选项卡" class="TabCtl (严格)"("PageSelVis"=FALSE ("页选择器可见")) -> ()  [unwired: 2 in, 2 out]
                        n1014 = property on="outPut_form" class="Tbl (严格)"() -> ("Value"=w1329:string[][])  [unwired: 2 in, 2 out]
                        n1015 = Number To Fractional String(number=w1322, precision (6)=w1326) -> (F-format string=w1328:string)  [unwired: 2 in]
                        n1016 = Number To Fractional String(number=w1332, precision (6)=w1326) -> (F-format string=w1336:string)  [unwired: 2 in]
                        n1017 = Number To Fractional String(number=w1323, precision (6)=w1326) -> (F-format string=w1335:string)  [unwired: 2 in]
                        n1018 = Index Array(array=w1329, index (col)=3 ("禁用的索引 (列)")) -> (element=w1340:string[])  [unwired: 1 in]
                        n1019 = Replace Array Subset(array=w1340, new element=w1336, index=1 ("索引")) -> (w1337:string[])
                        n1020 = Replace Array Subset(array=w1337, new element=w1335, index=3 ("索引")) -> (w1325:string[])
                        n1021 = Replace Array Subset(array=w1325, new element=w1328, index=4 ("索引")) -> (w1324:string[])
                        n1022 = Replace Array Subset(array=w1329, new element=w1324, index (col)=3 ("禁用的索引 (列)")) -> (w1330:string[][])  [unwired: 1 in]
                        n1023 = property on="UC_status" class="Bool (严格)"("Value"=TRUE ("输出状态")) -> ()  [unwired: 2 in, 2 out]
                        n1024 = property on="outPut_form" class="Tbl (严格)"("Value"=w1330) -> ()  [unwired: 2 in, 2 out]
                      }
                    }
                  }
                }
              }
            }
          }
        }
      }
      event "U操作.U停止", "I操作.I停止", "All输出.A停止", "UB_outPut_ctl.UB_outPut_stop", "UC_outPut_ctl.UC_outPut_stop", "IB_outPut_ctl.IB_outPut_stop": Value Change {
        n1025 = event-data() -> ("CtlRef"=w1343:refnum<vi>, "NewVal"=w1342:bool)  [unwired: 1 in, 3 out]
        n1026 = case shown="真" w1342 {
          tunnel: w1343 -> [_ w1346]
          frame False {
          }
          frame True {
            n1027 = property class="Bool (严格)"(reference=w1346) -> ("Label.Text"=w1345:string)  [unwired: 1 in, 2 out]
            n1028 = property on="串口号" class="VISAName"() -> ("Value"=w1344:refnum<visa-resource-name>)  [unwired: 2 in, 2 out]
            n1029 = case shown="\"A停止\"" w1345 {
              tunnel: w1344 -> [_ w1350 w1375 w1400 w1431 w1462 w1493]
              frame "假", Default {
                n1030 = property on="提示信息" class="Bool (严格)"("BoolText.Text"="停止项错误！", "Val(Sgnl)"=TRUE ("提示信息")) -> ()  [unwired: 2 in, 2 out]
              }
              frame "U停止" {
                w1351 = u16 0 items=["电压停止", "电流停止", "全部停止"] ("启动项")
                n1031 = call "输出停止.vi"("启动项"=w1351, "串口号"=w1350) -> ("应答"=w1349:string)  [unwired: 3 in]
                n1032 = case shown="\"正确\"" w1349 {
                  frame "错误", Default {
                    n1033 = property on="提示信息" class="Bool (严格)"("BoolText.Text"="停止失败！", "Val(Sgnl)"=TRUE ("提示信息")) -> ()  [unwired: 2 in, 2 out]
                  }
                  frame "超时" {
                    n1034 = property on="提示信息" class="Bool (严格)"("BoolText.Text"="输出超时！", "Val(Sgnl)"=TRUE ("提示信息")) -> ()  [unwired: 2 in, 2 out]
                  }
                  frame "正确" {
                    w1359 = sgl 0.0 ("数字")
                    w1357 = i16 3 ("精度(6)")
                    n1035 = property on="U状态" class="Bool (严格)"("Value"=FALSE ("输出状态")) -> ()  [unwired: 2 in, 2 out]
                    n1036 = Number To Fractional String(number=w1359, precision (6)=w1357) -> (F-format string=w1365:string)  [unwired: 2 in]
                    n1037 = Number To Fractional String(number=w1359, precision (6)=w1357) -> (F-format string=w1364:string)  [unwired: 2 in]
                    n1038 = Number To Fractional String(number=w1359, precision (6)=w1357) -> (F-format string=w1363:string)  [unwired: 2 in]
                    n1039 = property on="本机表格" class="Tbl (严格)"() -> ("Value"=w1373:string[][])  [unwired: 2 in, 2 out]
                    n1040 = Index Array(array=w1373, index (col)=0 ("禁用的索引 (列)")) -> (element=w1371:string[])  [unwired: 1 in]
                    n1041 = Replace Array Subset(array=w1371, new element=w1365, index=0 ("索引")) -> (w1368:string[])
                    n1042 = Replace Array Subset(array=w1368, new element=w1364, index=2 ("索引")) -> (w1366:string[])
                    n1043 = Replace Array Subset(array=w1366, new element=w1363, index=4 ("索引")) -> (w1361:string[])
                    n1044 = Replace Array Subset(array=w1373, new element=w1361, index (col)=0 ("禁用的索引 (列)")) -> (w1360:string[][])  [unwired: 1 in]
                    n1045 = property on="本机表格" class="Tbl (严格)"("Value"=w1360) -> ()  [unwired: 2 in, 2 out]
                    n1046 = property on="控制选项卡" class="TabCtl (严格)"("PageSelVis"=TRUE ("页选择器可见")) -> ()  [unwired: 2 in, 2 out]
                  }
                }
              }
              frame "I停止" {
                w1376 = u16 1 items=["电压停止", "电流停止", "全部停止"] ("启动项")
                n1047 = call "输出停止.vi"("启动项"=w1376, "串口号"=w1375) -> ("应答"=w1374:string)  [unwired: 3 in]
                n1048 = case shown="\"正确\"" w1374 {
                  frame "错误", Default {
                    n1049 = property on="提示信息" class="Bool (严格)"("BoolText.Text"="停止失败！", "Val(Sgnl)"=TRUE ("提示信息")) -> ()  [unwired: 2 in, 2 out]
                  }
                  frame "超时" {
                    n1050 = property on="提示信息" class="Bool (严格)"("BoolText.Text"="输出超时！", "Val(Sgnl)"=TRUE ("提示信息")) -> ()  [unwired: 2 in, 2 out]
                  }
                  frame "正确" {
                    w1384 = sgl 0.0 ("数字")
                    w1382 = i16 3 ("精度(6)")
                    n1051 = Number To Fractional String(number=w1384, precision (6)=w1382) -> (F-format string=w1390:string)  [unwired: 2 in]
                    n1052 = Number To Fractional String(number=w1384, precision (6)=w1382) -> (F-format string=w1389:string)  [unwired: 2 in]
                    n1053 = Number To Fractional String(number=w1384, precision (6)=w1382) -> (F-format string=w1388:string)  [unwired: 2 in]
                    n1054 = property on="本机表格" class="Tbl (严格)"() -> ("Value"=w1398:string[][])  [unwired: 2 in, 2 out]
                    n1055 = property on="I状态" class="Bool (严格)"("Value"=FALSE ("输出状态")) -> ()  [unwired: 2 in, 2 out]
                    n1056 = Index Array(array=w1398, index (col)=0 ("禁用的索引 (列)")) -> (element=w1396:string[])  [unwired: 1 in]
                    n1057 = Replace Array Subset(array=w1396, new element=w1390, index=1 ("索引")) -> (w1393:string[])
                    n1058 = Replace Array Subset(array=w1393, new element=w1389, index=3 ("索引")) -> (w1391:string[])
                    n1059 = Replace Array Subset(array=w1391, new element=w1388, index=4 ("索引")) -> (w1386:string[])
                    n1060 = Replace Array Subset(array=w1398, new element=w1386, index (col)=0 ("禁用的索引 (列)")) -> (w1385:string[][])  [unwired: 1 in]
                    n1061 = property on="本机表格" class="Tbl (严格)"("Value"=w1385) -> ()  [unwired: 2 in, 2 out]
                    n1062 = property on="控制选项卡" class="TabCtl (严格)"("PageSelVis"=TRUE ("页选择器可见")) -> ()  [unwired: 2 in, 2 out]
                  }
                }
              }
              frame "A停止" {
                w1401 = u16 2 items=["电压停止", "电流停止", "全部停止"] ("启动项")
                n1063 = call "输出停止.vi"("启动项"=w1401, "串口号"=w1400) -> ("应答"=w1399:string)  [unwired: 3 in]
                n1064 = case shown="\"正确\"" w1399 {
                  frame "错误", Default {
                    n1065 = property on="提示信息" class="Bool (严格)"("BoolText.Text"="停止失败！", "Val(Sgnl)"=TRUE ("提示信息")) -> ()  [unwired: 2 in, 2 out]
                  }
                  frame "超时" {
                    n1066 = property on="提示信息" class="Bool (严格)"("BoolText.Text"="输出超时！", "Val(Sgnl)"=TRUE ("提示信息")) -> ()  [unwired: 2 in, 2 out]
                  }
                  frame "正确" {
                    w1410 = sgl 0.0 ("数字")
                    w1407 = i16 3 ("精度(6)")
                    n1067 = property on="U状态" class="Bool (严格)"("Value"=FALSE ("输出状态")) -> ()  [unwired: 2 in, 2 out]
                    n1068 = Number To Fractional String(number=w1410, precision (6)=w1407) -> (F-format string=w1422:string)  [unwired: 2 in]
                    n1069 = Number To Fractional String(number=w1410, precision (6)=w1407) -> (F-format string=w1421:string)  [unwired: 2 in]
                    n1070 = Number To Fractional String(number=w1410, precision (6)=w1407) -> (F-format string=w1420:string)  [unwired: 2 in]
                    n1071 = Number To Fractional String(number=w1410, precision (6)=w1407) -> (F-format string=w1416:string)  [unwired: 2 in]
                    n1072 = Number To Fractional String(number=w1410, precision (6)=w1407) -> (F-format string=w1417:string)  [unwired: 2 in]
                    n1073 = property on="I状态" class="Bool (严格)"("Value"=FALSE ("输出状态")) -> ()  [unwired: 2 in, 2 out]
                    n1074 = property on="本机表格" class="Tbl (严格)"() -> ("Value"=w1430:string[][])  [unwired: 2 in, 2 out]
                    n1075 = Index Array(array=w1430, index (col)=0 ("禁用的索引 (列)")) -> (element=w1428:string[])  [unwired: 1 in]
                    n1076 = Replace Array Subset(array=w1428, new element=w1422, index=0 ("索引")) -> (w1425:string[])
                    n1077 = Replace Array Subset(array=w1425, new element=w1421, index=1 ("索引")) -> (w1423:string[])
                    n1078 = Replace Array Subset(array=w1423, new element=w1420, index=2 ("索引")) -> (w1412:string[])
                    n1079 = Replace Array Subset(array=w1412, new element=w1416, index=3 ("索引")) -> (w1415:string[])
                    n1080 = Replace Array Subset(array=w1415, new element=w1417, index=4 ("索引")) -> (w1411:string[])
                    n1081 = Replace Array Subset(array=w1430, new element=w1411, index (col)=0 ("禁用的索引 (列)")) -> (w1418:string[][])  [unwired: 1 in]
                    n1082 = property on="本机表格" class="Tbl (严格)"("Value"=w1418) -> ()  [unwired: 2 in, 2 out]
                    n1083 = property on="控制选项卡" class="TabCtl (严格)"("PageSelVis"=TRUE ("页选择器可见")) -> ()  [unwired: 2 in, 2 out]
                  }
                }
              }
              frame "UB_outPut_stop" {
                w1433 = u16 3 items=["电压停止", "电流停止", "全部停止", "UB_outPut_stop", "IB_outPut_stop", "UC_outPut_stop", ""] ("启动项")
                n1084 = call "输出停止.vi"("启动项"=w1433, "串口号"=w1431) -> ("应答"=w1432:string)  [unwired: 3 in]
                n1085 = case shown="\"正确\"" w1432 {
                  frame "错误", Default {
                    n1086 = property on="提示信息" class="Bool (严格)"("BoolText.Text"="停止失败！", "Val(Sgnl)"=TRUE ("提示信息")) -> ()  [unwired: 2 in, 2 out]
                  }
                  frame "超时" {
                    n1087 = property on="提示信息" class="Bool (严格)"("BoolText.Text"="输出超时！", "Val(Sgnl)"=TRUE ("提示信息")) -> ()  [unwired: 2 in, 2 out]
                  }
                  frame "正确" {
                    w1441 = sgl 0.0 ("数字")
                    w1440 = i16 3 ("精度(6)")
                    n1088 = property on="UB_status" class="Bool (严格)"("Value"=FALSE ("输出状态")) -> ()  [unwired: 2 in, 2 out]
                    n1089 = Number To Fractional String(number=w1441, precision (6)=w1440) -> (F-format string=w1453:string)  [unwired: 2 in]
                    n1090 = Number To Fractional String(number=w1441, precision (6)=w1440) -> (F-format string=w1452:string)  [unwired: 2 in]
                    n1091 = Number To Fractional String(number=w1441, precision (6)=w1440) -> (F-format string=w1451:string)  [unwired: 2 in]
                    n1092 = Number To Fractional String(number=w1441, precision (6)=w1440) -> (F-format string=w1447:string)  [unwired: 2 in]
                    n1093 = Number To Fractional String(number=w1441, precision (6)=w1440) -> (F-format string=w1448:string)  [unwired: 2 in]
                    n1094 = property on="本机表格" class="Tbl (严格)"() -> ("Value"=w1461:string[][])  [unwired: 2 in, 2 out]
                    n1095 = Index Array(array=w1461, index (col)=0 ("禁用的索引 (列)")) -> (element=w1459:string[])  [unwired: 1 in]
                    n1096 = Replace Array Subset(array=w1459, new element=w1453, index=0 ("索引")) -> (w1456:string[])
                    n1097 = Replace Array Subset(array=w1456, new element=w1452, index=1 ("索引")) -> (w1454:string[])
                    n1098 = Replace Array Subset(array=w1454, new element=w1451, index=2 ("索引")) -> (w1443:string[])
                    n1099 = Replace Array Subset(array=w1443, new element=w1447, index=3 ("索引")) -> (w1446:string[])
                    n1100 = Replace Array Subset(array=w1446, new element=w1448, index=4 ("索引")) -> (w1442:string[])
                    n1101 = Replace Array Subset(array=w1461, new element=w1442, index (col)=0 ("禁用的索引 (列)")) -> (w1449:string[][])  [unwired: 1 in]
                    n1102 = property on="本机表格" class="Tbl (严格)"("Value"=w1449) -> ()  [unwired: 2 in, 2 out]
                    n1103 = property on="控制选项卡" class="TabCtl (严格)"("PageSelVis"=TRUE ("页选择器可见")) -> ()  [unwired: 2 in, 2 out]
                  }
                }
              }
              frame "IB_outPut_stop" {
                w1464 = u16 4 items=["电压停止", "电流停止", "全部停止", "UB_outPut_stop", "IB_outPut_stop", "UC_outPut_stop"] ("启动项")
                n1104 = call "输出停止.vi"("启动项"=w1464, "串口号"=w1462) -> ("应答"=w1463:string)  [unwired: 3 in]
                n1105 = case shown="\"正确\"" w1463 {
                  frame "错误", Default {
                    n1106 = property on="提示信息" class="Bool (严格)"("BoolText.Text"="停止失败！", "Val(Sgnl)"=TRUE ("提示信息")) -> ()  [unwired: 2 in, 2 out]
                  }
                  frame "超时" {
                    n1107 = property on="提示信息" class="Bool (严格)"("BoolText.Text"="输出超时！", "Val(Sgnl)"=TRUE ("提示信息")) -> ()  [unwired: 2 in, 2 out]
                  }
                  frame "正确" {
                    w1472 = sgl 0.0 ("数字")
                    w1471 = i16 3 ("精度(6)")
                    n1108 = Number To Fractional String(number=w1472, precision (6)=w1471) -> (F-format string=w1484:string)  [unwired: 2 in]
                    n1109 = Number To Fractional String(number=w1472, precision (6)=w1471) -> (F-format string=w1483:string)  [unwired: 2 in]
                    n1110 = Number To Fractional String(number=w1472, precision (6)=w1471) -> (F-format string=w1482:string)  [unwired: 2 in]
                    n1111 = Number To Fractional String(number=w1472, precision (6)=w1471) -> (F-format string=w1478:string)  [unwired: 2 in]
                    n1112 = Number To Fractional String(number=w1472, precision (6)=w1471) -> (F-format string=w1479:string)  [unwired: 2 in]
                    n1113 = property on="本机表格" class="Tbl (严格)"() -> ("Value"=w1492:string[][])  [unwired: 2 in, 2 out]
                    n1114 = Index Array(array=w1492, index (col)=0 ("禁用的索引 (列)")) -> (element=w1490:string[])  [unwired: 1 in]
                    n1115 = Replace Array Subset(array=w1490, new element=w1484, index=0 ("索引")) -> (w1487:string[])
                    n1116 = Replace Array Subset(array=w1487, new element=w1483, index=1 ("索引")) -> (w1485:string[])
                    n1117 = Replace Array Subset(array=w1485, new element=w1482, index=2 ("索引")) -> (w1474:string[])
                    n1118 = Replace Array Subset(array=w1474, new element=w1478, index=3 ("索引")) -> (w1477:string[])
                    n1119 = Replace Array Subset(array=w1477, new element=w1479, index=4 ("索引")) -> (w1473:string[])
                    n1120 = Replace Array Subset(array=w1492, new element=w1473, index (col)=0 ("禁用的索引 (列)")) -> (w1480:string[][])  [unwired: 1 in]
                    n1121 = property on="本机表格" class="Tbl (严格)"("Value"=w1480) -> ()  [unwired: 2 in, 2 out]
                    n1122 = property on="控制选项卡" class="TabCtl (严格)"("PageSelVis"=TRUE ("页选择器可见")) -> ()  [unwired: 2 in, 2 out]
                    n1123 = property on="IB_status" class="Bool (严格)"("Value"=FALSE ("输出状态")) -> ()  [unwired: 2 in, 2 out]
                  }
                }
              }
              frame "UC_outPut_stop" {
                w1495 = u16 5 items=["电压停止", "电流停止", "全部停止", "UB_outPut_stop", "IB_outPut_stop", "UC_outPut_stop"] ("启动项")
                n1124 = call "输出停止.vi"("启动项"=w1495, "串口号"=w1493) -> ("应答"=w1494:string)  [unwired: 3 in]
                n1125 = case shown="\"正确\"" w1494 {
                  frame "错误", Default {
                    n1126 = property on="提示信息" class="Bool (严格)"("BoolText.Text"="停止失败！", "Val(Sgnl)"=TRUE ("提示信息")) -> ()  [unwired: 2 in, 2 out]
                  }
                  frame "超时" {
                    n1127 = property on="提示信息" class="Bool (严格)"("BoolText.Text"="输出超时！", "Val(Sgnl)"=TRUE ("提示信息")) -> ()  [unwired: 2 in, 2 out]
                  }
                  frame "正确" {
                    w1500 = FALSE ("输出状态")
                    w1503 = sgl 0.0 ("数字")
                    w1502 = i16 3 ("精度(6)")
                    n1128 = Number To Fractional String(number=w1503, precision (6)=w1502) -> (F-format string=w1515:string)  [unwired: 2 in]
                    n1129 = Number To Fractional String(number=w1503, precision (6)=w1502) -> (F-format string=w1514:string)  [unwired: 2 in]
                    n1130 = Number To Fractional String(number=w1503, precision (6)=w1502) -> (F-format string=w1513:string)  [unwired: 2 in]
                    n1131 = Number To Fractional String(number=w1503, precision (6)=w1502) -> (F-format string=w1509:string)  [unwired: 2 in]
                    n1132 = Number To Fractional String(number=w1503, precision (6)=w1502) -> (F-format string=w1510:string)  [unwired: 2 in]
                    n1133 = property on="本机表格" class="Tbl (严格)"() -> ("Value"=w1523:string[][])  [unwired: 2 in, 2 out]
                    n1134 = Index Array(array=w1523, index (col)=0 ("禁用的索引 (列)")) -> (element=w1521:string[])  [unwired: 1 in]
                    n1135 = Replace Array Subset(array=w1521, new element=w1515, index=0 ("索引")) -> (w1518:string[])
                    n1136 = Replace Array Subset(array=w1518, new element=w1514, index=1 ("索引")) -> (w1516:string[])
                    n1137 = Replace Array Subset(array=w1516, new element=w1513, index=2 ("索引")) -> (w1505:string[])
                    n1138 = Replace Array Subset(array=w1505, new element=w1509, index=3 ("索引")) -> (w1508:string[])
                    n1139 = Replace Array Subset(array=w1508, new element=w1510, index=4 ("索引")) -> (w1504:string[])
                    n1140 = Replace Array Subset(array=w1523, new element=w1504, index (col)=0 ("禁用的索引 (列)")) -> (w1511:string[][])  [unwired: 1 in]
                    n1141 = property on="本机表格" class="Tbl (严格)"("Value"=w1511) -> ()  [unwired: 2 in, 2 out]
                    n1142 = property on="控制选项卡" class="TabCtl (严格)"("PageSelVis"=TRUE ("页选择器可见")) -> ()  [unwired: 2 in, 2 out]
                    n1143 = property on="UC_outPut_stop" class="Bool (严格)"("Value"=w1500) -> ()  [unwired: 2 in, 2 out]
                    n1144 = property on="UC_status" class="Bool (严格)"("Value"=w1500) -> ()  [unwired: 2 in, 2 out]
                  }
                }
              }
            }
          }
        }
      }
      event "U档位", "I档位": Value Change {
        n1145 = event-data() -> ("CtlRef"=w1526:refnum<vi>, "NewVal"=w1524:u32)  [unwired: 1 in, 3 out]
        n1146 = property class="Ring (严格)"(reference=w1526) -> ("Label.Text"=w1525:string)  [unwired: 1 in, 2 out]
        n1147 = case shown="\"I档位\"" w1525 {
          tunnel: w1524 -> [_ w1529 w1538]
          frame "假", Default {
          }
          frame "U档位" {
            n1148 = global write "程序全局.vi" "电压档位"(w1529) -> ()
            n1149 = case shown="4" w1529 {
              tunnel: [sgl 1000.0 ("电流限值") sgl 65.0 ("电流限值") sgl 250.0 ("电流限值") sgl 500.0 ("电流限值") sgl 750.0 ("电流限值") sgl 1000.0 ("电流限值")] -> w1527
              frame 85, Default {
              }
              frame 0 {
              }
              frame 1 {
              }
              frame 2 {
              }
              frame 3 {
              }
              frame 4 {
              }
            }
            n1150 = property on="U幅值" class="DigNum (严格)"("Maximum"=w1527, "Minimum"=0.0 ("数据输入界限:最小值")) -> ()  [unwired: 2 in, 2 out]
          }
          frame "I档位" {
            n1151 = global write "程序全局.vi" "电流档位"(w1538) -> ()
            n1152 = case shown="0" w1538 {
              tunnel: [sgl 200.0 ("电流限值") sgl 0.2 ("电流限值") sgl 1.0 ("电流限值") sgl 5.0 ("电流限值") sgl 10.0 ("电流限值") sgl 20.0 ("电流限值") sgl 30.0 ("电流限值") sgl 60.0 ("电流限值") sgl 200.0 ("电流限值")] -> w1537
              frame 85, Default {
              }
              frame 0 {
              }
              frame 1 {
              }
              frame 2 {
              }
              frame 3 {
              }
              frame 4 {
              }
              frame 5 {
              }
              frame 6 {
              }
              frame 7 {
              }
            }
            n1153 = property on="I幅值" class="DigNum (严格)"("Maximum"=w1537, "Minimum"=0.0 ("数据输入界限:最小值")) -> ()  [unwired: 2 in, 2 out]
          }
        }
      }
      event "E检定表格": Mouse Down {
        n1154 = event-data() -> ("CtlRef"=w1548:refnum<vi>)  [unwired: 1 in, 6 out]
        n1155 = property class="Tbl (严格)"(reference=w1548) -> ("EditPos"=w1553:T17)  [unwired: 1 in, 2 out]
        n1156 = property on="属性节点" class="Tbl (严格)"(reference=w1548) -> ("Active Cell"=w1551:T17)  [unwired: 1 in, 2 out]
        n1157 = Unbundle By Name(w1553) -> ("Column"=w1557:i32)
        n1158 = Unbundle By Name(w1553) -> ("Row"=w1554:i32)
        n1159 = Unbundle By Name(w1551) -> ("Row"=w1550:i32)
        n1160 = Unbundle By Name(w1553) -> ("Row"=w1549:i32)
        n1161 = Equal?(x=w1557, y=4) -> (x = y?=w1555:bool)
        n1162 = property on="E当前行" class="DigNum (严格)"("Value"=w1549) -> ()  [unwired: 2 in, 2 out]
        n1163 = case shown="真" w1555 {
          tunnel: w1554 -> [_ w1571]
          frame False {
          }
          frame True {
            n1164 = property on="E检定表格" class="Tbl (严格)"() -> ("Value"=w1570:string[][])  [unwired: 2 in, 2 out]
            n1165 = Index Array(array=w1570, index (row)=w1571) -> (element=w1576:string[])  [unwired: 1 in]
            n1166 = Index Array(array=w1576, index=5 ("索引")) -> (element=w1577:string)
            n1167 = case shown="\"否\", 默认" w1577 {
              tunnel: ["是" "否"] -> w1575
              frame "否", Default {
              }
              frame "是" {
              }
            }
            n1168 = Replace Array Subset(array=w1576, new element=w1575, index=5 ("索引")) -> (w1574:string[])
            n1169 = Replace Array Subset(array=w1570, new element=w1574, index (row)=w1571) -> (w1569:string[][])  [unwired: 1 in]
            n1170 = property on="E检定表格" class="Tbl (严格)"("Value"=w1569) -> ()  [unwired: 2 in, 2 out]
          }
        }
        n1171 = for {
          N: 6 -> [_]
          tunnel: [w1561] -> _
          tunnel: w1550 -> [w1559]
          tunnel: w1549 -> [w1558]
          i -> [w1563]
          n1172 = Bundle("Row"=w1558, w1563) -> (w1565:cluster{"Row":i32, i32})  [unwired: 1 in]
          n1173 = Bundle("Row"=w1559, w1563) -> (w1568:cluster{"Row":i32, i32})  [unwired: 1 in]
          n1174 = property on="E检定表格" class="Tbl (严格)"("Active Cell"=w1568) -> (error out=w1567:errorcluster)  [unwired: 2 in, 1 out]
          n1175 = property on="E检定表格" class="Tbl (严格)"(error in=w1567, "Cell BG Color"=u32 16777226) -> (error out=w1564:errorcluster)  [unwired: 1 in, 1 out]
          n1176 = property on="E检定表格" class="Tbl (严格)"(error in=w1564, "Active Cell"=w1565) -> (error out=w1566:errorcluster)  [unwired: 1 in, 1 out]
          n1177 = property on="E检定表格" class="Tbl (严格)"(error in=w1566, "Cell BG Color"=u32 16763457) -> (error out=w1561:errorcluster)  [unwired: 1 in, 1 out]
        }
      }
      event "E检定表格": Value Change {
        n1178 = event-data() -> ("NewVal"=w1580:string[][])  [unwired: 1 in, 4 out]
        n1179 = property on="单点检定" class="Bool (严格)"() -> ("Value"=w1582:bool)  [unwired: 2 in, 2 out]
        n1180 = call "表格行数.vi"("E检定表格"=w1580) -> ("行数"=w1581:i32)  [unwired: 2 in]
        n1181 = case shown="假" w1582 {
          tunnel: w1581 -> [w1585 _]
          tunnel: w1580 -> [w1584 _]
          frame False {
            n1182 = for {
              N: w1585 -> [_]
              tunnel: w1584 -> [w1607] mode=indexing
              tunnel: [w1592] -> w1583 mode=indexing
              w1589 = sgl 0.01
              w1602 = sgl 0.0 ("默认(0 DBL)")
              n1183 = Index Array(array=w1607, index=0 ("索引")) -> (element=w1606:string)
              n1184 = Index Array(array=w1607, index=1 ("索引")) -> (element=w1605:string)
              n1185 = Index Array(array=w1607, index=2 ("索引")) -> (element=w1604:string)
              n1186 = Index Array(array=w1607, index=3 ("索引")) -> (element=w1603:string)
              n1187 = Fract/Exp String To Number(string=w1606, default (0 dbl)=w1602) -> (number=w1601:sgl)  [unwired: 2 in, 1 out]
              n1188 = Fract/Exp String To Number(string=w1605, default (0 dbl)=w1602) -> (number=w1598:sgl)  [unwired: 2 in, 1 out]
              n1189 = Fract/Exp String To Number(string=w1604, default (0 dbl)=w1602) -> (number=w1600:sgl)  [unwired: 2 in, 1 out]
              n1190 = Fract/Exp String To Number(string=w1603, default (0 dbl)=w1602) -> (number=w1599:sgl)  [unwired: 2 in, 1 out]
              n1191 = Multiply(x=w1600, y=w1599) -> (x*y=w1588:sgl)
              n1192 = Multiply(x=w1601, y=w1598) -> (x*y=w1591:sgl)
              n1193 = Multiply(x=w1589, y=w1591) -> (x*y=w1590:sgl)
              n1194 = Multiply(x=w1589, y=w1588) -> (x*y=w1587:sgl)
              n1195 = Number To Fractional String(number=w1587, precision (6)=i16 2 ("精度(6)")) -> (F-format string=w1594:string)  [unwired: 2 in]
              n1196 = Number To Fractional String(number=w1590, precision (6)=i16 1 ("精度(6)")) -> (F-format string=w1596:string)  [unwired: 2 in]
              n1197 = Concatenate Strings(w1596, "V" ("字符串"), w1594, "A" ("字符串")) -> (w1592:string)
            }
            n1198 = property on="电能显示表" class="Tbl (严格)"("Row Headers[]"=w1583) -> ()  [unwired: 2 in, 2 out]
          }
          frame True {
          }
        }
        n1199 = property on="E行数" class="DigNum (严格)"("Value"=w1581) -> ()  [unwired: 2 in, 2 out]
      }
      event "E增删改清.插入", "E增删改清.编辑", "E增删改清.删除", "E增删改清.清空": Value Change {
        n1200 = event-data() -> ("CtlRef"=w1612:refnum<vi>, "NewVal"=w1613:bool)  [unwired: 1 in, 3 out]
        n1201 = case shown="真" w1613 {
          tunnel: w1612 -> [_ w1615]
          frame False {
          }
          frame True {
            n1202 = property class="Bool (严格)"(reference=w1615) -> ("BoolText.Text"=w1614:string)  [unwired: 1 in, 2 out]
            n1203 = case shown="\"清空\"" w1614 {
              frame "假", Default {
              }
              frame "插入" {
                w1617 = u32 16777226
                w1631 = i16 3 ("精度(6)")
                n1204 = property on="E检定参数" class="Clust (严格)"() -> ("Value"=w1638:T8)  [unwired: 2 in, 2 out]
                n1205 = Unbundle By Name(w1638) -> ("额定电压"=w1637:sgl, "U检定点"=w1636:sgl, "标定电流"=w1635:sgl, "I检定点"=w1627:sgl, "允许误差"=w1626:sgl)
                n1206 = Number To Fractional String(number=w1636, precision (6)=w1631) -> (F-format string=w1633:string)  [unwired: 2 in]
                n1207 = Number To Fractional String(number=w1635, precision (6)=w1631) -> (F-format string=w1632:string)  [unwired: 2 in]
                n1208 = Number To Fractional String(number=w1626, precision (6)=w1631) -> (F-format string=w1629:string)  [unwired: 2 in]
                n1209 = Number To Fractional String(number=w1637, precision (6)=w1631) -> (F-format string=w1634:string)  [unwired: 2 in]
                n1210 = Number To Fractional String(number=w1627, precision (6)=w1631) -> (F-format string=w1630:string)  [unwired: 2 in]
                n1211 = property on="E检定表格" class="Tbl (严格)"("Cell BG Color"=w1617) -> ()  [unwired: 2 in, 2 out]
                n1212 = property on="E当前行" class="DigNum (严格)"() -> (error out=w1624:errorcluster, "Value"=w1618:i32)  [unwired: 2 in, 1 out]
                n1213 = for {
                  N: 6 -> [_]
                  tunnel: w1618 -> [w1644]
                  tunnel: w1617 -> [w1650]
                  tunnel: [w1641] -> w1616
                  i -> [w1645]
                  n1214 = Increment(x=w1644) -> (x+1=w1643:i32)
                  n1215 = Bundle(w1643, w1645) -> (w1647:cluster{i32, i32})  [unwired: 1 in]
                  n1216 = Bundle("Value"=w1644, w1645) -> (w1651:cluster{"Value":i32, i32})  [unwired: 1 in]
                  n1217 = property on="E检定表格" class="Tbl (严格)"("Active Cell"=w1651) -> (error out=w1649:errorcluster)  [unwired: 2 in, 1 out]
                  n1218 = property on="E检定表格" class="Tbl (严格)"(error in=w1649, "Cell BG Color"=w1650) -> (error out=w1646:errorcluster)  [unwired: 1 in, 1 out]
                  n1219 = property on="E检定表格" class="Tbl (严格)"(error in=w1646, "Active Cell"=w1647) -> (error out=w1648:errorcluster)  [unwired: 1 in, 1 out]
                  n1220 = property on="E检定表格" class="Tbl (严格)"(error in=w1648, "Cell BG Color"=u32 16763457) -> (error out=w1641:errorcluster)  [unwired: 1 in, 1 out]
                }
                n1221 = Build Array(w1634, w1633, w1632, w1630, w1629, "是") -> (w1639:string[])
                n1222 = property on="E检定表格" class="Tbl (严格)"() -> ("Value"=w1640:string[][])  [unwired: 2 in, 2 out]
                n1223 = Insert Into Array(array=w1640, index (row)=w1618, new element=w1639) -> (w1628:string[][])  [unwired: 1 in]
                n1224 = Increment(x=w1618) -> (x+1=w1620:i32)
                n1225 = Bundle(w1620, "精度(6)"=i16 0) -> (w1621:cluster{i32, "精度(6)":i16})  [unwired: 1 in]
                n1226 = property on="E检定表格" class="Tbl (严格)"("Val(Sgnl)"=w1628) -> (error out=w1623:errorcluster)  [unwired: 2 in, 1 out]
                n1227 = property on="E当前行" class="DigNum (严格)"(error in=w1624, "Value"=w1620) -> ()  [unwired: 1 in, 2 out]
                n1228 = property on="E检定表格" class="Tbl (严格)"(error in=w1623, "EditPos"=w1621) -> ()  [unwired: 1 in, 2 out]
                n1229 = property on="E检定表格" class="Tbl (严格)"(error in=w1616, "Active Cell"=w1621) -> ()  [unwired: 1 in, 2 out]
              }
              frame "编辑" {
                w1658 = i16 3 ("精度(6)")
                n1230 = property on="E检定参数" class="Clust (严格)"() -> ("Value"=w1665:T8)  [unwired: 2 in, 2 out]
                n1231 = Unbundle By Name(w1665) -> ("额定电压"=w1664:sgl, "U检定点"=w1663:sgl, "标定电流"=w1662:sgl, "I检定点"=w1654:sgl, "允许误差"=w1653:sgl)
                n1232 = Number To Fractional String(number=w1663, precision (6)=w1658) -> (F-format string=w1660:string)  [unwired: 2 in]
                n1233 = Number To Fractional String(number=w1662, precision (6)=w1658) -> (F-format string=w1659:string)  [unwired: 2 in]
                n1234 = Number To Fractional String(number=w1653, precision (6)=w1658) -> (F-format string=w1656:string)  [unwired: 2 in]
                n1235 = Number To Fractional String(number=w1664, precision (6)=w1658) -> (F-format string=w1661:string)  [unwired: 2 in]
                n1236 = Number To Fractional String(number=w1654, precision (6)=w1658) -> (F-format string=w1657:string)  [unwired: 2 in]
                n1237 = property on="E当前行" class="DigNum (严格)"() -> ("Value"=w1667:i32)  [unwired: 2 in, 2 out]
                n1238 = Build Array(w1661, w1660, w1659, w1657, w1656, "是") -> (w1666:string[])
                n1239 = property on="E检定表格" class="Tbl (严格)"() -> ("Value"=w1668:string[][])  [unwired: 2 in, 2 out]
                n1240 = Replace Array Subset(array=w1668, new element=w1666, index (row)=w1667) -> (w1655:string[][])  [unwired: 1 in]
                n1241 = property on="E检定表格" class="Tbl (严格)"("Val(Sgnl)"=w1655) -> ()  [unwired: 2 in, 2 out]
              }
              frame "删除" {
                n1242 = property on="E检定表格" class="Tbl (严格)"() -> ("Value"=w1671:string[][])  [unwired: 2 in, 2 out]
                n1243 = property on="E当前行" class="DigNum (严格)"() -> ("Value"=w1669:i32)  [unwired: 2 in, 2 out]
                n1244 = Delete From Array(array=w1671, index (row)=w1669) -> (array with subset deleted=w1670:string[][])  [unwired: 2 in, 1 out]
                n1245 = property on="E检定表格" class="Tbl (严格)"("Val(Sgnl)"=w1670) -> ()  [unwired: 2 in, 2 out]
              }
              frame "清空" {
                n1246 = property on="E检定表格" class="Tbl (严格)"() -> ("Value"=w1673:string[][])  [unwired: 2 in, 2 out]
                n1247 = call "表格行数.vi"("E检定表格"=w1673) -> ("行数"=w1672:i32)  [unwired: 2 in]
                n1248 = Initialize Array("", w1672, 6 ("维数大小")) -> (w1674:string[][])
                n1249 = property on="E检定表格" class="Tbl (严格)"("Val(Sgnl)"=w1674) -> ()  [unwired: 2 in, 2 out]
              }
            }
          }
        }
      }
      event "E检定操作.开始检定": Value Change {
        n1250 = event-data() -> ("NewVal"=w1677:bool)  [unwired: 1 in, 4 out]
        n1251 = case shown="真" w1677 {
          frame False {
            w1678 = 0
            w1681 = 0
            n1252 = property on="表1" class="Bool (严格)"() -> ("Value"=w1684:bool)  [unwired: 2 in, 2 out]
            n1253 = property on="表2" class="Bool (严格)"() -> ("Value"=w1683:bool)  [unwired: 2 in, 2 out]
            n1254 = property on="表3" class="Bool (严格)"() -> ("Value"=w1682:bool)  [unwired: 2 in, 2 out]
            n1255 = property on="E检定表格" class="Tbl (严格)"("DisabledEnum"=0) -> ()  [unwired: 2 in, 2 out]
            n1256 = case shown="假" w1684 {
              frame False {
                n1257 = property on="表1OK" class="Bool (严格)"("Value"=TRUE ("表2OK")) -> ()  [unwired: 2 in, 2 out]
              }
              frame True {
                n1258 = property on="表1OK" class="Bool (严格)"("Value"=FALSE ("表2OK")) -> ()  [unwired: 2 in, 2 out]
              }
            }
            n1259 = case shown="假" w1683 {
              frame False {
                n1260 = property on="表2OK" class="Bool (严格)"("Value"=TRUE ("表2OK")) -> ()  [unwired: 2 in, 2 out]
              }
              frame True {
                n1261 = property on="表2OK" class="Bool (严格)"("Value"=FALSE ("表2OK")) -> ()  [unwired: 2 in, 2 out]
              }
            }
            n1262 = case shown="假" w1682 {
              frame False {
                n1263 = property on="表3OK" class="Bool (严格)"("Value"=TRUE ("表3OK")) -> ()  [unwired: 2 in, 2 out]
              }
              frame True {
                n1264 = property on="表3OK" class="Bool (严格)"("Value"=FALSE ("表3OK")) -> ()  [unwired: 2 in, 2 out]
              }
            }
            n1265 = property on="删除" class="Bool (严格)"("DisabledEnum"=w1678) -> ()  [unwired: 2 in, 2 out]
            n1266 = property on="编辑" class="Bool (严格)"("DisabledEnum"=w1678) -> ()  [unwired: 2 in, 2 out]
            n1267 = property on="单点检定" class="Bool (严格)"("DisabledEnum"=w1678) -> ()  [unwired: 2 in, 2 out]
            n1268 = property on="清空" class="Bool (严格)"("DisabledEnum"=w1678) -> ()  [unwired: 2 in, 2 out]
            n1269 = property on="插入" class="Bool (严格)"("DisabledEnum"=w1678) -> ()  [unwired: 2 in, 2 out]
            n1270 = property on="表1" class="Bool (严格)"("DisabledEnum"=w1681) -> ()  [unwired: 2 in, 2 out]
            n1271 = property on="表2" class="Bool (严格)"("DisabledEnum"=w1681) -> ()  [unwired: 2 in, 2 out]
            n1272 = property on="表3" class="Bool (严格)"("DisabledEnum"=w1681) -> ()  [unwired: 2 in, 2 out]
            n1273 = property on="保存方案" class="Bool (严格)"("DisabledEnum"=w1678) -> ()  [unwired: 2 in, 2 out]
            n1274 = property on="导入方案" class="Bool (严格)"("DisabledEnum"=w1678) -> ()  [unwired: 2 in, 2 out]
            n1275 = property on="检定状态" class="Bool (严格)"("Value"=FALSE ("检定状态")) -> ()  [unwired: 2 in, 2 out]
            n1276 = disable-structure shown="禁用" {
              frame Disabled {
                n1277 = property on="E行数" class="DigNum (严格)"() -> ("Value"=w1687:i32)  [unwired: 2 in, 2 out]
                n1278 = for {
                  N: w1687 -> [_]
                  i -> [w1688]
                  n1279 = for {
                    N: 7 -> [_]
                    tunnel: w1688 -> [w1693]
                    i -> [w1691]
                    n1280 = property on="电能显示表" class="Tbl (严格)"() -> ("Active Cell"=w1696:T17)  [unwired: 2 in, 2 out]
                    n1281 = Decrement(x=w1691) -> (x-1=w1690:i32)
                    n1282 = Bundle By Name(cluster=w1696, "Row"=w1693, "Column"=w1690) -> (w1695:T17)
                    n1283 = property on="电能显示表" class="Tbl (严格)"("Active Cell"=w1695) -> (error out=w1694:errorcluster)  [unwired: 2 in, 1 out]
                    n1284 = property on="电能显示表" class="Tbl (严格)"(error in=w1694, "Cell BG Color"=u32 16448250) -> ()  [unwired: 1 in, 2 out]
                  }
                }
              }
              frame Enabled {
              }
            }
            n1285 = property on="控制选项卡" class="TabCtl (严格)"("DisabledEnum"=T19."Enabled" ("禁用")) -> ()  [unwired: 2 in, 2 out]
            n1286 = property on="控制选项卡" class="TabCtl (严格)"("PageSelVis"=TRUE ("页选择器可见")) -> ()  [unwired: 2 in, 2 out]
          }
          frame True {
            w1703 = 2
            w1705 = 3
            n1287 = flat-sequence {
              frame #0 {
                n1288 = property on="串口灯" class="Bool (严格)"() -> ("Value"=w1707:bool)  [unwired: 2 in, 2 out]
                n1289 = case shown="真" w1707 {
                  frame False {
                  }
                  frame True {
                    n1290 = property on="串口号" class="VISAName"() -> ("Value"=w1708:refnum<visa-resource-name>)  [unwired: 2 in, 2 out]
                    n1291 = call "电能清零.vi"("串口号"=w1708) -> ()  [unwired: 2 in, 1 out]
                    n1292 = Wait (ms)(milliseconds to wait=50) -> ()  [unwired: 1 out]
                  }
                }
              }
              frame #1 {
                n1293 = property on="串口号" class="VISAName"() -> ("Value"=w1711:refnum<visa-resource-name>)  [unwired: 2 in, 2 out]
                n1294 = property on="电能检定通道" class="Ring (严格)"() -> ("Value"=w1712:u16)  [unwired: 2 in, 2 out]
                n1295 = call "小信号配置.vi"("电流通道"=w1712, "串口号"=w1711) -> ("应答"=w1710:string)  [unwired: 9 in]
                n1296 = case shown="\"错误\", 默认" w1710 {
                  frame "错误", Default {
                    n1297 = property on="提示信息" class="Bool (严格)"("BoolText.Text"="小信号设置出错！", "Val(Sgnl)"=TRUE ("提示信息")) -> ()  [unwired: 2 in, 2 out]
                  }
                  frame "正确" {
                  }
                }
                n1298 = property on="E行数" class="DigNum (严格)"() -> ("Value"=w1713:i32)  [unwired: 2 in, 2 out]
                n1299 = for {
                  N: w1713 -> [_]
                  i -> [w1716]
                  n1300 = for {
                    N: 7 -> [_]
                    tunnel: w1716 -> [w1721]
                    i -> [w1719]
                    n1301 = property on="电能显示表" class="Tbl (严格)"() -> ("Active Cell"=w1724:T17)  [unwired: 2 in, 2 out]
                    n1302 = Decrement(x=w1719) -> (x-1=w1718:i32)
                    n1303 = Bundle By Name(cluster=w1724, "Row"=w1721, "Column"=w1718) -> (w1723:T17)
                    n1304 = property on="电能显示表" class="Tbl (严格)"("Active Cell"=w1723) -> (error out=w1722:errorcluster)  [unwired: 2 in, 1 out]
                    n1305 = property on="电能显示表" class="Tbl (严格)"(error in=w1722, "Cell BG Color"=u32 16448250) -> ()  [unwired: 1 in, 2 out]
                  }
                }
              }
              frame #2 {
                n1306 = property on="检定状态" class="Bool (严格)"("Value"=TRUE ("检定状态")) -> ()  [unwired: 2 in, 2 out]
              }
            }
            n1307 = property on="控制选项卡" class="TabCtl (严格)"("PageSelVis"=FALSE ("页选择器可见")) -> ()  [unwired: 2 in, 2 out]
            n1308 = property on="E检定表格" class="Tbl (严格)"("DisabledEnum"=2) -> ()  [unwired: 2 in, 2 out]
            n1309 = property on="表1" class="Bool (严格)"("DisabledEnum"=w1705) -> ()  [unwired: 2 in, 2 out]
            n1310 = property on="表2" class="Bool (严格)"("DisabledEnum"=w1705) -> ()  [unwired: 2 in, 2 out]
            n1311 = property on="表3" class="Bool (严格)"("DisabledEnum"=w1705) -> ()  [unwired: 2 in, 2 out]
            n1312 = property on="插入" class="Bool (严格)"("DisabledEnum"=w1703) -> ()  [unwired: 2 in, 2 out]
            n1313 = property on="编辑" class="Bool (严格)"("DisabledEnum"=w1703) -> ()  [unwired: 2 in, 2 out]
            n1314 = property on="清空" class="Bool (严格)"("DisabledEnum"=w1703) -> ()  [unwired: 2 in, 2 out]
            n1315 = property on="单点检定" class="Bool (严格)"("DisabledEnum"=w1703) -> ()  [unwired: 2 in, 2 out]
            n1316 = property on="删除" class="Bool (严格)"("DisabledEnum"=w1703) -> ()  [unwired: 2 in, 2 out]
            n1317 = property on="保存方案" class="Bool (严格)"("DisabledEnum"=w1703) -> ()  [unwired: 2 in, 2 out]
            n1318 = property on="导入方案" class="Bool (严格)"("DisabledEnum"=w1703) -> ()  [unwired: 2 in, 2 out]
          }
        }
      }
      event "E检定操作.单点检定": Value Change {
        n1319 = event-data() -> ("NewVal"=w1726:bool)  [unwired: 1 in, 4 out]
        n1320 = case shown="真" w1726 {
          frame False {
            w1729 = TRUE ("表2OK")
            n1321 = property on="E检定表格" class="Tbl (严格)"() -> ("Value"=w1731:string[][])  [unwired: 2 in, 2 out]
            n1322 = property on="单点显示表" class="Tbl (严格)"("Visible"=FALSE ("可见")) -> ()  [unwired: 2 in, 2 out]
            n1323 = property on="电能显示表" class="Tbl (严格)"("Visible"=TRUE ("可见")) -> ()  [unwired: 2 in, 2 out]
            n1324 = property on="误差显示表" class="Tbl (严格)"("Visible"=FALSE ("可见")) -> ()  [unwired: 2 in, 2 out]
            n1325 = local write "result_Tab"(1) -> ()
            n1326 = property on="result_Tab" class="TabCtl (严格)"("Visible"=TRUE) -> ()  [unwired: 2 in, 2 out]
            n1327 = call "表格行数.vi"("E检定表格"=w1731) -> ("行数"=w1732:i32)  [unwired: 2 in]
            n1328 = for {
              N: w1732 -> [_]
              tunnel: w1731 -> [w1756] mode=indexing
              tunnel: [w1741] -> w1733 mode=indexing
              w1738 = sgl 0.01 ("x")
              w1746 = i16 1 ("精度(6)")
              w1751 = sgl 0.0 ("默认(0 DBL)")
              n1329 = Index Array(array=w1756, index=0 ("索引")) -> (element=w1755:string)
              n1330 = Index Array(array=w1756, index=1 ("索引")) -> (element=w1754:string)
              n1331 = Index Array(array=w1756, index=2 ("索引")) -> (element=w1753:string)
              n1332 = Index Array(array=w1756, index=3 ("索引")) -> (element=w1752:string)
              n1333 = Fract/Exp String To Number(string=w1755, default (0 dbl)=w1751) -> (number=w1750:sgl)  [unwired: 2 in, 1 out]
              n1334 = Fract/Exp String To Number(string=w1754, default (0 dbl)=w1751) -> (number=w1747:sgl)  [unwired: 2 in, 1 out]
              n1335 = Fract/Exp String To Number(string=w1753, default (0 dbl)=w1751) -> (number=w1749:sgl)  [unwired: 2 in, 1 out]
              n1336 = Fract/Exp String To Number(string=w1752, default (0 dbl)=w1751) -> (number=w1748:sgl)  [unwired: 2 in, 1 out]
              n1337 = Multiply(x=w1749, y=w1748) -> (x*y=w1737:sgl)
              n1338 = Multiply(x=w1750, y=w1747) -> (x*y=w1740:sgl)
              n1339 = Multiply(x=w1738, y=w1740) -> (x*y=w1739:sgl)
              n1340 = Multiply(x=w1738, y=w1737) -> (x*y=w1736:sgl)
              n1341 = Number To Fractional String(number=w1736, precision (6)=w1746) -> (F-format string=w1743:string)  [unwired: 2 in]
              n1342 = Number To Fractional String(number=w1739, precision (6)=w1746) -> (F-format string=w1745:string)  [unwired: 2 in]
              n1343 = Concatenate Strings(w1745, "V" ("字符串"), w1743, "A" ("字符串")) -> (w1741:string)
            }
            n1344 = property on="E行数" class="DigNum (严格)"("Value"=w1732) -> ()  [unwired: 2 in, 2 out]
            n1345 = property on="表1" class="Bool (严格)"("Visible"=w1729) -> ()  [unwired: 2 in, 2 out]
            n1346 = property on="表2" class="Bool (严格)"("Visible"=w1729) -> ()  [unwired: 2 in, 2 out]
            n1347 = property on="表3" class="Bool (严格)"("Visible"=w1729) -> ()  [unwired: 2 in, 2 out]
            n1348 = property on="电能显示表" class="Tbl (严格)"("Row Headers[]"=w1733) -> ()  [unwired: 2 in, 2 out]
          }
          frame True {
            w1763 = FALSE ("表2OK")
            n1349 = local write "result_Tab"(3) -> ()
            n1350 = property on="result_Tab" class="TabCtl (严格)"("Visible"=TRUE) -> ()  [unwired: 2 in, 2 out]
            n1351 = property on="表1" class="Bool (严格)"("Visible"=w1763) -> ()  [unwired: 2 in, 2 out]
            n1352 = property on="表2" class="Bool (严格)"("Visible"=w1763) -> ()  [unwired: 2 in, 2 out]
            n1353 = property on="表3" class="Bool (严格)"("Visible"=w1763) -> ()  [unwired: 2 in, 2 out]
            n1354 = property on="电能显示表" class="Tbl (严格)"("Visible"=FALSE ("可见")) -> ()  [unwired: 2 in, 2 out]
            n1355 = property on="单点显示表" class="Tbl (严格)"("Visible"=TRUE ("可见")) -> ()  [unwired: 2 in, 2 out]
            n1356 = property on="误差显示表" class="Tbl (严格)"("Visible"=FALSE ("可见")) -> ()  [unwired: 2 in, 2 out]
            n1357 = property on="单点显示表" class="Tbl (严格)"("Row Headers[]"=string[] ["脉冲输入数", "脉冲输入功率(W)", "脉冲输入电能(KWh)", "标准偏差值", "电能误差(%)"] ("行首字符串[]")) -> ()  [unwired: 2 in, 2 out]
          }
        }
      }
      event "shutDown": Value Change {
        # "停止输出,并且关机"
        n1358 = event-data() -> ("NewVal"=w1768:bool)  [unwired: 1 in, 5 out]
        n1359 = case shown="真" w1768 {
          frame False {
          }
          frame True {
            n1360 = Two Button Dialog(message="是否关机?") -> (T button?=w1769:bool)  [unwired: 2 in]
            n1361 = case shown="真" w1769 {
              frame False {
              }
              frame True {
                w1772 = u16 2 items=["电压停止", "电流停止", "全部停止"] ("启动项")
                n1362 = property on="串口号" class="VISAName"() -> ("Value"=w1773:refnum<visa-resource-name>)  [unwired: 2 in, 2 out]
                n1363 = call "输出停止.vi"("启动项"=w1772, "串口号"=w1773) -> ("应答"=w1771:string)  [unwired: 3 in]
                n1364 = case shown="\"正确\", 默认" w1771 {
                  frame "错误" {
                    n1365 = One Button Dialog(message="输出异常，请重新点击" ("消息")) -> ()  [unwired: 1 in, 1 out]
                  }
                  frame "正确", Default {
                    w1776 = FALSE
                    n1366 = disable-structure shown="启用" {
                      frame Enabled {
                        n1367 = One Button Dialog(message="停止输出后自动关闭系统，为安全起见，请及时关闭电源" ("消息")) -> ()  [unwired: 1 in, 1 out]
                      }
                      frame Disabled {
                      }
                    }
                    n1368 = property on="U状态" class="Bool (严格)"("Value"=w1776) -> ()  [unwired: 2 in, 2 out]
                    n1369 = property on="IB_status" class="Bool (严格)"("Value"=w1776) -> ()  [unwired: 2 in, 2 out]
                    n1370 = property on="UC_status" class="Bool (严格)"("Value"=w1776) -> ()  [unwired: 2 in, 2 out]
                    n1371 = property on="UB_status" class="Bool (严格)"("Value"=w1776) -> ()  [unwired: 2 in, 2 out]
                    n1372 = property on="I状态" class="Bool (严格)"("Value"=w1776) -> ()  [unwired: 2 in, 2 out]
                    n1373 = call <vilib>:"System Exec.vi"("command line"="shutdown -s") -> ()  [unwired: 7 in, 4 out]
                  }
                  frame "超时" {
                    n1374 = One Button Dialog(message="相应超时，请重新点击" ("消息")) -> ()  [unwired: 1 in, 1 out]
                  }
                }
              }
            }
          }
        }
      }
      event "E检定操作.保存方案", "E检定操作.导入方案": Value Change {
        n1375 = event-data() -> ("CtlRef"=w1779:refnum<vi>, "NewVal"=w1780:bool)  [unwired: 1 in, 3 out]
        n1376 = case shown="真" w1780 {
          tunnel: w1779 -> [_ w1782]
          frame False {
          }
          frame True {
            n1377 = property class="Bool (严格)"(reference=w1782) -> ("BoolText.Text"=w1781:string)  [unwired: 1 in, 2 out]
            n1378 = case shown="\"保存方案\"" w1781 {
              frame "假", Default {
              }
              frame "保存方案" {
                n1379 = property on="E检定表格" class="Tbl (严格)"() -> ("Value"=w1783:string[][])  [unwired: 2 in, 2 out]
                n1380 = call-poly <vilib>:"Write To Spreadsheet File.vi"("2D data"=w1783) -> ()  [unwired: 7 in, 1 out]
              }
              frame "导入方案" {
                n1381 = call-poly <vilib>:"Read From Spreadsheet File.vi"() -> ("all rows"=w1786:string[][], "new file path (Not A Path if cancelled)"=w1784:path)  [unwired: 7 in, 3 out]
                n1382 = Strip Path(path=w1784) -> (name=w1785:string)  [unwired: 1 out]
                n1383 = property on="E检定表格" class="Tbl (严格)"("Caption.Text"=w1785) -> ()  [unwired: 2 in, 2 out]
                n1384 = property on="E检定表格" class="Tbl (严格)"("Val(Sgnl)"=w1786) -> ()  [unwired: 2 in, 2 out]
              }
            }
          }
        }
      }
      event "表1", "表2", "表3": Value Change {
        n1385 = event-data() -> ()  [unwired: 1 in, 5 out]
        n1386 = flat-sequence {
          frame #0 {
            n1387 = property on="表1" class="Bool (严格)"() -> ("Value"=w1790:bool)  [unwired: 2 in, 2 out]
            n1388 = property on="表2" class="Bool (严格)"() -> ("Value"=w1789:bool)  [unwired: 2 in, 2 out]
            n1389 = property on="表3" class="Bool (严格)"() -> ("Value"=w1788:bool)  [unwired: 2 in, 2 out]
            n1390 = Compound Arithmetic op=OR(w1790, w1789, w1788) -> (w1787:bool)
            n1391 = case shown="假" w1787 {
              frame False {
                n1392 = property on="表1" class="Bool (严格)"("Value"=TRUE ("表1")) -> ()  [unwired: 2 in, 2 out]
              }
              frame True {
              }
            }
          }
          frame #1 {
            n1393 = property on="表1" class="Bool (严格)"() -> ("Value"=w1792:bool)  [unwired: 2 in, 2 out]
            n1394 = property on="表2" class="Bool (严格)"() -> ("Value"=w1793:bool)  [unwired: 2 in, 2 out]
            n1395 = property on="表3" class="Bool (严格)"() -> ("Value"=w1794:bool)  [unwired: 2 in, 2 out]
            n1396 = Not(x=w1792) -> (.not. x?=w1795:bool)
            n1397 = Not(x=w1794) -> (.not. x?=w1797:bool)
            n1398 = Not(x=w1793) -> (.not. x?=w1796:bool)
            n1399 = property on="表1OK" class="Bool (严格)"("Value"=w1795) -> ()  [unwired: 2 in, 2 out]
            n1400 = property on="表2OK" class="Bool (严格)"("Value"=w1796) -> ()  [unwired: 2 in, 2 out]
            n1401 = property on="表3OK" class="Bool (严格)"("Value"=w1797) -> ()  [unwired: 2 in, 2 out]
          }
        }
      }
      event "UI检定参数.检定项目": Value Change {
        n1402 = event-data() -> ("NewVal"=w1798:u16)  [unwired: 1 in, 4 out]
        n1403 = case shown="1" w1798 {
          frame 0, Default {
            n1404 = property on="UI增删改清" class="Clust (严格)"("DisabledEnum"=0) -> ()  [unwired: 2 in, 2 out]
            n1405 = property on="保存方案" class="Bool (严格)"("DisabledEnum"=0) -> ()  [unwired: 2 in, 2 out]
            n1406 = property on="导入方案" class="Bool (严格)"("DisabledEnum"=0) -> ()  [unwired: 2 in, 2 out]
            n1407 = property on="UI检定表格" class="Tbl (严格)"("Column Headers[]"=string[] ["电压幅值(V)", "检定点(%)", "误差限值(%)"] ("列首字符串[]")) -> ()  [unwired: 2 in, 2 out]
            n1408 = property on="UI检定表格" class="Tbl (严格)"("DisabledEnum"=0) -> ()  [unwired: 2 in, 2 out]
            n1409 = property on="计算误差" class="Bool (严格)"("DisabledEnum"=0) -> ()  [unwired: 2 in, 2 out]
            n1410 = property on="电压检定点" class="DigNum (严格)"("DisabledEnum"=0) -> ()  [unwired: 2 in, 2 out]
            n1411 = property on="额定电压" class="DigNum (严格)"("DisabledEnum"=0) -> ()  [unwired: 2 in, 2 out]
            n1412 = property on="电流检定点" class="DigNum (严格)"("DisabledEnum"=3) -> ()  [unwired: 2 in, 2 out]
            n1413 = property on="误差限值" class="DigNum (严格)"("DisabledEnum"=0) -> ()  [unwired: 2 in, 2 out]
            n1414 = property on="标定电流" class="DigNum (严格)"("DisabledEnum"=3) -> ()  [unwired: 2 in, 2 out]
            n1415 = property on="电压纹波" class="DigNum (严格)"("DisabledEnum"=3) -> ()  [unwired: 2 in, 2 out]
            n1416 = property on="电流纹波" class="DigNum (严格)"("DisabledEnum"=3) -> ()  [unwired: 2 in, 2 out]
            n1417 = property on="纹波频率" class="DigNum (严格)"("DisabledEnum"=3) -> ()  [unwired: 2 in, 2 out]
            n1418 = Current VI's Path() -> (path=w1802:path)
            n1419 = Strip Path(path=w1802) -> (stripped path=w1801:path)  [unwired: 1 out]
            n1420 = Initialize Array("", 15 ("维数大小"), 3 ("维数大小")) -> (w1809:string[][])
            n1421 = Strip Path(path=w1801) -> (stripped path=w1800:path)  [unwired: 1 out]
            n1422 = property on="UI检定表格" class="Tbl (严格)"("Val(Sgnl)"=w1809) -> ()  [unwired: 2 in, 2 out]
            n1423 = Build Path(base path=w1800, name or relative path="table\\默认电压误差表" ("名称或相对路径")) -> (appended path=w1799:path)
            n1424 = property on="误差显示表" class="Tbl (严格)"("Column Headers[]"=string[] ["表1电压(V)", "误差(%)", "表2电压(V)", "误差(%)", "表3电压(V)", "误差(%)"] ("列首字符串[]")) -> ()  [unwired: 2 in, 2 out]
            n1425 = call-poly <vilib>:"Read From Spreadsheet File.vi"("file path (dialog if empty)"=w1799) -> ("all rows"=w1804:string[][])  [unwired: 6 in, 4 out]
            n1426 = property on="UI检定表格" class="Tbl (严格)"("Val(Sgnl)"=w1804) -> ()  [unwired: 2 in, 2 out]
          }
          frame 1 {
            n1427 = property on="UI检定表格" class="Tbl (严格)"("DisabledEnum"=0) -> ()  [unwired: 2 in, 2 out]
            n1428 = property on="UI增删改清" class="Clust (严格)"("DisabledEnum"=0) -> ()  [unwired: 2 in, 2 out]
            n1429 = property on="计算误差" class="Bool (严格)"("DisabledEnum"=0) -> ()  [unwired: 2 in, 2 out]
            n1430 = property on="保存方案" class="Bool (严格)"("DisabledEnum"=0) -> ()  [unwired: 2 in, 2 out]
            n1431 = property on="导入方案" class="Bool (严格)"("DisabledEnum"=0) -> ()  [unwired: 2 in, 2 out]
            n1432 = property on="额定电压" class="DigNum (严格)"("DisabledEnum"=3) -> ()  [unwired: 2 in, 2 out]
            n1433 = property on="标定电流" class="DigNum (严格)"("DisabledEnum"=0) -> ()  [unwired: 2 in, 2 out]
            n1434 = property on="误差限值" class="DigNum (严格)"("DisabledEnum"=0) -> ()  [unwired: 2 in, 2 out]
            n1435 = property on="电压纹波" class="DigNum (严格)"("DisabledEnum"=3) -> ()  [unwired: 2 in, 2 out]
            n1436 = property on="电流纹波" class="DigNum (严格)"("DisabledEnum"=3) -> ()  [unwired: 2 in, 2 out]
            n1437 = property on="纹波频率" class="DigNum (严格)"("DisabledEnum"=3) -> ()  [unwired: 2 in, 2 out]
            n1438 = property on="电压检定点" class="DigNum (严格)"("DisabledEnum"=3) -> ()  [unwired: 2 in, 2 out]
            n1439 = property on="电流检定点" class="DigNum (严格)"("DisabledEnum"=0) -> ()  [unwired: 2 in, 2 out]
            n1440 = Current VI's Path() -> (path=w1827:path)
            n1441 = Strip Path(path=w1827) -> (stripped path=w1826:path)  [unwired: 1 out]
            n1442 = Strip Path(path=w1826) -> (stripped path=w1825:path)  [unwired: 1 out]
            n1443 = Build Path(base path=w1825, name or relative path="table\\默认电流误差表" ("名称或相对路径")) -> (appended path=w1824:path)
            n1444 = Initialize Array("", 15 ("维数大小"), 3 ("维数大小")) -> (w1834:string[][])
            n1445 = call-poly <vilib>:"Read From Spreadsheet File.vi"("file path (dialog if empty)"=w1824) -> ("all rows"=w1829:string[][])  [unwired: 6 in, 4 out]
            n1446 = property on="误差显示表" class="Tbl (严格)"("Column Headers[]"=string[] ["表1电流(A)", "误差(%)", "表2电流(A)", "误差(%)", "表3电流(A)", "误差(%)"] ("列首字符串[]")) -> ()  [unwired: 2 in, 2 out]
            n1447 = property on="UI检定表格" class="Tbl (严格)"("Val(Sgnl)"=w1829) -> ()  [unwired: 2 in, 2 out]
            n1448 = property on="UI检定表格" class="Tbl (严格)"("Column Headers[]"=string[] ["电流幅值(A)", "检定点(%)", "误差限值(%)"] ("列首字符串[]")) -> ()  [unwired: 2 in, 2 out]
            n1449 = property on="UI检定表格" class="Tbl (严格)"("Val(Sgnl)"=w1834) -> ()  [unwired: 2 in, 2 out]
          }
          frame 2 {
            n1450 = property on="UI检定表格" class="Tbl (严格)"("Column Headers[]"=string[] ["", ""] ("列首字符串[]")) -> ()  [unwired: 2 in, 2 out]
            n1451 = property on="UI检定表格" class="Tbl (严格)"("DisabledEnum"=3) -> ()  [unwired: 2 in, 2 out]
            n1452 = property on="UI增删改清" class="Clust (严格)"("DisabledEnum"=3) -> ()  [unwired: 2 in, 2 out]
            n1453 = property on="保存方案" class="Bool (严格)"("DisabledEnum"=3) -> ()  [unwired: 2 in, 2 out]
            n1454 = property on="导入方案" class="Bool (严格)"("DisabledEnum"=3) -> ()  [unwired: 2 in, 2 out]
            n1455 = property on="计算误差" class="Bool (严格)"("DisabledEnum"=3) -> ()  [unwired: 2 in, 2 out]
            n1456 = property on="额定电压" class="DigNum (严格)"("DisabledEnum"=0) -> ()  [unwired: 2 in, 2 out]
            n1457 = property on="标定电流" class="DigNum (严格)"("DisabledEnum"=0) -> ()  [unwired: 2 in, 2 out]
            n1458 = property on="误差限值" class="DigNum (严格)"("DisabledEnum"=3) -> ()  [unwired: 2 in, 2 out]
            n1459 = property on="电压纹波" class="DigNum (严格)"("DisabledEnum"=0) -> ()  [unwired: 2 in, 2 out]
            n1460 = property on="电流纹波" class="DigNum (严格)"("DisabledEnum"=0) -> ()  [unwired: 2 in, 2 out]
            n1461 = property on="纹波频率" class="DigNum (严格)"("DisabledEnum"=0) -> ()  [unwired: 2 in, 2 out]
            n1462 = property on="电压检定点" class="DigNum (严格)"("DisabledEnum"=0) -> ()  [unwired: 2 in, 2 out]
            n1463 = property on="电流检定点" class="DigNum (严格)"("DisabledEnum"=0) -> ()  [unwired: 2 in, 2 out]
            n1464 = Initialize Array("", 15 ("维数大小"), 3 ("维数大小")) -> (w1853:string[][])
            n1465 = property on="UI检定表格" class="Tbl (严格)"("Val(Sgnl)"=w1853) -> ()  [unwired: 2 in, 2 out]
          }
        }
      }
      event "UI检定表格": Mouse Down {
        n1466 = event-data() -> ("CtlRef"=w1867:refnum<vi>)  [unwired: 1 in, 6 out]
        n1467 = property class="Tbl (严格)"(reference=w1867) -> ("EditPos"=w1872:T17)  [unwired: 1 in, 2 out]
        n1468 = property on="属性节点" class="Tbl (严格)"(reference=w1867, "Cell BG Color"=u32 16777226) -> (reference out=w1869:refnum<vi>, error out=w1873:errorcluster)  [unwired: 1 in]
        n1469 = property on="属性节点" class="Tbl (严格)"(reference=w1869, error in=w1873, "Active Cell"=w1872) -> (reference out=w1868:refnum<vi>, error out=w1874:errorcluster)
        n1470 = Unbundle By Name(w1872) -> ("Row"=w1875:i32)
        n1471 = property on="UI当前行" class="DigNum (严格)"("Value"=w1875) -> ()  [unwired: 2 in, 2 out]
        n1472 = property on="属性节点" class="Tbl (严格)"(reference=w1868, error in=w1874, "Cell BG Color"=u32 16763457) -> ()  [unwired: 2 out]
      }
      event "UI检定表格": Value Change {
        n1473 = event-data() -> ("NewVal"=w1877:string[][])  [unwired: 1 in, 4 out]
        n1474 = call "表格行数.vi"("E检定表格"=w1877) -> ("行数"=w1876:i32)  [unwired: 2 in]
        n1475 = for {
          N: w1876 -> [_]
          tunnel: w1877 -> [w1889] mode=indexing
          tunnel: [w1885] -> w1878 mode=indexing
          w1884 = 0.0
          n1476 = Index Array(array=w1889, index=0 ("索引")) -> (element=w1888:string)
          n1477 = Index Array(array=w1889, index=1 ("索引")) -> (element=w1887:string)
          n1478 = Fract/Exp String To Number(string=w1888, default (0 dbl)=w1884) -> (number=w1883:dbl)  [unwired: 2 in, 1 out]
          n1479 = Fract/Exp String To Number(string=w1887, default (0 dbl)=w1884) -> (number=w1881:dbl)  [unwired: 2 in, 1 out]
          n1480 = Multiply(x=w1881, y=0.01) -> (x*y=w1879:dbl)
          n1481 = Multiply(x=w1883, y=w1879) -> (x*y=w1882:dbl)
          n1482 = Number To Fractional String(number=w1882, precision (6)=i16 2 ("精度(6)")) -> (F-format string=w1885:string)  [unwired: 2 in]
        }
        n1483 = property on="UI行数" class="DigNum (严格)"("Value"=w1876) -> ()  [unwired: 2 in, 2 out]
        n1484 = property on="误差显示表" class="Tbl (严格)"("Row Headers[]"=w1878) -> ()  [unwired: 2 in, 2 out]
      }
      event "UI增删改清.插入", "UI增删改清.编辑", "UI增删改清.删除", "UI增删改清.清空": Value Change {
        n1485 = event-data() -> ("CtlRef"=w1894:refnum<vi>, "NewVal"=w1896:bool)  [unwired: 1 in, 3 out]
        n1486 = property class="Bool (严格)"(reference=w1894) -> ("BoolText.Text"=w1893:string)  [unwired: 1 in, 2 out]
        n1487 = property on="UI检定参数" class="Clust (严格)"() -> ("Value"=w1892:T11)  [unwired: 2 in, 2 out]
        n1488 = property on="检定项目" class="Ring (严格)"() -> ("Value"=w1895:u16)  [unwired: 2 in, 2 out]
        n1489 = case shown="真" w1896 {
          tunnel: w1895 -> [_ w1899]
          tunnel: w1893 -> [_ w1898]
          tunnel: w1892 -> [_ w1897]
          frame False {
          }
          frame True {
            n1490 = case shown="1" w1899 {
              tunnel: w1898 -> [w1901 w1936]
              tunnel: w1897 -> [w1900 w1935]
              frame 0, Default {
                n1491 = case shown="\"清空\"" w1901 {
                  tunnel: w1900 -> [_ w1909 w1920 _ _]
                  frame "假", Default {
                  }
                  frame "插入" {
                    w1907 = i16 3 ("精度(6)")
                    n1492 = Unbundle By Name(w1909) -> ("额定电压"=w1908:sgl, "电压检定点"=w1906:sgl, "误差限值"=w1905:sgl)  [unwired: 2 out]
                    n1493 = Number To Fractional String(number=w1906, precision (6)=w1907) -> (F-format string=w1911:string)  [unwired: 2 in]
                    n1494 = Number To Fractional String(number=w1908, precision (6)=w1907) -> (F-format string=w1912:string)  [unwired: 2 in]
                    n1495 = Number To Fractional String(number=w1905, precision (6)=w1907) -> (F-format string=w1904:string)  [unwired: 2 in]
                    n1496 = property on="UI当前行" class="DigNum (严格)"() -> ("Value"=w1903:i32)  [unwired: 2 in, 2 out]
                    n1497 = property on="UI检定表格" class="Tbl (严格)"() -> ("Value"=w1914:string[][])  [unwired: 2 in, 2 out]
                    n1498 = Build Array(w1912, w1911, w1904) -> (w1913:string[])
                    n1499 = Increment(x=w1903) -> (x+1=w1902:i32)
                    n1500 = Insert Into Array(array=w1914, index (row)=w1902, new element=w1913) -> (w1910:string[][])  [unwired: 1 in]
                    n1501 = property on="UI检定表格" class="Tbl (严格)"("Val(Sgnl)"=w1910) -> ()  [unwired: 2 in, 2 out]
                  }
                  frame "编辑" {
                    w1917 = i16 3 ("精度(6)")
                    n1502 = Unbundle By Name(w1920) -> ("额定电压"=w1919:sgl, "电压检定点"=w1918:sgl, "误差限值"=w1916:sgl)  [unwired: 2 out]
                    n1503 = Number To Fractional String(number=w1918, precision (6)=w1917) -> (F-format string=w1925:string)  [unwired: 2 in]
                    n1504 = Number To Fractional String(number=w1916, precision (6)=w1917) -> (F-format string=w1915:string)  [unwired: 2 in]
                    n1505 = Number To Fractional String(number=w1919, precision (6)=w1917) -> (F-format string=w1926:string)  [unwired: 2 in]
                    n1506 = property on="UI当前行" class="DigNum (严格)"() -> ("Value"=w1923:i32)  [unwired: 2 in, 2 out]
                    n1507 = Build Array(w1926, w1925, w1915) -> (w1922:string[])
                    n1508 = property on="UI检定表格" class="Tbl (严格)"() -> ("Value"=w1924:string[][])  [unwired: 2 in, 2 out]
                    n1509 = Replace Array Subset(array=w1924, new element=w1922, index (row)=w1923) -> (w1921:string[][])  [unwired: 1 in]
                    n1510 = property on="UI检定表格" class="Tbl (严格)"("Val(Sgnl)"=w1921) -> ()  [unwired: 2 in, 2 out]
                  }
                  frame "删除" {
                    n1511 = property on="UI当前行" class="DigNum (严格)"() -> ("Value"=w1927:i32)  [unwired: 2 in, 2 out]
                    n1512 = property on="UI检定表格" class="Tbl (严格)"() -> ("Value"=w1928:string[][])  [unwired: 2 in, 2 out]
                    n1513 = Delete From Array(array=w1928, index (row)=w1927) -> (array with subset deleted=w1929:string[][])  [unwired: 2 in, 1 out]
                    n1514 = property on="UI检定表格" class="Tbl (严格)"("Val(Sgnl)"=w1929) -> ()  [unwired: 2 in, 2 out]
                  }
                  frame "清空" {
                    n1515 = property on="UI检定表格" class="Tbl (严格)"() -> ("Value"=w1931:string[][])  [unwired: 2 in, 2 out]
                    n1516 = call "表格行数.vi"("E检定表格"=w1931) -> ("行数"=w1930:i32)  [unwired: 2 in]
                    n1517 = Initialize Array("", w1930, 2 ("维数大小")) -> (w1932:string[][])
                    n1518 = property on="UI检定表格" class="Tbl (严格)"("Val(Sgnl)"=w1932) -> ()  [unwired: 2 in, 2 out]
                  }
                }
              }
              frame 1 {
                n1519 = case shown="\"清空\"" w1936 {
                  tunnel: w1935 -> [_ w1942 w1954 _ _]
                  frame "假", Default {
                  }
                  frame "插入" {
                    w1939 = i16 3 ("精度(6)")
                    n1520 = Unbundle By Name(w1942) -> ("标定电流"=w1941:sgl, "电流检定点"=w1940:sgl, "误差限值"=w1938:sgl)  [unwired: 2 out]
                    n1521 = Number To Fractional String(number=w1938, precision (6)=w1939) -> (F-format string=w1937:string)  [unwired: 2 in]
                    n1522 = Number To Fractional String(number=w1940, precision (6)=w1939) -> (F-format string=w1944:string)  [unwired: 2 in]
                    n1523 = Number To Fractional String(number=w1941, precision (6)=w1939) -> (F-format string=w1945:string)  [unwired: 2 in]
                    n1524 = property on="UI当前行" class="DigNum (严格)"() -> ("Value"=w1947:i32)  [unwired: 2 in, 2 out]
                    n1525 = Build Array(w1945, w1944, w1937) -> (w1946:string[])
                    n1526 = property on="UI检定表格" class="Tbl (严格)"() -> ("Value"=w1948:string[][])  [unwired: 2 in, 2 out]
                    n1527 = Insert Into Array(array=w1948, index (row)=w1947, new element=w1946) -> (w1943:string[][])  [unwired: 1 in]
                    n1528 = property on="UI检定表格" class="Tbl (严格)"("Val(Sgnl)"=w1943) -> ()  [unwired: 2 in, 2 out]
                  }
                  frame "编辑" {
                    w1950 = i16 3 ("精度(6)")
                    n1529 = Unbundle By Name(w1954) -> ("标定电流"=w1952:sgl, "电流检定点"=w1953:sgl, "误差限值"=w1951:sgl)  [unwired: 2 out]
                    n1530 = Number To Fractional String(number=w1951, precision (6)=w1950) -> (F-format string=w1949:string)  [unwired: 2 in]
                    n1531 = Number To Fractional String(number=w1953, precision (6)=w1950) -> (F-format string=w1959:string)  [unwired: 2 in]
                    n1532 = Number To Fractional String(number=w1952, precision (6)=w1950) -> (F-format string=w1960:string)  [unwired: 2 in]
                    n1533 = property on="UI当前行" class="DigNum (严格)"() -> ("Value"=w1957:i32)  [unwired: 2 in, 2 out]
                    n1534 = Build Array(w1960, w1959, w1949) -> (w1956:string[])
                    n1535 = property on="UI检定表格" class="Tbl (严格)"() -> ("Value"=w1958:string[][])  [unwired: 2 in, 2 out]
                    n1536 = Replace Array Subset(array=w1958, new element=w1956, index (row)=w1957) -> (w1955:string[][])  [unwired: 1 in]
                    n1537 = property on="UI检定表格" class="Tbl (严格)"("Val(Sgnl)"=w1955) -> ()  [unwired: 2 in, 2 out]
                  }
                  frame "删除" {
                    n1538 = property on="UI当前行" class="DigNum (严格)"() -> ("Value"=w1961:i32)  [unwired: 2 in, 2 out]
                    n1539 = property on="UI检定表格" class="Tbl (严格)"() -> ("Value"=w1962:string[][])  [unwired: 2 in, 2 out]
                    n1540 = Delete From Array(array=w1962, index (row)=w1961) -> (array with subset deleted=w1963:string[][])  [unwired: 2 in, 1 out]
                    n1541 = property on="UI检定表格" class="Tbl (严格)"("Val(Sgnl)"=w1963) -> ()  [unwired: 2 in, 2 out]
                  }
                  frame "清空" {
                    n1542 = property on="UI检定表格" class="Tbl (严格)"() -> ("Value"=w1965:string[][])  [unwired: 2 in, 2 out]
                    n1543 = call "表格行数.vi"("E检定表格"=w1965) -> ("行数"=w1964:i32)  [unwired: 2 in]
                    n1544 = Initialize Array("", w1964, 2 ("维数大小")) -> (w1966:string[][])
                    n1545 = property on="UI检定表格" class="Tbl (严格)"("Val(Sgnl)"=w1966) -> ()  [unwired: 2 in, 2 out]
                  }
                }
              }
            }
          }
        }
      }
      event "UI检定操作.输出开关": Value Change {
        n1546 = event-data() -> ("NewVal"=w1969:bool)  [unwired: 1 in, 4 out]
        n1547 = property on="检定项目" class="Ring (严格)"() -> ("Value"=w1970:u16)  [unwired: 2 in, 2 out]
        n1548 = case shown="真" w1969 {
          tunnel: w1970 -> [_ w2005]
          frame False {
            w1973 = u16 2 items=["电压停止", "电流停止", "全部停止"] ("启动项")
            n1549 = property on="串口号" class="VISAName"() -> ("Value"=w1972:refnum<visa-resource-name>)  [unwired: 2 in, 2 out]
            n1550 = call "输出停止.vi"("启动项"=w1973, "串口号"=w1972) -> ("应答"=w1971:string)  [unwired: 3 in]
            n1551 = case shown="\"正确\"" w1971 {
              frame "错误", Default {
                n1552 = property on="提示信息" class="Bool (严格)"("BoolText.Text"="停止失败！", "Val(Sgnl)"=TRUE ("提示信息")) -> ()  [unwired: 2 in, 2 out]
              }
              frame "超时" {
                n1553 = property on="提示信息" class="Bool (严格)"("BoolText.Text"="停止超时！", "Val(Sgnl)"=TRUE ("提示信息")) -> ()  [unwired: 2 in, 2 out]
              }
              frame "正确" {
                w1981 = 0.0 ("数字")
                n1554 = property on="本机表格" class="Tbl (严格)"() -> ("Value"=w1992:string[][])  [unwired: 2 in, 2 out]
                n1555 = Index Array(array=w1992, index (col)=0 ("禁用的索引 (列)")) -> (element=w1994:string[])  [unwired: 1 in]
                n1556 = Number To Fractional String(number=w1981, precision (6)=i16 3 ("精度(6)")) -> (F-format string=w1999:string)  [unwired: 2 in]
                n1557 = Number To Fractional String(number=w1981, precision (6)=i16 3 ("精度(6)")) -> (F-format string=w2000:string)  [unwired: 2 in]
                n1558 = Number To Fractional String(number=w1981, precision (6)=i16 3 ("精度(6)")) -> (F-format string=w1991:string)  [unwired: 2 in]
                n1559 = Number To Fractional String(number=w1981, precision (6)=i16 3 ("精度(6)")) -> (F-format string=w1988:string)  [unwired: 2 in]
                n1560 = Number To Fractional String(number=w1981, precision (6)=i16 3 ("精度(6)")) -> (F-format string=w1987:string)  [unwired: 2 in]
                n1561 = Replace Array Subset(array=w1994, new element=w1999, index=0 ("索引")) -> (w1997:string[])
                n1562 = Replace Array Subset(array=w1997, new element=w2000, index=1 ("索引")) -> (w1985:string[])
                n1563 = Replace Array Subset(array=w1985, new element=w1991, index=2 ("索引")) -> (w1984:string[])
                n1564 = Replace Array Subset(array=w1984, new element=w1988, index=3 ("索引")) -> (w1983:string[])
                n1565 = Replace Array Subset(array=w1983, new element=w1987, index=4 ("索引")) -> (w1982:string[])
                n1566 = Replace Array Subset(array=w1992, new element=w1982, index (col)=0 ("禁用的索引 (列)")) -> (w2002:string[][])  [unwired: 1 in]
                n1567 = property on="本机表格" class="Tbl (严格)"("Value"=w2002) -> ()  [unwired: 2 in, 2 out]
              }
            }
          }
          frame True {
            n1568 = property on="串口号" class="VISAName"() -> ("Value"=w2004:refnum<visa-resource-name>)  [unwired: 2 in, 2 out]
            n1569 = case shown="2" w2005 {
              tunnel: w2004 -> [w2007 w2055 w2135]
              frame 0, Default {
                w2023 = u32 85 ("电流档位")
                w2009 = sgl 0.0 ("电压纹波")
                n1570 = property on="UI检定表格" class="Tbl (严格)"() -> ("Value"=w2022:string[][])  [unwired: 2 in, 2 out]
                n1571 = property on="UI当前行" class="DigNum (严格)"() -> ("Value"=w2021:i32)  [unwired: 2 in, 2 out]
                n1572 = Index Array(array=w2022, index (row)=w2021) -> (element=w2014:string[])  [unwired: 1 in]
                n1573 = Index Array(array=w2014, index=0 ("索引")) -> (element=w2020:string)
                n1574 = Index Array(array=w2014, index=1 ("索引")) -> (element=w2015:string)
                n1575 = Fract/Exp String To Number(string=w2020, default (0 dbl)=sgl 0.0 ("默认(0 DBL)")) -> (number=w2011:sgl)  [unwired: 2 in, 1 out]
                n1576 = Fract/Exp String To Number(string=w2015, default (0 dbl)=sgl 0.0 ("默认(0 DBL)")) -> (number=w2013:sgl)  [unwired: 2 in, 1 out]
                n1577 = Multiply(x=w2013, y=sgl 0.01) -> (x*y=w2010:sgl)
                n1578 = Multiply(x=w2011, y=w2010) -> (x*y=w2006:sgl)
                n1579 = call "高精度写.vi"("电压幅值"=w2006, "电压纹波"=w2009, "串口号"=w2007, "电压档位"=w2023, "电流幅值"=w2009, "电流档位值"=w2023, "纹波频率"=w2009, "电流纹波"=w2009) -> ("应答"=w2008:string)  [unwired: 7 in]
                n1580 = case shown="\"正确\"" w2008 {
                  tunnel: w2007 -> [_ _ w2030]
                  tunnel: w2006 -> [_ _ w2028]
                  frame "错误", Default {
                    n1581 = property on="提示信息" class="Bool (严格)"("BoolText.Text"="高精度写错误！", "Val(Sgnl)"=TRUE ("提示信息")) -> ()  [unwired: 2 in, 2 out]
                  }
                  frame "超时" {
                    n1582 = property on="提示信息" class="Bool (严格)"("BoolText.Text"="高精度写超时！", "Val(Sgnl)"=TRUE ("提示信息")) -> ()  [unwired: 2 in, 2 out]
                  }
                  frame "正确" {
                    w2031 = u16 0 items=["电压启动", "电流启动", "全部启动"] ("启动项")
                    n1583 = call "输出启动.vi"("启动项"=w2031, "串口号"=w2030) -> ("应答"=w2029:string)  [unwired: 3 in]
                    n1584 = case shown="\"正确\"" w2029 {
                      tunnel: w2028 -> [_ _ w2036]
                      frame "错误", Default {
                        n1585 = property on="提示信息" class="Bool (严格)"("BoolText.Text"="输出失败！", "Val(Sgnl)"=TRUE ("提示信息")) -> ()  [unwired: 2 in, 2 out]
                      }
                      frame "超时" {
                        n1586 = property on="提示信息" class="Bool (严格)"("BoolText.Text"="输出超时！", "Val(Sgnl)"=TRUE ("提示信息")) -> ()  [unwired: 2 in, 2 out]
                      }
                      frame "正确" {
                        n1587 = property on="本机表格" class="Tbl (严格)"() -> ("Value"=w2038:string[][])  [unwired: 2 in, 2 out]
                        n1588 = Index Array(array=w2038, index (col)=0 ("禁用的索引 (列)")) -> (element=w2040:string[])  [unwired: 1 in]
                        n1589 = Number To Fractional String(number=w2036, precision (6)=i16 3 ("精度(6)")) -> (F-format string=w2045:string)  [unwired: 2 in]
                        n1590 = Number To Fractional String(number=0.0 ("数字"), precision (6)=i16 3 ("精度(6)")) -> (F-format string=w2046:string)  [unwired: 2 in]
                        n1591 = Replace Array Subset(array=w2040, new element=w2045, index=0 ("索引")) -> (w2043:string[])
                        n1592 = Replace Array Subset(array=w2043, new element=w2046, index=1 ("索引")) -> (w2049:string[])
                        n1593 = Replace Array Subset(array=w2038, new element=w2049, index (col)=0 ("禁用的索引 (列)")) -> (w2048:string[][])  [unwired: 1 in]
                        n1594 = property on="本机表格" class="Tbl (严格)"("Value"=w2048) -> ()  [unwired: 2 in, 2 out]
                      }
                    }
                  }
                }
              }
              frame 1 {
                w2070 = u32 85 ("电流档位")
                w2056 = sgl 0.0 ("电压纹波")
                n1595 = property on="误差电流通道" class="Ring (严格)"() -> ("Value"=w2051:u16)  [unwired: 2 in, 2 out]
                n1596 = property on="UI检定表格" class="Tbl (严格)"() -> ("Value"=w2069:string[][])  [unwired: 2 in, 2 out]
                n1597 = property on="UI当前行" class="DigNum (严格)"() -> ("Value"=w2068:i32)  [unwired: 2 in, 2 out]
                n1598 = Index Array(array=w2069, index (row)=w2068) -> (element=w2061:string[])  [unwired: 1 in]
                n1599 = Index Array(array=w2061, index=0 ("索引")) -> (element=w2067:string)
                n1600 = Index Array(array=w2061, index=1 ("索引")) -> (element=w2062:string)
                n1601 = Fract/Exp String To Number(string=w2067, default (0 dbl)=sgl 0.0 ("默认(0 DBL)")) -> (number=w2057:sgl)  [unwired: 2 in, 1 out]
                n1602 = Fract/Exp String To Number(string=w2062, default (0 dbl)=sgl 0.0 ("默认(0 DBL)")) -> (number=w2059:sgl)  [unwired: 2 in, 1 out]
                n1603 = Multiply(x=w2059, y=sgl 0.01) -> (x*y=w2058:sgl)
                n1604 = Multiply(x=w2057, y=w2058) -> (x*y=w2052:sgl)
                n1605 = case shown="1" w2051 {
                  tunnel: w2052 -> [w2071 w2074 w2080 w2086]
                  tunnel: [w2071 w2073 w2079 w2085] -> w2053
                  frame 0, Default {
                  }
                  frame 1 {
                    n1606 = property on="小信号变比(A/1mv)" class="Clust (严格)"() -> ("Value"=w2077:cluster{"电流2":sgl, "电流3":sgl, "电流4":sgl})  [unwired: 2 in, 2 out]
                    n1607 = Unbundle(w2077) -> ("电流2"=w2075:sgl)  [unwired: 2 out]
                    n1608 = Multiply(x=w2075, y=1000.0) -> (x*y=w2072:dbl)
                    n1609 = Divide(x=w2074, y=w2072) -> (x/y=w2073:dbl)
                  }
                  frame 2 {
                    n1610 = property on="小信号变比(A/1mv)" class="Clust (严格)"() -> ("Value"=w2083:cluster{"电流2":sgl, "电流3":sgl, "电流4":sgl})  [unwired: 2 in, 2 out]
                    n1611 = Unbundle(w2083) -> ("电流3"=w2081:sgl)  [unwired: 2 out]
                    n1612 = Multiply(x=w2081, y=1000.0) -> (x*y=w2078:dbl)
                    n1613 = Divide(x=w2080, y=w2078) -> (x/y=w2079:dbl)
                  }
                  frame 3 {
                    n1614 = property on="小信号变比(A/1mv)" class="Clust (严格)"() -> ("Value"=w2089:cluster{"电流2":sgl, "电流3":sgl, "电流4":sgl})  [unwired: 2 in, 2 out]
                    n1615 = Unbundle(w2089) -> ("电流4"=w2087:sgl)  [unwired: 2 out]
                    n1616 = Multiply(x=w2087, y=1000.0) -> (x*y=w2084:dbl)
                    n1617 = Divide(x=w2086, y=w2084) -> (x/y=w2085:dbl)
                  }
                }
                n1618 = call "高精度写.vi"("电压纹波"=w2056, "串口号"=w2055, "电压档位"=w2070, "电流幅值"=w2053, "电流档位值"=w2070, "纹波频率"=w2056, "电流纹波"=w2056, "电流通道"=w2051) -> ("应答"=w2054:string)  [unwired: 7 in]
                n1619 = case shown="\"正确\"" w2054 {
                  tunnel: w2055 -> [_ _ w2099]
                  tunnel: w2052 -> [_ _ w2097]
                  frame "错误", Default {
                    n1620 = property on="提示信息" class="Bool (严格)"("BoolText.Text"="高精度写错误！", "Val(Sgnl)"=TRUE ("提示信息")) -> ()  [unwired: 2 in, 2 out]
                  }
                  frame "超时" {
                    n1621 = property on="提示信息" class="Bool (严格)"("BoolText.Text"="高精度写超时！", "Val(Sgnl)"=TRUE ("提示信息")) -> ()  [unwired: 2 in, 2 out]
                  }
                  frame "正确" {
                    n1622 = property on="误差电流通道" class="Ring (严格)"() -> ("Value"=w2096:u16)  [unwired: 2 in, 2 out]
                    n1623 = case shown="1" w2096 {
                      tunnel: w2096 -> [w2101 w2103 w2105 w2107]
                      tunnel: [w2101 w2103 w2105 w2107] -> w2095
                      tunnel: [w2100 w2102 w2104 w2106] -> w2094
                      frame 0, Default {
                        w2100 = u16 1 items=["电压启动", "电流启动", "全部启动", "UB_outPut_start", "IB_outPut_start", "UC_outPut_start"] ("启动项")
                      }
                      frame 1 {
                        w2102 = u16 3 items=["电压启动", "电流启动", "全部启动", "UB_outPut_start", "IB_outPut_start", "UC_outPut_start"] ("启动项")
                      }
                      frame 2 {
                        w2104 = u16 4 items=["电压启动", "电流启动", "全部启动", "UB_outPut_start", "IB_outPut_start", "UC_outPut_start"] ("启动项")
                      }
                      frame 3 {
                        w2106 = u16 5 items=["电压启动", "电流启动", "全部启动", "UB_outPut_start", "IB_outPut_start", "UC_outPut_start"] ("启动项")
                      }
                    }
                    n1624 = call "输出启动.vi"("电流通道"=w2095, "启动项"=w2094, "串口号"=w2099) -> ("应答"=w2098:string)  [unwired: 2 in]
                    n1625 = case shown="\"正确\"" w2098 {
                      tunnel: w2097 -> [_ _ w2112]
                      frame "错误", Default {
                        n1626 = property on="提示信息" class="Bool (严格)"("BoolText.Text"="输出失败！", "Val(Sgnl)"=TRUE ("提示信息")) -> ()  [unwired: 2 in, 2 out]
                      }
                      frame "超时" {
                        n1627 = property on="提示信息" class="Bool (严格)"("BoolText.Text"="输出超时！", "Val(Sgnl)"=TRUE ("提示信息")) -> ()  [unwired: 2 in, 2 out]
                      }
                      frame "正确" {
                        n1628 = property on="本机表格" class="Tbl (严格)"() -> ("Value"=w2114:string[][])  [unwired: 2 in, 2 out]
                        n1629 = Index Array(array=w2114, index (col)=0 ("禁用的索引 (列)")) -> (element=w2116:string[])  [unwired: 1 in]
                        n1630 = Number To Fractional String(number=0.0 ("数字"), precision (6)=i16 3 ("精度(6)")) -> (F-format string=w2121:string)  [unwired: 2 in]
                        n1631 = Number To Fractional String(number=w2112, precision (6)=i16 3 ("精度(6)")) -> (F-format string=w2122:string)  [unwired: 2 in]
                        n1632 = Replace Array Subset(array=w2116, new element=w2121, index=0 ("索引")) -> (w2119:string[])
                        n1633 = Replace Array Subset(array=w2119, new element=w2122, index=1 ("索引")) -> (w2125:string[])
                        n1634 = Replace Array Subset(array=w2114, new element=w2125, index (col)=0 ("禁用的索引 (列)")) -> (w2124:string[][])  [unwired: 1 in]
                        n1635 = property on="本机表格" class="Tbl (严格)"("Value"=w2124) -> ()  [unwired: 2 in, 2 out]
                      }
                    }
                  }
                }
              }
              frame 2 {
                w2142 = sgl 0.01 ("y")
                w2144 = u32 85 ("电流档位")
                n1636 = property on="误差电流通道" class="Ring (严格)"() -> ("Value"=w2127:u16)  [unwired: 2 in, 2 out]
                n1637 = property on="电压检定点" class="DigNum (严格)"() -> ("Value"=w2141:sgl)  [unwired: 2 in, 2 out]
                n1638 = property on="电流检定点" class="DigNum (严格)"() -> ("Value"=w2143:sgl)  [unwired: 2 in, 2 out]
                n1639 = property on="电压纹波" class="DigNum (严格)"() -> ("Value"=w2133:sgl)  [unwired: 2 in, 2 out]
                n1640 = property on="标定电流" class="DigNum (严格)"() -> ("Value"=w2139:sgl)  [unwired: 2 in, 2 out]
                n1641 = property on="纹波频率" class="DigNum (严格)"() -> ("Value"=w2132:sgl)  [unwired: 2 in, 2 out]
                n1642 = property on="电流纹波" class="DigNum (严格)"() -> ("Value"=w2128:sgl)  [unwired: 2 in, 2 out]
                n1643 = Multiply(x=w2143, y=w2142) -> (x*y=w2140:sgl)
                n1644 = Multiply(x=w2139, y=w2140) -> (x*y=w2130:sgl)
                n1645 = case shown="1" w2127 {
                  tunnel: w2128 -> [w2146 w2151 w2159 w2167]
                  tunnel: [w2146 w2150 w2158 w2166] -> w2129
                  tunnel: w2130 -> [w2145 w2148 w2156 w2164]
                  tunnel: [w2145 w2147 w2155 w2163] -> w2131
                  frame 0, Default {
                  }
                  frame 1 {
                    n1646 = property on="小信号变比(A/1mv)" class="Clust (严格)"() -> ("Value"=w2154:cluster{"电流2":sgl, "电流3":sgl, "电流4":sgl})  [unwired: 2 in, 2 out]
                    n1647 = Unbundle(w2154) -> ("电流2"=w2152:sgl)  [unwired: 2 out]
                    n1648 = Multiply(x=w2152, y=1000.0) -> (x*y=w2149:dbl)
                    n1649 = Divide(x=w2151, y=w2149) -> (x/y=w2150:dbl)
                    n1650 = Divide(x=w2148, y=w2149) -> (x/y=w2147:dbl)
                  }
                  frame 2 {
                    n1651 = property on="小信号变比(A/1mv)" class="Clust (严格)"() -> ("Value"=w2162:cluster{"电流2":sgl, "电流3":sgl, "电流4":sgl})  [unwired: 2 in, 2 out]
                    n1652 = Unbundle(w2162) -> ("电流3"=w2160:sgl)  [unwired: 2 out]
                    n1653 = Multiply(x=w2160, y=1000.0) -> (x*y=w2157:dbl)
                    n1654 = Divide(x=w2159, y=w2157) -> (x/y=w2158:dbl)
                    n1655 = Divide(x=w2156, y=w2157) -> (x/y=w2155:dbl)
                  }
                  frame 3 {
                    n1656 = property on="小信号变比(A/1mv)" class="Clust (严格)"() -> ("Value"=w2170:cluster{"电流2":sgl, "电流3":sgl, "电流4":sgl})  [unwired: 2 in, 2 out]
                    n1657 = Unbundle(w2170) -> ("电流4"=w2168:sgl)  [unwired: 2 out]
                    n1658 = Multiply(x=w2168, y=1000.0) -> (x*y=w2165:dbl)
                    n1659 = Divide(x=w2167, y=w2165) -> (x/y=w2166:dbl)
                    n1660 = Divide(x=w2164, y=w2165) -> (x/y=w2163:dbl)
                  }
                }
                n1661 = property on="额定电压" class="DigNum (严格)"() -> ("Value"=w2138:sgl)  [unwired: 2 in, 2 out]
                n1662 = Multiply(x=w2141, y=w2142) -> (x*y=w2137:sgl)
                n1663 = Multiply(x=w2138, y=w2137) -> (x*y=w2134:sgl)
                n1664 = call "高精度写.vi"("电压幅值"=w2134, "电压纹波"=w2133, "串口号"=w2135, "电压档位"=w2144, "电流幅值"=w2131, "电流档位值"=w2144, "纹波频率"=w2132, "电流纹波"=w2129, "电流通道"=w2127) -> ("应答"=w2136:string)  [unwired: 6 in]
                n1665 = case shown="\"正确\"" w2136 {
                  tunnel: w2135 -> [_ _ w2182]
                  tunnel: w2134 -> [_ _ w2180]
                  tunnel: w2130 -> [_ _ w2179]
                  tunnel: w2133 -> [_ _ w2178]
                  tunnel: w2128 -> [_ _ w2177]
                  tunnel: w2132 -> [_ _ w2176]
                  frame "错误", Default {
                    n1666 = property on="提示信息" class="Bool (严格)"("BoolText.Text"="高精度写错误！", "Val(Sgnl)"=TRUE ("提示信息")) -> ()  [unwired: 2 in, 2 out]
                  }
                  frame "超时" {
                    n1667 = property on="提示信息" class="Bool (严格)"("BoolText.Text"="高精度写超时！", "Val(Sgnl)"=TRUE ("提示信息")) -> ()  [unwired: 2 in, 2 out]
                  }
                  frame "正确" {
                    w2183 = u16 2 items=["电压启动", "电流启动", "全部启动"] ("启动项")
                    n1668 = property on="误差电流通道" class="Ring (严格)"() -> ("Value"=w2175:u16)  [unwired: 2 in, 2 out]
                    n1669 = call "输出启动.vi"("电流通道"=w2175, "启动项"=w2183, "串口号"=w2182) -> ("应答"=w2181:string)  [unwired: 2 in]
                    n1670 = case shown="\"正确\"" w2181 {
                      tunnel: w2180 -> [_ _ w2195]
                      tunnel: w2179 -> [_ _ w2194]
                      tunnel: w2178 -> [_ _ w2193]
                      tunnel: w2177 -> [_ _ w2192]
                      tunnel: w2176 -> [_ _ w2191]
                      frame "错误", Default {
                        n1671 = property on="提示信息" class="Bool (严格)"("BoolText.Text"="输出失败！", "Val(Sgnl)"=TRUE ("提示信息")) -> ()  [unwired: 2 in, 2 out]
                      }
                      frame "超时" {
                        n1672 = property on="提示信息" class="Bool (严格)"("BoolText.Text"="输出超时！", "Val(Sgnl)"=TRUE ("提示信息")) -> ()  [unwired: 2 in, 2 out]
                      }
                      frame "正确" {
                        n1673 = property on="本机表格" class="Tbl (严格)"() -> ("Value"=w2206:string[][])  [unwired: 2 in, 2 out]
                        n1674 = Index Array(array=w2206, index (col)=0 ("禁用的索引 (列)")) -> (element=w2208:string[])  [unwired: 1 in]
                        n1675 = Number To Fractional String(number=w2195, precision (6)=i16 3 ("精度(6)")) -> (F-format string=w2213:string)  [unwired: 2 in]
                        n1676 = Number To Fractional String(number=w2194, precision (6)=i16 3 ("精度(6)")) -> (F-format string=w2214:string)  [unwired: 2 in]
                        n1677 = Number To Fractional String(number=w2193, precision (6)=i16 3 ("精度(6)")) -> (F-format string=w2205:string)  [unwired: 2 in]
                        n1678 = Number To Fractional String(number=w2192, precision (6)=i16 3 ("精度(6)")) -> (F-format string=w2202:string)  [unwired: 2 in]
                        n1679 = Number To Fractional String(number=w2191, precision (6)=i16 3 ("精度(6)")) -> (F-format string=w2201:string)  [unwired: 2 in]
                        n1680 = Replace Array Subset(array=w2208, new element=w2213, index=0 ("索引")) -> (w2211:string[])
                        n1681 = Replace Array Subset(array=w2211, new element=w2214, index=1 ("索引")) -> (w2199:string[])
                        n1682 = Replace Array Subset(array=w2199, new element=w2205, index=2 ("索引")) -> (w2198:string[])
                        n1683 = Replace Array Subset(array=w2198, new element=w2202, index=3 ("索引")) -> (w2197:string[])
                        n1684 = Replace Array Subset(array=w2197, new element=w2201, index=4 ("索引")) -> (w2196:string[])
                        n1685 = Replace Array Subset(array=w2206, new element=w2196, index (col)=0 ("禁用的索引 (列)")) -> (w2216:string[][])  [unwired: 1 in]
                        n1686 = property on="本机表格" class="Tbl (严格)"("Value"=w2216) -> ()  [unwired: 2 in, 2 out]
                      }
                    }
                  }
                }
              }
            }
          }
        }
      }
      event "UI检定操作.保存方案", "UI检定操作.导入方案": Value Change {
        n1687 = event-data() -> ("CtlRef"=w2218:refnum<vi>, "NewVal"=w2219:bool)  [unwired: 1 in, 3 out]
        n1688 = case shown="真" w2219 {
          tunnel: w2218 -> [_ w2221]
          frame False {
          }
          frame True {
            n1689 = property class="Bool (严格)"(reference=w2221) -> ("BoolText.Text"=w2220:string)  [unwired: 1 in, 2 out]
            n1690 = case shown="\"导入方案\"" w2220 {
              frame "假", Default {
              }
              frame "保存方案" {
                n1691 = property on="UI检定表格" class="Tbl (严格)"() -> ("Value"=w2222:string[][])  [unwired: 2 in, 2 out]
                n1692 = call-poly <vilib>:"Write To Spreadsheet File.vi"("2D data"=w2222) -> ()  [unwired: 7 in, 1 out]
              }
              frame "导入方案" {
                n1693 = call-poly <vilib>:"Read From Spreadsheet File.vi"() -> ("all rows"=w2225:string[][], "new file path (Not A Path if cancelled)"=w2224:path)  [unwired: 7 in, 3 out]
                n1694 = Strip Path(path=w2224) -> (name=w2223:string)  [unwired: 1 out]
                n1695 = property on="UI检定表格" class="Tbl (严格)"("Val(Sgnl)"=w2225) -> ()  [unwired: 2 in, 2 out]
                n1696 = property on="UI检定表格" class="Tbl (严格)"("Caption.Text"=w2223) -> ()  [unwired: 2 in, 2 out]
              }
            }
          }
        }
      }
      event "UI检定操作.计算误差": Value Change {
        n1697 = event-data() -> ("NewVal"=w2227:bool)  [unwired: 1 in]
        n1698 = property on="误差显示表" class="Tbl (严格)"() -> ("Row Headers[]"=w2230:string[])  [unwired: 2 in, 2 out]
        n1699 = property on="UI检定表格" class="Tbl (严格)"() -> ("Value"=w2228:string[][])  [unwired: 2 in, 2 out]
        n1700 = property on="误差显示表" class="Tbl (严格)"() -> ("Value"=w2229:string[][])  [unwired: 2 in, 2 out]
        n1701 = property on="UI行数" class="DigNum (严格)"() -> ("Value"=w2226:i32)  [unwired: 2 in, 2 out]
        n1702 = case shown="真" w2227 {
          tunnel: w2230 -> [_ w2253]
          tunnel: w2229 -> [_ w2235]
          tunnel: w2228 -> [_ w2237]
          tunnel: w2226 -> [_ w2232]
          frame False {
          }
          frame True {
            n1703 = for {
              N: 15 -> [_]
              tunnel: [w2255] -> w2233
              i -> [w2256]
              n1704 = for {
                N: 6 -> [_]
                tunnel: w2256 -> [w2259]
                tunnel: [w2258] -> w2255 mode=indexing
                i -> [w2257]
                n1705 = property on="误差显示表" class="Tbl (严格)"() -> ("Active Cell"=w2264:T17)  [unwired: 2 in, 2 out]
                n1706 = Bundle By Name(cluster=w2264, "Row"=w2259, "Column"=w2257) -> (w2258:T17)
                n1707 = property on="误差显示表" class="Tbl (严格)"("Active Cell"=w2258) -> (error out=w2263:errorcluster)  [unwired: 2 in, 1 out]
                n1708 = property on="误差显示表" class="Tbl (严格)"(error in=w2263) -> ("Cell BG Color"=w2262:u32)  [unwired: 1 in, 2 out]
                n1709 = Not Equal?(x=w2262, y=u32 16448250) -> (x != y?=w2260:bool)
                n1710 = case shown="真" w2260 {
                  frame False {
                  }
                  frame True {
                    n1711 = property on="误差显示表" class="Tbl (严格)"("Cell BG Color"=u32 16448250) -> ()  [unwired: 2 in, 2 out]
                  }
                }
              }
            }
            n1712 = for {
              N: w2232 -> [_]
              tunnel: w2253 -> [w2334] mode=indexing
              tunnel: w2235 -> [w2329] mode=indexing
              tunnel: [w2314] -> w2252 mode=indexing
              tunnel: [w2313] -> w2249 mode=indexing
              tunnel: [w2312] -> w2248 mode=indexing
              tunnel: [w2307] -> w2243 mode=indexing
              tunnel: [w2306] -> w2241 mode=indexing
              tunnel: [w2305] -> w2239 mode=indexing
              tunnel: w2237 -> [w2302] mode=indexing
              tunnel: [w2300] -> w2236 mode=indexing
              w2308 = sgl 100.0 ("默认(0 DBL)")
              w2315 = i16 3 ("精度(6)")
              n1713 = Index Array(array=w2329, index=4 ("索引")) -> (element=w2323:string)
              n1714 = Index Array(array=w2302, index=2 ("索引")) -> (element=w2301:string)
              n1715 = Index Array(array=w2329, index=0 ("索引")) -> (element=w2325:string)
              n1716 = Index Array(array=w2329, index=2 ("索引")) -> (element=w2324:string)
              n1717 = Fract/Exp String To Number(string=w2334, default (0 dbl)=sgl 0.0 ("默认(0 DBL)")) -> (number=w2316:sgl)  [unwired: 2 in, 1 out]
              n1718 = Fract/Exp String To Number(string=w2325, default (0 dbl)=sgl 0.0 ("默认(0 DBL)")) -> (number=w2322:sgl)  [unwired: 2 in, 1 out]
              n1719 = Fract/Exp String To Number(string=w2324, default (0 dbl)=sgl 0.0 ("默认(0 DBL)")) -> (number=w2321:sgl)  [unwired: 2 in, 1 out]
              n1720 = Fract/Exp String To Number(string=w2323, default (0 dbl)=sgl 0.0 ("默认(0 DBL)")) -> (number=w2320:sgl)  [unwired: 2 in, 1 out]
              n1721 = Fract/Exp String To Number(string=w2301, default (0 dbl)=sgl 0.0 ("默认(0 DBL)")) -> (number=w2300:sgl)  [unwired: 2 in, 1 out]
              n1722 = Subtract(x=w2322, y=w2316) -> (x-y=w2319:sgl)
              n1723 = Subtract(x=w2321, y=w2316) -> (x-y=w2317:sgl)
              n1724 = Subtract(x=w2320, y=w2316) -> (x-y=w2318:sgl)
              n1725 = Divide(x=w2317, y=w2316) -> (x/y=w2310:sgl)
              n1726 = Divide(x=w2318, y=w2316) -> (x/y=w2309:sgl)
              n1727 = Divide(x=w2319, y=w2316) -> (x/y=w2311:sgl)
              n1728 = Multiply(x=w2308, y=w2311) -> (x*y=w2307:sgl)
              n1729 = Multiply(x=w2308, y=w2310) -> (x*y=w2306:sgl)
              n1730 = Multiply(x=w2308, y=w2309) -> (x*y=w2305:sgl)
              n1731 = Number To Fractional String(number=w2307, precision (6)=w2315) -> (F-format string=w2314:string)  [unwired: 2 in]
              n1732 = Number To Fractional String(number=w2306, precision (6)=w2315) -> (F-format string=w2313:string)  [unwired: 2 in]
              n1733 = Number To Fractional String(number=w2305, precision (6)=w2315) -> (F-format string=w2312:string)  [unwired: 2 in]
            }
            n1734 = property on="误差显示表" class="Tbl (严格)"("Value"=w2235) -> (error out=w2234:errorcluster)  [unwired: 2 in, 1 out]
            n1735 = Replace Array Subset(array=w2235, new element=w2252, index (col)=1 ("索引")) -> (w2251:string[][])  [unwired: 1 in]
            n1736 = Replace Array Subset(array=w2251, new element=w2249, index (col)=3 ("索引")) -> (w2250:string[][])  [unwired: 1 in]
            n1737 = Replace Array Subset(array=w2250, new element=w2248, index (col)=5 ("索引")) -> (w2244:string[][])  [unwired: 1 in]
            n1738 = property on="误差显示表" class="Tbl (严格)"(error in=w2234, "Value"=w2244) -> ()  [unwired: 1 in, 2 out]
            n1739 = Absolute Value(x=w2243) -> (abs(x)=w2242:sgl[])
            n1740 = Absolute Value(x=w2241) -> (abs(x)=w2240:sgl[])
            n1741 = Absolute Value(x=w2239) -> (abs(x)=w2238:sgl[])
            n1742 = for {
              N: w2232 -> [_]
              tunnel: w2242 -> [w2276] mode=indexing
              tunnel: w2240 -> [w2275] mode=indexing
              tunnel: w2238 -> [w2274] mode=indexing
              tunnel: w2236 -> [w2269] mode=indexing
              tunnel: w2233 -> [w2268] mode=indexing
              i -> [w2270]
              n1743 = Greater?(x=w2274, y=w2269) -> (0:w2279:bool)
              n1744 = Greater?(x=w2276, y=w2269) -> (0:w2278:bool)
              n1745 = Greater?(x=w2275, y=w2269) -> (0:w2277:bool)
              n1746 = case shown="真" w2278 {
                tunnel: 1 ("索引") -> [_ w2298]
                tunnel: w2270 -> [_ w2299]
                tunnel: w2268 -> [w2293 w2295]
                tunnel: [w2293 w2294] -> w2267
                frame False {
                }
                frame True {
                  n1747 = Bundle By Name(cluster=w2295, "Row"=w2299, "Column"=w2298) -> (w2294:T17)
                  n1748 = property on="误差显示表" class="Tbl (严格)"("Active Cell"=w2294) -> (error out=w2297:errorcluster)  [unwired: 2 in, 1 out]
                  n1749 = property on="误差显示表" class="Tbl (严格)"(error in=w2297, "Cell BG Color"=u32 16448250) -> ()  [unwired: 1 in, 2 out]
                }
              }
              n1750 = case shown="真" w2277 {
                tunnel: 3 ("索引") -> [_ w2291]
                tunnel: w2270 -> [_ w2292]
                tunnel: w2267 -> [w2286 w2288]
                tunnel: [w2286 w2287] -> w2266
                frame False {
                }
                frame True {
                  n1751 = Bundle By Name(cluster=w2288, "Row"=w2292, "Column"=w2291) -> (w2287:T17)
                  n1752 = property on="误差显示表" class="Tbl (严格)"("Active Cell"=w2287) -> (error out=w2290:errorcluster)  [unwired: 2 in, 1 out]
                  n1753 = property on="误差显示表" class="Tbl (严格)"(error in=w2290, "Cell BG Color"=u32 16448250) -> ()  [unwired: 1 in, 2 out]
                }
              }
              n1754 = case shown="真" w2279 {
                tunnel: 5 ("索引") -> [_ w2284]
                tunnel: w2270 -> [_ w2285]
                tunnel: w2266 -> [_ w2280]
                frame False {
                }
                frame True {
                  n1755 = Bundle By Name(cluster=w2280, "Row"=w2285, "Column"=w2284) -> (w2281:T17)
                  n1756 = property on="误差显示表" class="Tbl (严格)"("Active Cell"=w2281) -> (error out=w2283:errorcluster)  [unwired: 2 in, 1 out]
                  n1757 = property on="误差显示表" class="Tbl (严格)"(error in=w2283, "Cell BG Color"=u32 16448250) -> ()  [unwired: 1 in, 2 out]
                }
              }
            }
          }
        }
      }
      event "控制选项卡": Value Change {
        n1758 = event-data() -> ("NewVal"=w2335:T1)  [unwired: 1 in, 4 out]
        n1759 = case shown="\"误差计算\"" w2335 {
          frame "输出控制", Default {
            n1760 = local write "result_Tab"(0) -> ()
            n1761 = property on="本机表格" class="Tbl (严格)"("Visible"=FALSE) -> ()  [unwired: 2 in, 2 out]
            n1762 = property on="result_Tab" class="TabCtl (严格)"("Visible"=TRUE) -> ()  [unwired: 2 in, 2 out]
          }
          frame "电能检定" {
            n1763 = local write "result_Tab"(1) -> ()
            n1764 = property on="result_Tab" class="TabCtl (严格)"("Visible"=TRUE) -> ()  [unwired: 2 in, 2 out]
            n1765 = property on="误差显示表" class="Tbl (严格)"("Column Headers[]"=string[] ["表1电能(KWh)", "误差(%)", "表2电能(KWh)", "误差(%)", "表3电能(KWh)", "误差(%)"] ("列首字符串[]")) -> ()  [unwired: 2 in, 2 out]
            n1766 = property on="单点显示表" class="Tbl (严格)"("Row Headers[]"=string[] ["脉冲输入数", "脉冲输入功率(W)", "脉冲输入电能(KWh)", "标准偏差值(KWh)", "电能误差(%)"] ("行首字符串[]")) -> ()  [unwired: 2 in, 2 out]
            n1767 = property on="本机表格" class="Tbl (严格)"("Visible"=TRUE) -> ()  [unwired: 2 in, 2 out]
            n1768 = property on="E检定表格" class="Tbl (严格)"() -> ("Value"=w2343:string[][])  [unwired: 2 in, 2 out]
            n1769 = property on="单点检定" class="Bool (严格)"() -> ("Value"=w2344:bool)  [unwired: 2 in, 2 out]
            n1770 = call "表格行数.vi"("E检定表格"=w2343) -> ("行数"=w2345:i32)  [unwired: 2 in]
            n1771 = case shown="真" w2344 {
              tunnel: w2345 -> [w2352 _]
              tunnel: w2343 -> [w2351 _]
              frame False {
                n1772 = property on="电能显示表" class="Tbl (严格)"("Visible"=TRUE ("可见")) -> ()  [unwired: 2 in, 2 out]
                n1773 = property on="单点显示表" class="Tbl (严格)"("Visible"=FALSE ("可见")) -> ()  [unwired: 2 in, 2 out]
                n1774 = property on="误差显示表" class="Tbl (严格)"("Visible"=FALSE ("可见")) -> ()  [unwired: 2 in, 2 out]
                n1775 = for {
                  N: w2352 -> [_]
                  tunnel: w2351 -> [w2373] mode=indexing
                  tunnel: [w2358] -> w2350 mode=indexing
                  w2355 = sgl 0.01
                  w2363 = i16 2 ("精度(6)")
                  w2368 = sgl 0.0 ("默认(0 DBL)")
                  n1776 = Index Array(array=w2373, index=0 ("索引")) -> (element=w2372:string)
                  n1777 = Index Array(array=w2373, index=1 ("索引")) -> (element=w2371:string)
                  n1778 = Index Array(array=w2373, index=2 ("索引")) -> (element=w2370:string)
                  n1779 = Index Array(array=w2373, index=3 ("索引")) -> (element=w2369:string)
                  n1780 = Fract/Exp String To Number(string=w2372, default (0 dbl)=w2368) -> (number=w2367:sgl)  [unwired: 2 in, 1 out]
                  n1781 = Fract/Exp String To Number(string=w2371, default (0 dbl)=w2368) -> (number=w2364:sgl)  [unwired: 2 in, 1 out]
                  n1782 = Fract/Exp String To Number(string=w2370, default (0 dbl)=w2368) -> (number=w2366:sgl)  [unwired: 2 in, 1 out]
                  n1783 = Fract/Exp String To Number(string=w2369, default (0 dbl)=w2368) -> (number=w2365:sgl)  [unwired: 2 in, 1 out]
                  n1784 = Multiply(x=w2366, y=w2365) -> (x*y=w2354:sgl)
                  n1785 = Multiply(x=w2367, y=w2364) -> (x*y=w2357:sgl)
                  n1786 = Multiply(x=w2355, y=w2357) -> (x*y=w2356:sgl)
                  n1787 = Multiply(x=w2355, y=w2354) -> (x*y=w2353:sgl)
                  n1788 = Number To Fractional String(number=w2353, precision (6)=w2363) -> (F-format string=w2360:string)  [unwired: 2 in]
                  n1789 = Number To Fractional String(number=w2356, precision (6)=w2363) -> (F-format string=w2362:string)  [unwired: 2 in]
                  n1790 = Concatenate Strings(w2362, "V" ("字符串"), w2360, "A" ("字符串")) -> (w2358:string)
                }
                n1791 = property on="误差显示表" class="Tbl (严格)"("Row Headers[]"=w2350) -> ()  [unwired: 2 in, 2 out]
              }
              frame True {
                n1792 = local write "result_Tab"(3) -> ()
                n1793 = property on="电能显示表" class="Tbl (严格)"("Visible"=FALSE ("可见")) -> ()  [unwired: 2 in, 2 out]
                n1794 = property on="误差显示表" class="Tbl (严格)"("Visible"=FALSE ("可见")) -> ()  [unwired: 2 in, 2 out]
                n1795 = property on="单点显示表" class="Tbl (严格)"("Visible"=TRUE ("可见")) -> ()  [unwired: 2 in, 2 out]
              }
            }
            n1796 = property on="E行数" class="DigNum (严格)"("Value"=w2345) -> ()  [unwired: 2 in, 2 out]
          }
          frame "误差计算" {
            w2390 = T17 {"Row"=0, "Column"=0} ("输入簇")
            n1797 = local write "result_Tab"(2) -> ()
            n1798 = property on="result_Tab" class="TabCtl (严格)"("Visible"=TRUE) -> ()  [unwired: 2 in, 2 out]
            n1799 = property on="UI检定表格" class="Tbl (严格)"("Cell BG Color"=u32 16777226) -> (error out=w2387:errorcluster)  [unwired: 2 in, 1 out]
            n1800 = property on="误差显示表" class="Tbl (严格)"("Column Headers[]"=string[] ["表1电压(V)", "误差(%)", "表2电压(V)", "误差(%)", "表3电压(V)", "误差(%)"] ("列首字符串[]")) -> ()  [unwired: 2 in, 2 out]
            n1801 = Unbundle By Name(w2390) -> ("Row"=w2389:i32)
            n1802 = property on="UI检定表格" class="Tbl (严格)"(error in=w2387, "Active Cell"=w2390) -> (error out=w2388:errorcluster)  [unwired: 1 in, 1 out]
            n1803 = property on="单点显示表" class="Tbl (严格)"("Visible"=FALSE ("可见")) -> ()  [unwired: 2 in, 2 out]
            n1804 = property on="误差显示表" class="Tbl (严格)"("Visible"=TRUE ("可见")) -> ()  [unwired: 2 in, 2 out]
            n1805 = property on="电能显示表" class="Tbl (严格)"("Visible"=FALSE ("可见")) -> ()  [unwired: 2 in, 2 out]
            n1806 = property on="本机表格" class="Tbl (严格)"("Visible"=TRUE) -> ()  [unwired: 2 in, 2 out]
            n1807 = property on="UI当前行" class="DigNum (严格)"("Value"=w2389) -> ()  [unwired: 2 in, 2 out]
            n1808 = property on="UI检定表格" class="Tbl (严格)"() -> ("Value"=w2393:string[][])  [unwired: 2 in, 2 out]
            n1809 = property on="UI检定表格" class="Tbl (严格)"(error in=w2388, "Cell BG Color"=u32 16763457) -> ()  [unwired: 1 in, 2 out]
            n1810 = call "表格行数.vi"("E检定表格"=w2393) -> ("行数"=w2392:i32)  [unwired: 2 in]
            n1811 = for {
              N: w2392 -> [_]
              tunnel: w2393 -> [w2408] mode=indexing
              tunnel: [w2398] -> w2394 mode=indexing
              w2404 = 0.0
              n1812 = Index Array(array=w2408, index=0 ("索引")) -> (element=w2407:string)
              n1813 = Index Array(array=w2408, index=1 ("索引")) -> (element=w2406:string)
              n1814 = Fract/Exp String To Number(string=w2407, default (0 dbl)=w2404) -> (number=w2403:dbl)  [unwired: 2 in, 1 out]
              n1815 = Fract/Exp String To Number(string=w2406, default (0 dbl)=w2404) -> (number=w2400:dbl)  [unwired: 2 in, 1 out]
              n1816 = Multiply(x=w2400, y=0.01) -> (x*y=w2402:dbl)
              n1817 = Multiply(x=w2403, y=w2402) -> (x*y=w2401:dbl)
              n1818 = Number To Fractional String(number=w2401, precision (6)=i16 2 ("精度(6)")) -> (F-format string=w2398:string)  [unwired: 2 in]
            }
            n1819 = property on="UI行数" class="DigNum (严格)"("Value"=w2392) -> ()  [unwired: 2 in, 2 out]
            n1820 = property on="误差显示表" class="Tbl (严格)"("Row Headers[]"=w2394) -> ()  [unwired: 2 in, 2 out]
          }
          frame "潜动起动" {
            n1821 = property on="result_Tab" class="TabCtl (严格)"("Visible"=TRUE) -> ()  [unwired: 2 in, 2 out]
            n1822 = local write "result_Tab"(3) -> ()
            n1823 = property on="单点显示表" class="Tbl (严格)"("Visible"=TRUE ("可见")) -> ()  [unwired: 2 in, 2 out]
            n1824 = property on="误差显示表" class="Tbl (严格)"("Visible"=FALSE ("可见")) -> ()  [unwired: 2 in, 2 out]
            n1825 = property on="电能显示表" class="Tbl (严格)"("Visible"=FALSE ("可见")) -> ()  [unwired: 2 in, 2 out]
            n1826 = property on="本机表格" class="Tbl (严格)"("Visible"=TRUE) -> ()  [unwired: 2 in, 2 out]
            n1827 = Initialize Array("", 5 ("维数大小"), 3 ("维数大小")) -> (w2418:string[][])
            n1828 = property on="单点显示表" class="Tbl (严格)"("Value"=w2418) -> ()  [unwired: 2 in, 2 out]
            n1829 = property on="单点显示表" class="Tbl (严格)"("Row Headers[]"=string[] ["脉冲输入数", "脉冲输入功率(W)", "脉冲输入电能(KWh)"] ("行首字符串[]")) -> ()  [unwired: 2 in, 2 out]
          }
          frame "报表生成" {
            n1830 = property on="本机表格" class="Tbl (严格)"("Visible"=FALSE) -> ()  [unwired: 2 in, 2 out]
            n1831 = local write "result_Tab"(4) -> ()
            n1832 = property on="result_Tab" class="TabCtl (严格)"("Visible"=FALSE) -> ()  [unwired: 2 in, 2 out]
            n1833 = Get Date/Time In Seconds() -> (seconds since 1Jan1904=w2430:timestamp)
            n1834 = Format Date/Time String(time format string (%c)="%Y%m%d-" ("时间格式字符串(%c)"), seconds (now)=w2430) -> (date/time string=w2427:string)  [unwired: 1 in]
            n1835 = Format Date/Time String(time format string (%c)="%H-%M-%S" ("时间格式字符串(%c)"), seconds (now)=w2430) -> (date/time string=w2426:string)  [unwired: 1 in]
            n1836 = Concatenate Strings(w2427, w2426) -> (w2425:string)
            n1837 = property on="报表名称" class="Str"("Value"=w2425) -> ()  [unwired: 2 in, 2 out]
          }
          frame "参数设置" {
            n1838 = local write "result_Tab"(4) -> ()
            n1839 = property on="result_Tab" class="TabCtl (严格)"("Visible"=FALSE) -> ()  [unwired: 2 in, 2 out]
            n1840 = property on="本机表格" class="Tbl (严格)"("Visible"=FALSE) -> ()  [unwired: 2 in, 2 out]
            n1841 = property on="串口灯" class="Bool (严格)"() -> ("Value"=w2434:bool)  [unwired: 2 in, 2 out]
            n1842 = case shown="真" w2434 {
              frame False {
              }
              frame True {
                n1843 = property on="串口号" class="VISAName"() -> ("Value"=w2435:refnum<visa-resource-name>)  [unwired: 2 in, 2 out]
                n1844 = stacked-sequence {
                  tunnel: w2435 -> [w2436 _ w2445 _ w2454]
                  frame #0 {
                    n1845 = property on="脉冲输入口" class="Ring (严格)"() -> ("Value"=w2438:u8)  [unwired: 2 in, 2 out]
                    n1846 = call "读电表参数.vi"("脉冲输入口"=w2438, "串口号"=w2436) -> ("应答"=w2437:string)  [unwired: 3 in]
                    n1847 = case shown="\"读电能表\"" w2437 {
                      frame Default {
                      }
                      frame "超时" {
                        n1848 = property on="提示信息" class="Bool (严格)"("BoolText.Text"="读电能表参数超时！", "Val(Sgnl)"=TRUE ("提示信息")) -> ()  [unwired: 2 in, 2 out]
                      }
                      frame "错误" {
                        n1849 = property on="提示信息" class="Bool (严格)"("BoolText.Text"="读电能表参数错误！", "Val(Sgnl)"=TRUE ("提示信息")) -> ()  [unwired: 2 in, 2 out]
                      }
                      frame "读电能表" {
                        n1850 = global read "程序全局.vi" "电能表参数"() -> (w2443:T13)
                        n1851 = property on="电能表参数" class="Clust (严格)"("Value"=w2443) -> ()  [unwired: 2 in, 2 out]
                      }
                    }
                  }
                  frame #1 {
                    n1852 = Wait (ms)(milliseconds to wait=u32 200 ("等待时间（毫秒）")) -> ()  [unwired: 1 out]
                  }
                  frame #2 {
                    n1853 = call "读本机参数.vi"("串口号"=w2445) -> ("应答"=w2446:string)  [unwired: 2 in]
                    n1854 = case shown="\"读本机表\"" w2446 {
                      frame "假", Default {
                      }
                      frame "超时" {
                        n1855 = property on="提示信息" class="Bool (严格)"("BoolText.Text"="读本机表参数超时！", "Val(Sgnl)"=TRUE ("提示信息")) -> ()  [unwired: 2 in, 2 out]
                      }
                      frame "错误" {
                        n1856 = property on="提示信息" class="Bool (严格)"("BoolText.Text"="读本机表参数错误！", "Val(Sgnl)"=TRUE ("提示信息")) -> ()  [unwired: 2 in, 2 out]
                      }
                      frame "读本机表" {
                        n1857 = global read "程序全局.vi" "本机表参数"() -> (w2451:cluster{"有功常数":i32, "无功常数":i32, "输出类型":i32})
                        n1858 = property on="本机表参数" class="Clust (严格)"("Value"=w2451) -> ()  [unwired: 2 in, 2 out]
                      }
                    }
                  }
                  frame #3 {
                    n1859 = Wait (ms)(milliseconds to wait=u32 200 ("等待时间（毫秒）")) -> ()  [unwired: 1 out]
                  }
                  frame #4 {
                    n1860 = call "读小信号变比.vi"("串口号"=w2454) -> ("应答"=w2453:string)  [unwired: 10 in]
                    n1861 = case shown="\"读小信号\"" w2453 {
                      frame "假", Default {
                      }
                      frame "超时" {
                        n1862 = property on="提示信息" class="Bool (严格)"("BoolText.Text"="读小信号超时！", "Val(Sgnl)"=TRUE ("提示信息")) -> ()  [unwired: 2 in, 2 out]
                      }
                      frame "错误" {
                        n1863 = property on="提示信息" class="Bool (严格)"("BoolText.Text"="读小信号错误！", "Val(Sgnl)"=TRUE ("提示信息")) -> ()  [unwired: 2 in, 2 out]
                      }
                      frame "读小信号" {
                        n1864 = global read "程序全局.vi" "小信号变比"() -> (w2459:cluster{"UB":sgl, "IB":sgl, "UC":sgl})
                        n1865 = local write "小信号变比(A/1mv)"(w2459) -> ()
                      }
                    }
                  }
                }
              }
            }
          }
        }
      }
      event "电能表设置.表读参数", "电能表设置.表写参数": Value Change {
        n1866 = event-data() -> ("CtlRef"=w2460:refnum<vi>, "NewVal"=w2461:bool)  [unwired: 1 in, 3 out]
        n1867 = stacked-sequence {
          tunnel: w2460 -> [_ w2464]
          frame #0 {
            n1868 = Wait (ms)(milliseconds to wait=u32 200 ("等待时间（毫秒）")) -> ()  [unwired: 1 out]
          }
          frame #1 {
            n1869 = property class="Bool (严格)"(reference=w2464, "Value"=FALSE ("值")) -> ()  [unwired: 1 in, 2 out]
          }
        }
        n1870 = case shown="真" w2461 {
          tunnel: w2460 -> [_ w2467]
          frame False {
          }
          frame True {
            n1871 = property class="Bool (严格)"(reference=w2467) -> ("BoolText.Text"=w2466:string)  [unwired: 1 in, 2 out]
            n1872 = property on="串口号" class="VISAName"() -> ("Value"=w2465:refnum<visa-resource-name>)  [unwired: 2 in, 2 out]
            n1873 = case shown="\"读参数\"" w2466 {
              tunnel: w2465 -> [_ w2470 w2487]
              frame "假", Default {
              }
              frame "读参数" {
                n1874 = property on="脉冲输入口" class="Ring (严格)"() -> ("Value"=w2468:u8)  [unwired: 2 in, 2 out]
                n1875 = call "读电表参数.vi"("脉冲输入口"=w2468, "串口号"=w2470) -> ("应答"=w2469:string)  [unwired: 3 in]
                n1876 = case shown="默认" w2469 {
                  tunnel: w2468 -> [_ _ _ w2479]
                  frame Default {
                  }
                  frame "超时" {
                    n1877 = property on="提示信息" class="Bool (严格)"("BoolText.Text"="读取超时！", "Val(Sgnl)"=TRUE ("提示信息")) -> ()  [unwired: 2 in, 2 out]
                  }
                  frame "错误" {
                    n1878 = property on="提示信息" class="Bool (严格)"("BoolText.Text"="读取错误！", "Val(Sgnl)"=TRUE ("提示信息")) -> ()  [unwired: 2 in, 2 out]
                  }
                  frame "读电能表" {
                    n1879 = global read "程序全局.vi" "电能表参数"() -> (w2478:T13)
                    n1880 = global read "程序全局.vi" "脉冲输入口"() -> (w2481:u8)
                    n1881 = property on="电能表参数" class="Clust (严格)"("Value"=w2478) -> ()  [unwired: 2 in, 2 out]
                    n1882 = property on="脉冲输入口" class="Ring (严格)"("Value"=w2481) -> ()  [unwired: 2 in, 2 out]
                    n1883 = property on="提示信息" class="Bool (严格)"("BoolText.Text"="读取正确！", "Val(Sgnl)"=TRUE ("提示信息")) -> ()  [unwired: 2 in, 2 out]
                    n1884 = global read "程序全局.vi" "电能表参数数组"() -> (w2480:T18)
                    n1885 = Replace Array Subset(array=w2480, new element=w2478, index=w2479) -> (w2477:T18)
                    n1886 = global write "程序全局.vi" "电能表参数数组"(w2477) -> ()
                  }
                }
              }
              frame "写参数" {
                n1887 = global read "程序全局.vi" "电能表参数数组"() -> (w2485:T18)
                n1888 = property on="电能表参数" class="Clust (严格)"() -> ("Value"=w2483:T13)  [unwired: 2 in, 2 out]
                n1889 = local read "脉冲输入口"() -> (w2484:u8)
                n1890 = Replace Array Subset(array=w2485, new element=w2483, index=w2484) -> (w2482:T18)
                n1891 = global write "程序全局.vi" "电能表参数数组"(w2482) -> ()
                n1892 = call "设置电能表.vi"("电能表参数"=w2483, "脉冲输入口"=w2484, "串口号"=w2487) -> ("应答"=w2486:string)  [unwired: 4 in]
                n1893 = case shown="\"超时\"" w2486 {
                  frame "假", Default {
                  }
                  frame "超时" {
                    n1894 = property on="提示信息" class="Bool (严格)"("BoolText.Text"="写入超时！", "Val(Sgnl)"=TRUE ("提示信息")) -> ()  [unwired: 2 in, 2 out]
                  }
                  frame "错误" {
                    n1895 = property on="提示信息" class="Bool (严格)"("BoolText.Text"="写入错误！", "Val(Sgnl)"=TRUE ("提示信息")) -> ()  [unwired: 2 in, 2 out]
                  }
                  frame "正确" {
                    n1896 = property on="提示信息" class="Bool (严格)"("BoolText.Text"="写入成功！", "Val(Sgnl)"=TRUE ("提示信息")) -> ()  [unwired: 2 in, 2 out]
                  }
                }
              }
            }
          }
        }
      }
      event "脉冲输入口": Value Change {
        n1897 = event-data() -> ()  [unwired: 1 in, 5 out]
        n1898 = property on="串口灯" class="Bool (严格)"() -> ("Value"=w2494:bool)  [unwired: 2 in, 2 out]
        n1899 = case shown="真" w2494 {
          frame False {
          }
          frame True {
            n1900 = disable-structure shown="禁用" {
              frame Disabled {
                n1901 = property on="脉冲输入口" class="Ring (严格)"() -> ("Value"=w2498:u8)  [unwired: 2 in, 2 out]
                n1902 = property on="串口号" class="VISAName"() -> ("Value"=w2496:refnum<visa-resource-name>)  [unwired: 2 in, 2 out]
                n1903 = call "读电表参数.vi"("脉冲输入口"=w2498, "串口号"=w2496) -> ("应答"=w2497:string)  [unwired: 3 in]
                n1904 = case shown="\"读电能表\"" w2497 {
                  frame Default {
                  }
                  frame "超时" {
                    n1905 = property on="提示信息" class="Bool (严格)"("BoolText.Text"="读电能表参数超时！", "Val(Sgnl)"=TRUE ("提示信息")) -> ()  [unwired: 2 in, 2 out]
                  }
                  frame "错误" {
                    n1906 = property on="提示信息" class="Bool (严格)"("BoolText.Text"="读电能表参数错误！", "Val(Sgnl)"=TRUE ("提示信息")) -> ()  [unwired: 2 in, 2 out]
                  }
                  frame "读电能表" {
                    n1907 = global read "程序全局.vi" "电能表参数"() -> (w2503:T13)
                    n1908 = property on="电能表参数" class="Clust (严格)"("Value"=w2503) -> ()  [unwired: 2 in, 2 out]
                  }
                }
              }
              frame Enabled {
              }
            }
            n1909 = property on="表读参数" class="Bool (严格)"("Val(Sgnl)"=TRUE ("值(信号)")) -> ()  [unwired: 2 in, 2 out]
          }
        }
      }
      event "本机表设置.本机读参数", "本机表设置.本机写参数": Value Change {
        n1910 = event-data() -> ("CtlRef"=w2505:refnum<vi>, "NewVal"=w2504:bool)  [unwired: 1 in, 3 out]
        n1911 = case shown="真" w2504 {
          tunnel: w2505 -> [_ w2508]
          frame False {
          }
          frame True {
            n1912 = property class="Bool (严格)"(reference=w2508) -> ("BoolText.Text"=w2507:string)  [unwired: 1 in, 2 out]
            n1913 = property on="串口号" class="VISAName"() -> ("Value"=w2506:refnum<visa-resource-name>)  [unwired: 2 in, 2 out]
            n1914 = case shown="\"写参数\"" w2507 {
              tunnel: w2506 -> [_ w2511 w2540]
              frame "假", Default {
              }
              frame "读参数" {
                # "本机读取正确才读小信号"
                n1915 = flat-sequence {
                  tunnel: w2511 -> [w2513]
                  tunnel: [w2513] -> w2510
                  tunnel: [w2512] -> w2509
                  tunnel: w2510 -> [w2529]
                  tunnel: w2509 -> [w2528]
                  frame #0 {
                    n1916 = disable-structure shown="启用" {
                      disable-tunnel: w2513 -> [w2515 _]
                      disable-tunnel: [w2514 _] -> w2512
                      frame Enabled {
                        n1917 = call "读本机参数.vi"("串口号"=w2515) -> ("应答"=w2516:string)  [unwired: 2 in]
                        n1918 = case shown="\"读本机表\"" w2516 {
                          tunnel: [FALSE FALSE FALSE TRUE] -> w2514
                          frame "假", Default {
                          }
                          frame "超时" {
                            n1919 = property on="提示信息" class="Bool (严格)"("BoolText.Text"="读本机表参数超时！", "Val(Sgnl)"=TRUE ("提示信息")) -> ()  [unwired: 2 in, 2 out]
                          }
                          frame "错误" {
                            n1920 = property on="提示信息" class="Bool (严格)"("BoolText.Text"="读本机表参数错误！", "Val(Sgnl)"=TRUE ("提示信息")) -> ()  [unwired: 2 in, 2 out]
                          }
                          frame "读本机表" {
                            n1921 = global read "程序全局.vi" "本机表参数"() -> (w2527:cluster{"有功常数":i32, "无功常数":i32, "输出类型":i32})
                            n1922 = property on="本机表参数" class="Clust (严格)"("Value"=w2527) -> ()  [unwired: 2 in, 2 out]
                            n1923 = property on="提示信息" class="Bool (严格)"("BoolText.Text"="读本机表参数成功！", "Val(Sgnl)"=TRUE ("提示信息")) -> ()  [unwired: 2 in, 2 out]
                          }
                        }
                      }
                      frame Disabled {
                      }
                    }
                  }
                  frame #1 {
                    n1924 = case shown="真" w2528 {
                      tunnel: w2529 -> [_ w2531]
                      frame False {
                      }
                      frame True {
                        n1925 = call "读小信号变比.vi"("串口号"=w2531) -> ("应答"=w2530:string)  [unwired: 10 in]
                        n1926 = case shown="\"超时\"" w2530 {
                          frame "假", Default {
                          }
                          frame "超时" {
                            n1927 = property on="提示信息" class="Bool (严格)"("BoolText.Text"="读小信号超时！", "Val(Sgnl)"=TRUE ("提示信息")) -> ()  [unwired: 2 in, 2 out]
                          }
                          frame "错误" {
                            n1928 = property on="提示信息" class="Bool (严格)"("BoolText.Text"="读小信号错误！", "Val(Sgnl)"=TRUE ("提示信息")) -> ()  [unwired: 2 in, 2 out]
                          }
                          frame "读小信号" {
                            n1929 = global read "程序全局.vi" "小信号变比"() -> (w2538:cluster{"UB":sgl, "IB":sgl, "UC":sgl})
                            n1930 = local write "小信号变比(A/1mv)"(w2538) -> ()
                            n1931 = property on="提示信息" class="Bool (严格)"("BoolText.Text"="读小信号成功！", "Val(Sgnl)"=TRUE ("提示信息")) -> ()  [unwired: 2 in, 2 out]
                          }
                        }
                      }
                    }
                  }
                }
              }
              frame "写参数" {
                n1932 = local read "小信号变比(A/1mv)"() -> (w2539:cluster{"电流2":sgl, "电流3":sgl, "电流4":sgl})
                n1933 = property on="本机表参数" class="Clust (严格)"() -> ("Value"=w2546:cluster{"有功常数":i32, "无功常数":i32, "输出类型":i32})  [unwired: 2 in, 2 out]
                n1934 = call "设置本机表.vi"("本机表参数"=w2546, "串口号"=w2540) -> ("应答"=w2545:string)  [unwired: 3 in]
                n1935 = flat-sequence {
                  tunnel: w2545 -> [w2551]
                  tunnel: [w2551] -> w2542
                  tunnel: [w2548] -> w2541
                  tunnel: w2540 -> [w2550]
                  tunnel: w2539 -> [w2549]
                  tunnel: [w2553] -> w2544
                  tunnel: [w2552] -> w2543
                  tunnel: w2542 -> [w2554]
                  tunnel: w2541 -> [w2553]
                  tunnel: w2544 -> [w2565]
                  tunnel: w2543 -> [w2564]
                  frame #0 {
                    n1936 = call "临时信号变比.vi"("小信号变比"=w2549, "串口号"=w2550) -> ("应答"=w2548:string)  [unwired: 9 in]
                    n1937 = Wait (ms)(milliseconds to wait=10) -> ()  [unwired: 1 out]
                  }
                  frame #1 {
                    n1938 = case shown="\"正确\"" w2554 {
                      tunnel: [FALSE FALSE FALSE w2562] -> w2552
                      frame "假", Default {
                      }
                      frame "超时" {
                        n1939 = property on="提示信息" class="Bool (严格)"("BoolText.Text"="写入超时！", "Val(Sgnl)"=TRUE ("提示信息")) -> ()  [unwired: 2 in, 2 out]
                      }
                      frame "错误" {
                        n1940 = property on="提示信息" class="Bool (严格)"("BoolText.Text"="写入错误！", "Val(Sgnl)"=TRUE ("提示信息")) -> ()  [unwired: 2 in, 2 out]
                      }
                      frame "正确" {
                        w2562 = TRUE ("提示信息")
                        n1941 = property on="提示信息" class="Bool (严格)"("BoolText.Text"="写入成功！", "Val(Sgnl)"=w2562) -> ()  [unwired: 2 in, 2 out]
                      }
                    }
                  }
                  frame #2 {
                    n1942 = case shown="真" w2564 {
                      tunnel: w2565 -> [_ w2566]
                      frame False {
                      }
                      frame True {
                        n1943 = case shown="\"超时\"" w2566 {
                          frame "假", Default {
                          }
                          frame "超时" {
                            n1944 = property on="提示信息" class="Bool (严格)"("BoolText.Text"="小信号写入超时！", "Val(Sgnl)"=TRUE ("提示信息")) -> ()  [unwired: 2 in, 2 out]
                          }
                          frame "错误" {
                            n1945 = property on="提示信息" class="Bool (严格)"("BoolText.Text"="小信号写入错误！", "Val(Sgnl)"=TRUE ("提示信息")) -> ()  [unwired: 2 in, 2 out]
                          }
                          frame "正确" {
                            n1946 = property on="提示信息" class="Bool (严格)"("BoolText.Text"="小信号写入成功！", "Val(Sgnl)"=TRUE ("提示信息")) -> ()  [unwired: 2 in, 2 out]
                          }
                        }
                      }
                    }
                  }
                }
              }
            }
          }
        }
      }
      event "E检定参数.额定电压", "UI检定参数.额定电压": Value Change {
        n1947 = event-data() -> ("NewVal"=w2573:sgl)  [unwired: 1 in, 4 out]
        n1948 = property on="额定电压" class="DigNum (严格)"("Value"=w2573) -> ()  [unwired: 2 in, 2 out]
        n1949 = property on="额定电压" class="DigNum (严格)"("Value"=w2573) -> ()  [unwired: 2 in, 2 out]
        n1950 = property on="额定电压" class="DigNum (严格)"("Value"=w2573) -> ()  [unwired: 2 in, 2 out]
        n1951 = global write "程序全局.vi" "额定电压"(w2573) -> ()
      }
      event "E检定参数.标定电流", "UI检定参数.标定电流": Value Change {
        n1952 = event-data() -> ("NewVal"=w2574:sgl)  [unwired: 1 in, 4 out]
        n1953 = property on="标定电流" class="DigNum (严格)"("Value"=w2574) -> ()  [unwired: 2 in, 2 out]
        n1954 = property on="标定电流" class="DigNum (严格)"("Value"=w2574) -> ()  [unwired: 2 in, 2 out]
        n1955 = property on="标定电流" class="DigNum (严格)"("Value"=w2574) -> ()  [unwired: 2 in, 2 out]
        n1956 = global write "程序全局.vi" "标定电流"(w2574) -> ()
      }
      event "潜动起动.试验项目": Value Change {
        n1957 = event-data() -> ("NewVal"=w2575:u16)  [unwired: 1 in, 4 out]
        n1958 = case shown="1" w2575 {
          frame 0, Default {
            n1959 = property on="I检定点" class="DigNum (严格)"("DisabledEnum"=3) -> ()  [unwired: 2 in, 2 out]
            n1960 = property on="标定电流" class="DigNum (严格)"("DisabledEnum"=3) -> ()  [unwired: 2 in, 2 out]
            n1961 = property on="测试时间" class="DigNum (严格)"("Value"=20.0 ("值")) -> ()  [unwired: 2 in, 2 out]
          }
          frame 1 {
            # "n个脉冲的时间"
            # "得到脉冲频率"
            n1962 = property on="标定电流" class="DigNum (严格)"("DisabledEnum"=0) -> ()  [unwired: 2 in, 2 out]
            n1963 = property on="I检定点" class="DigNum (严格)"("DisabledEnum"=0) -> ()  [unwired: 2 in, 2 out]
            n1964 = property on="标定电流" class="DigNum (严格)"() -> ("Value"=w2592:sgl)  [unwired: 2 in, 2 out]
            n1965 = property on="I检定点" class="DigNum (严格)"() -> ("Value"=w2590:sgl)  [unwired: 2 in, 2 out]
            n1966 = property on="额定电压" class="DigNum (严格)"() -> ("Value"=w2595:sgl)  [unwired: 2 in, 2 out]
            n1967 = property on="U检定点" class="DigNum (严格)"() -> ("Value"=w2594:sgl)  [unwired: 2 in, 2 out]
            n1968 = property on="有功常数" class="DigNum (严格)"() -> ("Value"=w2587:i32)  [unwired: 2 in, 2 out]
            n1969 = Compound Arithmetic op=MULTIPLY(w2595, w2594, sgl 0.01 ("值")) -> (w2589:sgl)
            n1970 = Compound Arithmetic op=MULTIPLY(w2592, w2590, sgl 0.01 ("值")) -> (w2588:sgl)
            n1971 = Divide(x=w2587, y=3600000) -> (x/y=w2585:dbl)
            n1972 = Compound Arithmetic op=MULTIPLY(w2589, w2588, w2585) -> (w2584:dbl)
            n1973 = property on="脉冲数" class="DigNum (严格)"() -> ("Value"=w2582:u32)  [unwired: 2 in, 2 out]
            n1974 = Reciprocal(x=w2584) -> (1/x=w2583:dbl)
            n1975 = Multiply(x=w2583, y=w2582) -> (x*y=w2581:dbl)
            n1976 = Divide(x=w2581, y=60.0) -> (x/y=w2579:dbl)
            n1977 = property on="测试时间" class="DigNum (严格)"("Value"=w2579) -> ()  [unwired: 2 in, 2 out]
          }
        }
      }
      event "潜动起动.脉冲数": Value Change {
        n1978 = event-data() -> ()  [unwired: 1 in, 5 out]
        n1979 = property on="试验项目" class="Ring (严格)"() -> ("Value"=w2600:u16)  [unwired: 2 in, 2 out]
        n1980 = Equal?(x=w2600, y=u16 1) -> (x = y?=w2598:bool)
        n1981 = case shown="真" w2598 {
          frame False {
            n1982 = property on="I检定点" class="DigNum (严格)"("DisabledEnum"=3) -> ()  [unwired: 2 in, 2 out]
            n1983 = property on="标定电流" class="DigNum (严格)"("DisabledEnum"=3) -> ()  [unwired: 2 in, 2 out]
            n1984 = property on="测试时间" class="DigNum (严格)"("Value"=20.0 ("值")) -> ()  [unwired: 2 in, 2 out]
          }
          frame True {
            n1985 = property on="试验项目" class="Ring (严格)"("Val(Sgnl)"=u16 1 ("值(信号)")) -> ()  [unwired: 2 in, 2 out]
          }
        }
      }
      event "潜动起动.额定电压", "潜动起动.U检定点", "潜动起动.标定电流", "潜动起动.I检定点": Value Change {
        n1986 = event-data() -> ()  [unwired: 1 in, 5 out]
        n1987 = property on="标定电流" class="DigNum (严格)"() -> ("Value"=w2607:sgl)  [unwired: 2 in, 2 out]
        n1988 = property on="试验项目" class="Ring (严格)"() -> ("Value"=w2605:u16)  [unwired: 2 in, 2 out]
        n1989 = global write "程序全局.vi" "标定电流"(w2607) -> ()
        n1990 = property on="标定电流" class="DigNum (严格)"("Value"=w2607) -> ()  [unwired: 2 in, 2 out]
        n1991 = property on="标定电流" class="DigNum (严格)"("Value"=w2607) -> ()  [unwired: 2 in, 2 out]
        n1992 = case shown="1" w2605 {
          selector: w2605 -> [_ w2609]
          frame 0, Default {
            n1993 = property on="测试时间" class="DigNum (严格)"("Value"=20.0 ("值")) -> ()  [unwired: 2 in, 2 out]
          }
          frame 1 {
            n1994 = property on="试验项目" class="Ring (严格)"("Val(Sgnl)"=w2609) -> ()  [unwired: 2 in, 2 out]
          }
        }
        n1995 = property on="额定电压" class="DigNum (严格)"() -> ("Value"=w2606:sgl)  [unwired: 2 in, 2 out]
        n1996 = property on="额定电压" class="DigNum (严格)"("Value"=w2606) -> ()  [unwired: 2 in, 2 out]
        n1997 = property on="额定电压" class="DigNum (严格)"("Value"=w2606) -> ()  [unwired: 2 in, 2 out]
        n1998 = global write "程序全局.vi" "额定电压"(w2606) -> ()
      }
      event "潜动起动.开始试验": Value Change {
        n1999 = event-data() -> ("NewVal"=w2611:bool)  [unwired: 1 in, 4 out]
        n2000 = property on="试验项目" class="Ring (严格)"() -> ("Value"=w2610:u16)  [unwired: 2 in, 2 out]
        n2001 = case shown="真" w2611 {
          tunnel: w2610 -> [_ w2616]
          frame False {
            n2002 = property on="控制选项卡" class="TabCtl (严格)"("PageSelVis"=TRUE ("页选择器可见")) -> ()  [unwired: 2 in, 2 out]
            n2003 = property on="计时状态" class="Bool (严格)"("Value"=FALSE ("检定状态")) -> ()  [unwired: 2 in, 2 out]
          }
          frame True {
            n2004 = flat-sequence {
              tunnel: w2616 -> [w2621]
              tunnel: [w2621] -> w2615
              tunnel: [w2620] -> w2614
              tunnel: w2615 -> [w2627]
              tunnel: w2614 -> [w2626]
              frame #0 {
                n2005 = property on="潜启电流通道" class="Ring (严格)"() -> ("Value"=w2619:u16)  [unwired: 2 in, 2 out]
                n2006 = property on="串口号" class="VISAName"() -> ("Value"=w2620:refnum<visa-resource-name>)  [unwired: 2 in, 2 out]
                n2007 = call "小信号配置.vi"("电流通道"=w2619, "串口号"=w2620) -> ("应答"=w2618:string)  [unwired: 9 in]
                n2008 = case shown="\"正确\"" w2618 {
                  frame "错误", Default {
                    n2009 = property on="提示信息" class="Bool (严格)"("BoolText.Text"="小信号设置出错！", "Val(Sgnl)"=TRUE ("提示信息")) -> ()  [unwired: 2 in, 2 out]
                  }
                  frame "正确" {
                  }
                }
                n2010 = Wait (ms)(milliseconds to wait=u32 10 ("等待时间（毫秒）")) -> ()  [unwired: 1 out]
              }
              frame #1 {
                n2011 = case shown="1" w2627 {
                  tunnel: w2626 -> [_ w2678]
                  frame 0, Default {
                    w2631 = sgl 0.0 ("电流幅值")
                    w2638 = u32 85 ("电流档位")
                    w2630 = sgl 0.0 ("电压纹波")
                    n2012 = property on="串口号" class="VISAName"() -> ("Value"=w2629:refnum<visa-resource-name>)  [unwired: 2 in, 2 out]
                    n2013 = property on="U检定点" class="DigNum (严格)"() -> ("Value"=w2636:sgl)  [unwired: 2 in, 2 out]
                    n2014 = property on="额定电压" class="DigNum (严格)"() -> ("Value"=w2634:sgl)  [unwired: 2 in, 2 out]
                    n2015 = Multiply(x=w2636, y=sgl 0.01 ("电压纹波")) -> (x*y=w2635:sgl)
                    n2016 = Multiply(x=w2635, y=w2634) -> (x*y=w2633:sgl)
                    n2017 = call "高精度写.vi"("电压幅值"=w2633, "电压纹波"=w2630, "串口号"=w2629, "电压档位"=w2638, "电流幅值"=w2631, "电流档位值"=w2638, "纹波频率"=w2630, "电流纹波"=w2630) -> ("应答"=w2628:string)  [unwired: 7 in]
                    n2018 = Wait (ms)(milliseconds to wait=u32 100 ("等待时间（毫秒）")) -> ()  [unwired: 1 out]
                    n2019 = case shown="\"正确\"" w2628 {
                      tunnel: w2629 -> [_ _ w2643]
                      tunnel: w2633 -> [_ _ w2647]
                      tunnel: w2631 -> [_ _ w2646]
                      frame "错误", Default {
                        n2020 = property on="提示信息" class="Bool (严格)"("BoolText.Text"="高精度写错误！", "Val(Sgnl)"=TRUE ("提示信息")) -> ()  [unwired: 2 in, 2 out]
                      }
                      frame "超时" {
                        n2021 = property on="提示信息" class="Bool (严格)"("BoolText.Text"="高精度写超时！", "Val(Sgnl)"=TRUE ("提示信息")) -> ()  [unwired: 2 in, 2 out]
                      }
                      frame "正确" {
                        n2022 = call "电能清零.vi"("串口号"=w2643) -> ("应答"=w2644:string)  [unwired: 2 in]
                        n2023 = Wait (ms)(milliseconds to wait=u32 100 ("等待时间（毫秒）")) -> ()  [unwired: 1 out]
                        n2024 = case shown="\"正确\"" w2644 {
                          tunnel: w2643 -> [_ w2651]
                          tunnel: w2647 -> [_ w2653]
                          tunnel: w2646 -> [_ w2652]
                          frame "错误", Default {
                            n2025 = property on="提示信息" class="Bool (严格)"("BoolText.Text"="电能清零错误！", "Val(Sgnl)"=TRUE ("提示信息")) -> ()  [unwired: 2 in, 2 out]
                          }
                          frame "正确" {
                            w2655 = u16 0 items=["电压启动", "电流启动", "全部启动"] ("启动项")
                            n2026 = Wait (ms)(milliseconds to wait=u32 100 ("等待时间（毫秒）")) -> ()  [unwired: 1 out]
                            n2027 = call "输出启动.vi"("启动项"=w2655, "串口号"=w2651) -> ("应答"=w2650:string)  [unwired: 3 in]
                            n2028 = case shown="\"正确\"" w2650 {
                              tunnel: w2653 -> [_ w2659]
                              tunnel: w2652 -> [_ w2658]
                              frame "错误", Default {
                                n2029 = property on="提示信息" class="Bool (严格)"("BoolText.Text"="起动输出错误！", "Val(Sgnl)"=TRUE ("提示信息")) -> ()  [unwired: 2 in, 2 out]
                              }
                              frame "正确" {
                                n2030 = property on="本机表格" class="Tbl (严格)"() -> ("Value"=w2660:string[][])  [unwired: 2 in, 2 out]
                                n2031 = Number To Fractional String(number=w2659, precision (6)=i16 3 ("精度(6)")) -> (F-format string=w2667:string)  [unwired: 2 in]
                                n2032 = Number To Fractional String(number=w2658, precision (6)=i16 3 ("精度(6)")) -> (F-format string=w2669:string)  [unwired: 2 in]
                                n2033 = Index Array(array=w2660, index (col)=0 ("禁用的索引 (列)")) -> (element=w2662:string[])  [unwired: 1 in]
                                n2034 = Replace Array Subset(array=w2662, new element=w2667, index=0 ("索引")) -> (w2665:string[])
                                n2035 = Replace Array Subset(array=w2665, new element=w2669, index=1 ("索引")) -> (w2672:string[])
                                n2036 = property on="计时状态" class="Bool (严格)"("Value"=TRUE ("计时状态")) -> ()  [unwired: 2 in, 2 out]
                                n2037 = Replace Array Subset(array=w2660, new element=w2672, index (col)=0 ("禁用的索引 (列)")) -> (w2671:string[][])  [unwired: 1 in]
                                n2038 = property on="本机表格" class="Tbl (严格)"("Value"=w2671) -> ()  [unwired: 2 in, 2 out]
                              }
                            }
                          }
                        }
                      }
                    }
                  }
                  frame 1 {
                    w2684 = sgl 0.01 ("电压纹波")
                    w2689 = u32 85 ("电流档位")
                    w2680 = sgl 0.0 ("电压纹波")
                    n2039 = property on="U检定点" class="DigNum (严格)"() -> ("Value"=w2688:sgl)  [unwired: 2 in, 2 out]
                    n2040 = property on="额定电压" class="DigNum (严格)"() -> ("Value"=w2686:sgl)  [unwired: 2 in, 2 out]
                    n2041 = property on="I检定点" class="DigNum (严格)"() -> ("Value"=w2683:sgl)  [unwired: 2 in, 2 out]
                    n2042 = property on="标定电流" class="DigNum (严格)"() -> ("Value"=w2681:sgl)  [unwired: 2 in, 2 out]
                    n2043 = property on="潜启电流通道" class="Ring (严格)"() -> ("Value"=w2674:u16)  [unwired: 2 in, 2 out]
                    n2044 = Multiply(x=w2684, y=w2683) -> (x*y=w2682:sgl)
                    n2045 = Multiply(x=w2688, y=w2684) -> (x*y=w2687:sgl)
                    n2046 = Multiply(x=w2687, y=w2686) -> (x*y=w2685:sgl)
                    n2047 = Multiply(x=w2682, y=w2681) -> (x*y=w2677:sgl)
                    n2048 = case shown="1" w2674 {
                      tunnel: w2677 -> [w2690 w2692 w2698 w2704]
                      tunnel: [w2690 w2691 w2697 w2703] -> w2676
                      frame 0, Default {
                      }
                      frame 1 {
                        n2049 = property on="小信号变比(A/1mv)" class="Clust (严格)"() -> ("Value"=w2696:cluster{"电流2":sgl, "电流3":sgl, "电流4":sgl})  [unwired: 2 in, 2 out]
                        n2050 = Unbundle(w2696) -> ("电流2"=w2694:sgl)  [unwired: 2 out]
                        n2051 = Multiply(x=w2694, y=1000.0) -> (x*y=w2693:dbl)
                        n2052 = Divide(x=w2692, y=w2693) -> (x/y=w2691:dbl)
                      }
                      frame 2 {
                        n2053 = property on="小信号变比(A/1mv)" class="Clust (严格)"() -> ("Value"=w2702:cluster{"电流2":sgl, "电流3":sgl, "电流4":sgl})  [unwired: 2 in, 2 out]
                        n2054 = Unbundle(w2702) -> ("电流3"=w2700:sgl)  [unwired: 2 out]
                        n2055 = Multiply(x=w2700, y=1000.0) -> (x*y=w2699:dbl)
                        n2056 = Divide(x=w2698, y=w2699) -> (x/y=w2697:dbl)
                      }
                      frame 3 {
                        n2057 = property on="小信号变比(A/1mv)" class="Clust (严格)"() -> ("Value"=w2708:cluster{"电流2":sgl, "电流3":sgl, "电流4":sgl})  [unwired: 2 in, 2 out]
                        n2058 = Unbundle(w2708) -> ("电流4"=w2706:sgl)  [unwired: 2 out]
                        n2059 = Multiply(x=w2706, y=1000.0) -> (x*y=w2705:dbl)
                        n2060 = Divide(x=w2704, y=w2705) -> (x/y=w2703:dbl)
                      }
                    }
                    n2061 = call "高精度写.vi"("电压幅值"=w2685, "电压纹波"=w2680, "串口号"=w2678, "电压档位"=w2689, "电流幅值"=w2676, "电流档位值"=w2689, "纹波频率"=w2680, "电流纹波"=w2680, "电流通道"=w2674) -> ("应答"=w2679:string)  [unwired: 6 in]
                    n2062 = Wait (ms)(milliseconds to wait=u32 100 ("等待时间（毫秒）")) -> ()  [unwired: 1 out]
                    n2063 = case shown="\"正确\"" w2679 {
                      tunnel: w2678 -> [_ _ w2714]
                      tunnel: w2685 -> [_ _ w2717]
                      tunnel: w2677 -> [_ _ w2716]
                      frame "错误", Default {
                        n2064 = property on="提示信息" class="Bool (严格)"("BoolText.Text"="高精度写错误！", "Val(Sgnl)"=TRUE ("提示信息")) -> ()  [unwired: 2 in, 2 out]
                      }
                      frame "超时" {
                        n2065 = property on="提示信息" class="Bool (严格)"("BoolText.Text"="高精度写超时！", "Val(Sgnl)"=TRUE ("提示信息")) -> ()  [unwired: 2 in, 2 out]
                      }
                      frame "正确" {
                        n2066 = call "电能清零.vi"("串口号"=w2714) -> ("应答"=w2713:string)  [unwired: 2 in]
                        n2067 = Wait (ms)(milliseconds to wait=u32 50 ("等待时间（毫秒）")) -> ()  [unwired: 1 out]
                        n2068 = case shown="\"正确\"" w2713 {
                          tunnel: w2714 -> [_ w2721]
                          tunnel: w2717 -> [_ w2724]
                          tunnel: w2716 -> [_ w2723]
                          frame "错误", Default {
                            n2069 = property on="提示信息" class="Bool (严格)"("BoolText.Text"="电能清零错误！", "Val(Sgnl)"=TRUE ("提示信息")) -> ()  [unwired: 2 in, 2 out]
                          }
                          frame "正确" {
                            w2726 = u16 2 items=["电压启动", "电流启动", "全部启动"] ("启动项")
                            n2070 = property on="潜启电流通道" class="Ring (严格)"() -> ("Value"=w2720:u16)  [unwired: 2 in, 2 out]
                            n2071 = call "输出启动.vi"("电流通道"=w2720, "启动项"=w2726, "串口号"=w2721) -> ("应答"=w2722:string)  [unwired: 2 in]
                            n2072 = Wait (ms)(milliseconds to wait=u32 100 ("等待时间（毫秒）")) -> ()  [unwired: 1 out]
                            n2073 = case shown="\"正确\"" w2722 {
                              tunnel: w2724 -> [_ w2730]
                              tunnel: w2723 -> [_ w2729]
                              frame "错误", Default {
                                n2074 = property on="提示信息" class="Bool (严格)"("BoolText.Text"="起动输出错误！", "Val(Sgnl)"=TRUE ("提示信息")) -> ()  [unwired: 2 in, 2 out]
                              }
                              frame "正确" {
                                n2075 = property on="本机表格" class="Tbl (严格)"() -> ("Value"=w2731:string[][])  [unwired: 2 in, 2 out]
                                n2076 = Number To Fractional String(number=w2730, precision (6)=i16 3 ("精度(6)")) -> (F-format string=w2738:string)  [unwired: 2 in]
                                n2077 = Number To Fractional String(number=w2729, precision (6)=i16 3 ("精度(6)")) -> (F-format string=w2740:string)  [unwired: 2 in]
                                n2078 = Index Array(array=w2731, index (col)=0 ("禁用的索引 (列)")) -> (element=w2733:string[])  [unwired: 1 in]
                                n2079 = Replace Array Subset(array=w2733, new element=w2738, index=0 ("索引")) -> (w2736:string[])
                                n2080 = Replace Array Subset(array=w2736, new element=w2740, index=1 ("索引")) -> (w2743:string[])
                                n2081 = property on="计时状态" class="Bool (严格)"("Value"=TRUE ("计时状态")) -> ()  [unwired: 2 in, 2 out]
                                n2082 = Replace Array Subset(array=w2731, new element=w2743, index (col)=0 ("禁用的索引 (列)")) -> (w2742:string[][])  [unwired: 1 in]
                                n2083 = property on="本机表格" class="Tbl (严格)"("Value"=w2742) -> ()  [unwired: 2 in, 2 out]
                              }
                            }
                          }
                        }
                      }
                    }
                  }
                }
                n2084 = property on="控制选项卡" class="TabCtl (严格)"("PageSelVis"=FALSE ("页选择器可见")) -> ()  [unwired: 2 in, 2 out]
                n2085 = property on="试验结果" class="Arr (严格)"("Value"=string[] [" ", "", " "] ("试验结果")) -> ()  [unwired: 2 in, 2 out]
              }
            }
          }
        }
      }
      event "报表选项": Value Change {
        n2086 = event-data() -> ("NewVal"=w2745:u16)  [unwired: 1 in, 4 out]
        n2087 = case shown="0, 默认" w2745 {
          frame 0, Default {
            n2088 = Get Date/Time In Seconds() -> (seconds since 1Jan1904=w2752:timestamp)
            n2089 = property on="报表名称" class="Str"("DisabledEnum"=3) -> ()  [unwired: 2 in, 2 out]
            n2090 = Format Date/Time String(time format string (%c)="%Y%m%d-" ("时间格式字符串(%c)"), seconds (now)=w2752) -> (date/time string=w2749:string)  [unwired: 1 in]
            n2091 = Format Date/Time String(time format string (%c)="%H-%M-%S" ("时间格式字符串(%c)"), seconds (now)=w2752) -> (date/time string=w2748:string)  [unwired: 1 in]
            n2092 = Concatenate Strings(w2749, w2748) -> (w2747:string)
            n2093 = property on="报表名称" class="Str"("Value"=w2747) -> ()  [unwired: 2 in, 2 out]
          }
          frame 1 {
            n2094 = property on="报表名称" class="Str"("DisabledEnum"=0) -> ()  [unwired: 2 in, 2 out]
          }
        }
      }
      event "生成报表": Value Change {
        n2095 = event-data() -> ("NewVal"=w2754:bool)  [unwired: 1 in, 4 out]
        n2096 = case shown="真" w2754 {
          frame False {
          }
          frame True {
            n2097 = property on="电能显示表" class="Tbl (严格)"() -> ("Visible"=w2755:bool)  [unwired: 2 in, 2 out]
            n2098 = property on="误差显示表" class="Tbl (严格)"() -> ("Visible"=w2758:bool)  [unwired: 2 in, 2 out]
            n2099 = case shown="假" w2758 {
              tunnel: w2755 -> [w2759 _]
              frame False {
                n2100 = case shown="真" w2759 {
                  frame False {
                    n2101 = property on="单点显示表" class="Tbl (严格)"() -> ("Value"=w2773:string[][])  [unwired: 2 in, 2 out]
                    n2102 = property on="单点显示表" class="Tbl (严格)"() -> ("Row Headers[]"=w2771:string[])  [unwired: 2 in, 2 out]
                    n2103 = property on="单点显示表" class="Tbl (严格)"() -> ("Column Headers[]"=w2770:string[])  [unwired: 2 in, 2 out]
                    n2104 = Insert Into Array(array=w2770, index=0 ("索引"), new element="") -> (w2766:string[])
                    n2105 = Insert Into Array(array=w2773, index (col)=0 ("禁用的索引 (列)"), new element=w2771) -> (w2767:string[][])  [unwired: 1 in]
                    n2106 = Insert Into Array(array=w2767, index (row)=0 ("索引 (行)"), new element=w2766) -> (w2764:string[][])  [unwired: 1 in]
                    n2107 = property on="报表名称" class="Str"() -> ("Value"=w2763:string)  [unwired: 2 in, 2 out]
                    n2108 = Concatenate Strings(".\\" ("字符串"), w2763, ".xls" ("字符串")) -> (w2760:string)
                    n2109 = Build Path(base path=path "D:/report" ("基路径"), name or relative path=w2760) -> (appended path=w2774:path)
                    n2110 = call-poly <vilib>:"Write To Spreadsheet File.vi"("2D data"=w2764, "file path (dialog if empty)"=w2774) -> ()  [unwired: 6 in, 1 out]
                  }
                  frame True {
                    n2111 = property on="电能显示表" class="Tbl (严格)"() -> ("Value"=w2791:string[][])  [unwired: 2 in, 2 out]
                    n2112 = property on="电能显示表" class="Tbl (严格)"() -> ("Row Headers[]"=w2789:string[])  [unwired: 2 in, 2 out]
                    n2113 = property on="电能显示表" class="Tbl (严格)"() -> ("Column Headers[]"=w2788:string[])  [unwired: 2 in, 2 out]
                    n2114 = Insert Into Array(array=w2788, index=0 ("索引"), new element="") -> (w2784:string[])
                    n2115 = Insert Into Array(array=w2791, index (col)=0 ("禁用的索引 (列)"), new element=w2789) -> (w2785:string[][])  [unwired: 1 in]
                    n2116 = Insert Into Array(array=w2785, index (row)=0 ("索引 (行)"), new element=w2784) -> (w2782:string[][])  [unwired: 1 in]
                    n2117 = property on="报表名称" class="Str"() -> ("Value"=w2780:string)  [unwired: 2 in, 2 out]
                    n2118 = Concatenate Strings(".\\" ("字符串"), w2780, ".xls" ("字符串")) -> (w2777:string)
                    n2119 = Build Path(base path=path "D:/report" ("基路径"), name or relative path=w2777) -> (appended path=w2776:path)
                    n2120 = call-poly <vilib>:"Write To Spreadsheet File.vi"("2D data"=w2782, "file path (dialog if empty)"=w2776) -> ()  [unwired: 6 in, 1 out]
                  }
                }
              }
              frame True {
                n2121 = property on="误差显示表" class="Tbl (严格)"() -> ("Value"=w2807:string[][])  [unwired: 2 in, 2 out]
                n2122 = property on="误差显示表" class="Tbl (严格)"() -> ("Row Headers[]"=w2805:string[])  [unwired: 2 in, 2 out]
                n2123 = property on="误差显示表" class="Tbl (严格)"() -> ("Column Headers[]"=w2804:string[])  [unwired: 2 in, 2 out]
                n2124 = Insert Into Array(array=w2804, index=0 ("索引"), new element="") -> (w2800:string[])
                n2125 = Insert Into Array(array=w2807, index (col)=0 ("禁用的索引 (列)"), new element=w2805) -> (w2801:string[][])  [unwired: 1 in]
                n2126 = Insert Into Array(array=w2801, index (row)=0 ("索引 (行)"), new element=w2800) -> (w2798:string[][])  [unwired: 1 in]
                n2127 = property on="报表名称" class="Str"() -> ("Value"=w2796:string)  [unwired: 2 in, 2 out]
                n2128 = Concatenate Strings(".\\" ("字符串"), w2796, ".xls" ("字符串")) -> (w2793:string)
                n2129 = Build Path(base path=path "D:/report" ("基路径"), name or relative path=w2793) -> (appended path=w2792:path)
                n2130 = call-poly <vilib>:"Write To Spreadsheet File.vi"("2D data"=w2798, "file path (dialog if empty)"=w2792) -> ()  [unwired: 6 in, 1 out]
              }
            }
            n2131 = property on="提示信息" class="Bool (严格)"("BoolText.Text"="报表已保存在D:/report目录下！", "Val(Sgnl)"=TRUE ("提示信息")) -> ()  [unwired: 2 in, 2 out]
          }
        }
      }
      event Panel Close? {
        n2132 = event-data() -> ()  [unwired: 1 in, 3 out]
        n2133 = local read "串口信息"() -> (w2812:T14)
        n2134 = Unbundle By Name(w2812) -> ("串口号"=w2811:refnum<visa-resource-name>)
        n2135 = global write "系统全局.vi" "退出程序"(TRUE ("退出程序")) -> ()
        n2136 = Wait (ms)(milliseconds to wait=u32 500 ("等待时间（毫秒）")) -> ()  [unwired: 1 out]
        n2137 = VISA Close(VISA resource name=w2811) -> ()  [unwired: 1 in, 1 out]
        n2138 = event-data("Discard?"=FALSE) -> ()  [unwired: 1 in, 1 out]
      }
    }
    n2139 = Wait (ms)(milliseconds to wait=u32 50 ("等待时间（毫秒）")) -> ()  [unwired: 1 out]
    n2140 = global read "系统全局.vi" "退出程序"() -> (w907:bool)
  }
  n2141 = disable-structure "潜动启动" shown="启用" {
    frame Disabled {
    }
    frame Enabled {
    }
  }
  n2142 = disable-structure "误差计算" shown="启用" {
    frame Enabled {
    }
    frame Disabled {
    }
  }
  n2143 = property on="result_Tab" class="TabCtl (严格)"("Visible"=TRUE) -> ()  [unwired: 2 in, 2 out]
  n2144 = disable-structure shown="禁用" {
    frame Disabled {
      n2145 = property on="U状态" class="Bool (严格)"("Value"=TRUE ("输出状态")) -> ()  [unwired: 2 in, 2 out]
      n2146 = property on="I状态" class="Bool (严格)"("Value"=TRUE ("输出状态")) -> ()  [unwired: 2 in, 2 out]
    }
    frame Enabled {
    }
  }
  n2147 = Wait (ms)(milliseconds to wait=u32 50 ("等待时间（毫秒）")) -> ()  [unwired: 1 out]
